vi "CRYLimits Editor.vi"(6 "Channel":i32=1, 8 "Calibration In":string, 9 "Hardware In":string, 10 "Set up in":string) -> (2 "Set up Out":string)   [LabVIEW 2013]
uses:
  <vilib>/Utility/miscctls.llb/LVBoundsTypeDef.ctl
  Typedef Control/CRYLimits.ctl
  Typedef Control/CRYWaveform Cluster.ctl
  Typedef Control/CRYData Cluster.ctl
  <vilib>/Utility/miscctls.llb/LVRowAndColumnTypeDef.ctl
  <vilib>/Utility/miscctls.llb/LVRowAndColumnUnsignedTypeDef.ctl
  CRYLimit edit global.vi
  CRYProject/CRYProject Editor Global.vi
  CRYWindow/SubVI/CRYMain Sub Window Global.vi
  CRYMainGlobal.vi
  CRYStepSetup/CRYStepSetup Global.vi
panel:
  in  "RawLo Limit":dbl caption="酒贰茄拌" format="%.2p"
  in  "RawUp Limit":dbl caption="眶茄拌" format="%.2p"
  out "Limit Cluster Bk":T1={"Name"="", "Tolerance"=2, "X Axis"=1, "Limits"=2, "Upper Limit"=[{100.0, 1.0}, {1000.0, 1.0}], "Align Ref"={1000.0, 0.0}, "Lower Limit"=[{100.0, -1.0}, {1000.0, -1.0}], "Y data"=1, "Y unit"="(und)", "Y dB ref"=1.0, "Curve Names"=[], "Y-Resolution"=1, "Type"=1, "x float"=FALSE, "X min-max-step"={"Limit X Offset Min"=0.9, "Limit X Offset Max"=1.1, "Limit X Offset Step Size"=1.01}, "magn/phase"=1, "Upper Limit Type"=0, "Lower Limit Type"=0, "Lim Curve axis up"=1, "Lim Curve axis lo"=1, "Data Selection Upper"=1, "Data Selection Lower"=1, "X-Resolution"=1, "Output failed point curves?"=FALSE, "X data"=1, "X unit"="(und)", "X dB ref"=1.0, "X-Y Graph Set-up"="", "Tab Value"=enum."Parameters", "Help"="", "X Up Val"=0.0, "Y Up Val"=0.0, "X Low Val"=0.0, "Y Low Val"=0.0, "Up Limit Val"=0.0, "Low Limit Val"=0.0, "bAdd DataName"=FALSE, "Custom Name"=""} {"X data" items=["dB", "Lin"]; "Data Selection Lower" items=["Single Values", "Curves", "Waveforms"]; "Data Selection Upper" items=["Single Values", "Curves", "Waveforms"]; "Lim Curve axis lo" items=["x", "y", "z"]; "Lim Curve axis up" items=["x", "y", "z"]; "Lower Limit Type" items=["User Defined", "Memory List"]; "Upper Limit Type" items=["User Defined", "Memory List"]; "Type" items=["Single Value", "Curve", "Waveforms", "Voltmeter"]; "Y data" items=["dB", "Lin"]; "Limits" items=["Upper Only", "Lower Only", "Upper & Lower"]; "X Axis" items=["Linear", "Logarithmic"]; "Tolerance" items=["Individual Points", "Absolute Limits", "Floating Limits", "Floating Data", "Aligned Limits", "Aligned Data"]}
  out "Raw DataVal":dbl format="%.2p"
  in  "CurLibChange":bool caption="Add Lib"
  out "MinMaxXrange":bool
  out "Lo_oldx":dbl
  out "Up_oldx":dbl
  out "cursor move":bool
  out "Wave":T2={"Waveform"={"X0"=0.0, "dX"=0.0, "Y"=[]}, "X data"=1, "Y data"=1, "Y axis"=1, "X unit"="s", "Y unit"="V", "Y dB ref"=1.0, "display Y"=TRUE, "display X"=TRUE, "Overload?"=FALSE, "Test Info"="", "Step No."=0, "Name"="", "protected"=FALSE, "Sqc history"=[], "Signal Channel ID"=0, "Plot Settings"={"Color"=0, "Interpolation"=0, "Point Style"=0, "Line Style"=0, "Point Color"=0, "Line Width"=0, "Bar Plot Style"=0, "Fill To"=0}, "AutoProtect"=FALSE} {"Y dB ref" format="%.1f"; "Y axis" items=["Log", "Lin"]; "Y data" items=["dB", "Lin"]; "X data" items=["dB", "Lin"]}
  out "EndFlag":bool
  in  "Add Lib":bool
  in  "AddStep":bool
  in  "Load state":bool
  out "Lo Curve and Values":T3={"Name"="", "Curve"=[], "X data"=1, "Y data"=1, "Z data"=1, "X axis"=0, "Y axis"=1, "Z axis"=1, "X unit"="Hz", "Y unit"="", "Z unit"="deg.", "X dB ref"=1.0, "Y dB ref"=1.0, "Z dB ref"=1.0, "single val"=FALSE, "protected"=FALSE, "display X"=TRUE, "display Y"=TRUE, "display Z"=TRUE, "Test Info"="", "Step No."=0, "Plot Settings"={"Color"=0, "Interpolation"=0, "Point Style"=0, "Line Style"=0, "Point Color"=0, "Line Width"=0, "Bar Plot Style"=0, "Fill To"=0}, "AutoProtect"=FALSE} {"Z data" items=["dB", "Lin"]; "X data" items=["dB", "Lin"]; "Y data" items=["dB", "Lin"]; "Z dB ref" format="%.1f"; "Z axis" items=["Log", "Lin"]; "X dB ref" format="%.1f"; "X axis" items=["Log", "Lin"]; "Y axis" items=["Log", "Lin"]; "Y dB ref" format="%.1f"; "Curve"."z" format="%.2f"; "Curve"."y" format="%.2f"; "Curve"."x" format="%.2f"}
  out "Up Curve and Value":T3={"Name"="", "Curve"=[], "X data"=1, "Y data"=1, "Z data"=1, "X axis"=0, "Y axis"=1, "Z axis"=1, "X unit"="Hz", "Y unit"="", "Z unit"="deg.", "X dB ref"=1.0, "Y dB ref"=1.0, "Z dB ref"=1.0, "single val"=FALSE, "protected"=FALSE, "display X"=TRUE, "display Y"=TRUE, "display Z"=TRUE, "Test Info"="", "Step No."=0, "Plot Settings"={"Color"=0, "Interpolation"=0, "Point Style"=0, "Line Style"=0, "Point Color"=0, "Line Width"=0, "Bar Plot Style"=0, "Fill To"=0}, "AutoProtect"=FALSE} {"Z data" items=["dB", "Lin"]; "X data" items=["dB", "Lin"]; "Y data" items=["dB", "Lin"]; "Z dB ref" format="%.1f"; "Z axis" items=["Log", "Lin"]; "X dB ref" format="%.1f"; "X axis" items=["Log", "Lin"]; "Y axis" items=["Log", "Lin"]; "Y dB ref" format="%.1f"; "Curve"."z" format="%.2f"; "Curve"."y" format="%.2f"; "Curve"."x" format="%.2f"}
  out "Curve and Value":T3={"Name"="", "Curve"=[], "X data"=1, "Y data"=1, "Z data"=1, "X axis"=0, "Y axis"=1, "Z axis"=1, "X unit"="Hz", "Y unit"="", "Z unit"="deg.", "X dB ref"=1.0, "Y dB ref"=1.0, "Z dB ref"=1.0, "single val"=FALSE, "protected"=FALSE, "display X"=TRUE, "display Y"=TRUE, "display Z"=TRUE, "Test Info"="", "Step No."=0, "Plot Settings"={"Color"=0, "Interpolation"=0, "Point Style"=0, "Line Style"=0, "Point Color"=0, "Line Width"=0, "Bar Plot Style"=0, "Fill To"=0}, "AutoProtect"=FALSE} {"Z data" items=["dB", "Lin"]; "X data" items=["dB", "Lin"]; "Y data" items=["dB", "Lin"]; "Z dB ref" format="%.1f"; "Z axis" items=["Log", "Lin"]; "X dB ref" format="%.1f"; "X axis" items=["Log", "Lin"]; "Y axis" items=["Log", "Lin"]; "Y dB ref" format="%.1f"; "Curve"."z" format="%.2f"; "Curve"."y" format="%.2f"; "Curve"."x" format="%.2f"}
  in  "Plot Multilimit":bool
  out "Lo Wave":T2={"Waveform"={"X0"=0.0, "dX"=0.0, "Y"=[]}, "X data"=1, "Y data"=1, "Y axis"=1, "X unit"="s", "Y unit"="V", "Y dB ref"=1.0, "display Y"=TRUE, "display X"=TRUE, "Overload?"=FALSE, "Test Info"="", "Step No."=0, "Name"="", "protected"=FALSE, "Sqc history"=[], "Signal Channel ID"=0, "Plot Settings"={"Color"=0, "Interpolation"=0, "Point Style"=0, "Line Style"=0, "Point Color"=0, "Line Width"=0, "Bar Plot Style"=0, "Fill To"=0}, "AutoProtect"=FALSE} {"Y dB ref" format="%.1f"; "Y axis" items=["Log", "Lin"]; "Y data" items=["dB", "Lin"]; "X data" items=["dB", "Lin"]}
  out "Up Wave":T2={"Waveform"={"X0"=0.0, "dX"=0.0, "Y"=[]}, "X data"=1, "Y data"=1, "Y axis"=1, "X unit"="s", "Y unit"="V", "Y dB ref"=1.0, "display Y"=TRUE, "display X"=TRUE, "Overload?"=FALSE, "Test Info"="", "Step No."=0, "Name"="", "protected"=FALSE, "Sqc history"=[], "Signal Channel ID"=0, "Plot Settings"={"Color"=0, "Interpolation"=0, "Point Style"=0, "Line Style"=0, "Point Color"=0, "Line Width"=0, "Bar Plot Style"=0, "Fill To"=0}, "AutoProtect"=FALSE} {"Y dB ref" format="%.1f"; "Y axis" items=["Log", "Lin"]; "Y data" items=["dB", "Lin"]; "X data" items=["dB", "Lin"]}
  out "Lo Limit Data":cluster{"x":dbl, "y":dbl}[](array[cluster])
  out "Up Limit Data":cluster{"x":dbl, "y":dbl}[](array[cluster])
  in  "Plot graphs":bool
  out "Limit Cluster":T1={"Name"="", "Tolerance"=2, "X Axis"=1, "Limits"=2, "Upper Limit"=[{100.0, 1.0}, {1000.0, 1.0}], "Align Ref"={1000.0, 0.0}, "Lower Limit"=[{100.0, -1.0}, {1000.0, -1.0}], "Y data"=1, "Y unit"="(und)", "Y dB ref"=1.0, "Curve Names"=[], "Y-Resolution"=1, "Type"=1, "x float"=FALSE, "X min-max-step"={"Limit X Offset Min"=0.9, "Limit X Offset Max"=1.1, "Limit X Offset Step Size"=1.01}, "magn/phase"=1, "Upper Limit Type"=0, "Lower Limit Type"=0, "Lim Curve axis up"=1, "Lim Curve axis lo"=1, "Data Selection Upper"=1, "Data Selection Lower"=1, "X-Resolution"=1, "Output failed point curves?"=FALSE, "X data"=1, "X unit"="(und)", "X dB ref"=1.0, "X-Y Graph Set-up"="", "Tab Value"=enum."Parameters", "Help"="", "X Up Val"=0.0, "Y Up Val"=0.0, "X Low Val"=0.0, "Y Low Val"=0.0, "Up Limit Val"=0.0, "Low Limit Val"=0.0, "bAdd DataName"=FALSE, "Custom Name"=""} {"X data" items=["dB", "Lin"]; "Data Selection Lower" items=["Single Values", "Curves", "Waveforms"]; "Data Selection Upper" items=["Single Values", "Curves", "Waveforms"]; "Lim Curve axis lo" items=["x", "y", "z"]; "Lim Curve axis up" items=["x", "y", "z"]; "Lower Limit Type" items=["User Defined", "Memory List"]; "Upper Limit Type" items=["User Defined", "Memory List"]; "Type" items=["Single Value", "Curve", "Waveforms", "Voltmeter"]; "Y data" items=["dB", "Lin"]; "Limits" items=["Upper Only", "Lower Only", "Upper & Lower"]; "X Axis" items=["Linear", "Logarithmic"]; "Tolerance" items=["Individual Points", "Absolute Limits", "Floating Limits", "Floating Data", "Aligned Limits", "Aligned Data"]}
  in  "Load Test":bool
  out "VIMiniumBound":T4
  out "Proper VI No":i32
  in  "stop":bool
  out "Point index":i32
  out "Plot index":i32
  in  "Board Tab":enum32{"Page 1", "Page 2"}(tab)
  in  "Cancel":bool caption="Apply"
  in  "OK":bool caption="Apply"
  out "Lo tip":string="(und)"
  out "Up tip":string="(und)"
  in  "Single Limit":dbl(slide)=100.0 caption="Upper limit" scale=-0.1..1.0999999999999999 scale format="%#.3p"
  out "tolerance":string="(und)"
  out "Margin":dbl caption="边缘" format="%.0p"
  out "Verdict":bool=TRUE
  out "Multi unit":string="(und)"
  in  "Multi Limit":cluster{dbl, dbl}(slide)={100.0, 4.285714285714286} caption="Upper limit" scale=-0.1..1.0999999999999999 scale format="%#.3p"
  out "Multi value":dbl(slide) scale=-0.1..1.0999999999999999 scale format="%.1p"
  in  "Main Tab":enum32{"Data", "Parameters", "Help"}(tab)
  in  "bAdd DataName":bool caption="Add Input Data Name"
  in  "Custom Name":string caption="Custom Result Name"
  out "Data":bool
  in  "LoSource":u16(slide)=1 caption="Source"
  in  "UpSource":u16(slide)=1 caption="Source"
  in  "Type":u16(slide)=1
  out "Lower Limit":bool
  in  "Sub2 Tab":enum32{"Page 1"}(tab)
  out "Upper Limit Offset":bool
  in  "X Up Val":dbl caption="X" format="%#.3p"
  in  "Y Up Val":dbl caption="Y" format="%#.3p"
  in  "Upp x Unit":u16(ring) items=["s", "%"]
  in  "Upp y Unit":u16(ring) items=["V", "%"]
  in  "Offset Upper":bool
  in  "Insert Upper":bool
  in  "Delete Upper":bool
  in  "Sub3 Tab":enum32{"Page 1"}(tab)
  in  "Delete Lower":bool
  in  "Insert Lower":bool
  in  "Offset Lower":bool
  in  "Low x Unit":u16(ring) items=["s", "%"]
  in  "Low y Unit":u16(ring) items=["dB", "%"]
  in  "X Lo Val":dbl caption="X" format="%#.3p"
  in  "Y Lo Val":dbl caption="Y" format="%#.3p"
  out "Lower Limit Offset":bool
  in  "Sub5 Tab":enum32{"Page 1"}(tab)
  in  "LoTable_1":string[][](table)=[["100", "1000"], ["1.0", "1.0"]]
  in  "Clear Lower":bool
  in  "copy Lower":bool
  in  "Lo Limit Val":dbl caption="Lower Limit" format="%.0p"
  out "lo single unit":string="(und)"
  out "LowAlignRst_1":string="(und)"
  in  "Sub7 Tab":enum32{"Page 1"}(tab)
  in  "Lo_xyz":u16(slide) scale=0.0..2.0
  in  "Lo Cur Name":u16(ring) items=["unity cal-in sens-in", "CRY33x Mic 1 sens-in", "CRY33x Mic 2 sens-in", "CRY33x Mic 3 sens-in", "CRY33x Mic 4 sens-in", "USB In L sens-in", "USB In R sens-in", "unity cal-out sens-out", "CRY602 Mouth 1 sens-out", "CRY602 Mouth 2 sens-out", "USB Out R sens-out", "Max FSD Out Stimulus", "采集延迟 [Direct Out 1] - P"]
  out "LoSingleVal":dbl format="%.1p"
  out "low_unit":string="(und)"
  out "LoTable_2":string[][](table)=[["100", "1000"], ["1.0", "1.0"]]
  in  "Lo_type":enum32{"Single Values", "Curves", "Waveforms"}(radio) caption="Type"
  out "LowAlignRst_2":string="(und)"
  in  "Sub4 Tab":enum32{"Page 1"}(tab)
  in  "copy Upper":bool
  in  "UpTable_1":string[][](table)
  in  "Clear Upper":bool
  in  "Up Limit Val":dbl caption="Upper Limit" format="%.1p"
  out "UpAlignRst_1":string="(und)"
  out "up single unit":string="(und)"
  out "Upper Limit":bool
  in  "Sub6 Tab":enum32{"Page 1"}(tab)
  in  "Up_xyz":u16(slide) scale=0.0..2.0
  out "UpSingleVal":dbl format="%.1p"
  in  "Up Cur Name":u16(ring) items=["unity cal-in sens-in", "CRY33x Mic 1 sens-in", "CRY33x Mic 2 sens-in", "CRY33x Mic 3 sens-in", "CRY33x Mic 4 sens-in", "USB In L sens-in", "USB In R sens-in", "unity cal-out sens-out", "CRY602 Mouth 1 sens-out", "CRY602 Mouth 2 sens-out", "USB Out R sens-out", "Max FSD Out Stimulus", "采集延迟 [Direct Out 1] - P"]
  out "up_unit":string="(und)"
  out "UpTable_2":string[][](table)=[["100", "1000"], ["-1.0", "-1.0"]]
  in  "Up_type":enum32{"Single Values", "Curves", "Waveforms"}(radio) caption="Type"
  out "UpAlignRst_2":string="(und)"
  in  "Data Name":u16(ring) items=["Stimulus", "Stimulus - P", "2-Stimulus - P", "3-Stimulus - P"]
  in  "Sub1 Tab":enum32{"Page 1"}(tab)
  out "Data Value":dbl format="%.1p"
  in  "Data_xyz":u16(slide) scale=0.0..2.0
  out "data unit":string="(und)"
  out "Data Table":string[][](table)=[["100", "1000"], ["-1.0", "-1.0"]]
  out "DataAlignRst":string="(und)"
  out "y-axis":bool
  out "x-axis":bool
  out "size_unit":string="(und)"
  in  "Step Size":dbl=2.0 min=1.0001 step=0.01 format="%#.3p"
  in  "X AlignRef":dbl=1000.0 caption="Alignment Reference" format="%#.3p"
  in  "X Resolution":u8=1 caption="Absolute Comparison Precision" format="%01.0f"
  in  "x float":bool caption="Float limits"
  in  "Maximum":dbl=10.000000000000009 step=0.01 format="%#.3p"
  in  "Minimum":dbl=1.0 step=0.01 format="%#.3p"
  in  "Y AlignRef":dbl caption="Alignment Reference" format="%#.3p"
  in  "Y Resolution":u8=1 caption="Absolute Comparison Precision"
  out "Limits Parameters":bool
  in  "Out Fail":bool caption="Output Failed"
  in  "Mapping":u16(slide)=1
  in  "Alignment":u16(ring) items=["Individual Points", "Absolute Limits", "Floating Limits", "Floating Data", "Aligned Limits", "Aligned Data"]
  in  "Limits_Ring":u16(ring) caption="Limits" items=["Upper Only", "Lower Only", "Upper & Lower"]
  in  "Help":string
  in  "Appy limits":bool
  out "Limits Graph":cluster{"element":cluster{"x":dbl, "y":dbl}[]}[](graph)
  in  "Load...":bool caption="Apply"
  in  "Revert":bool caption="Apply"
  in  "Save As...":bool caption="Apply"
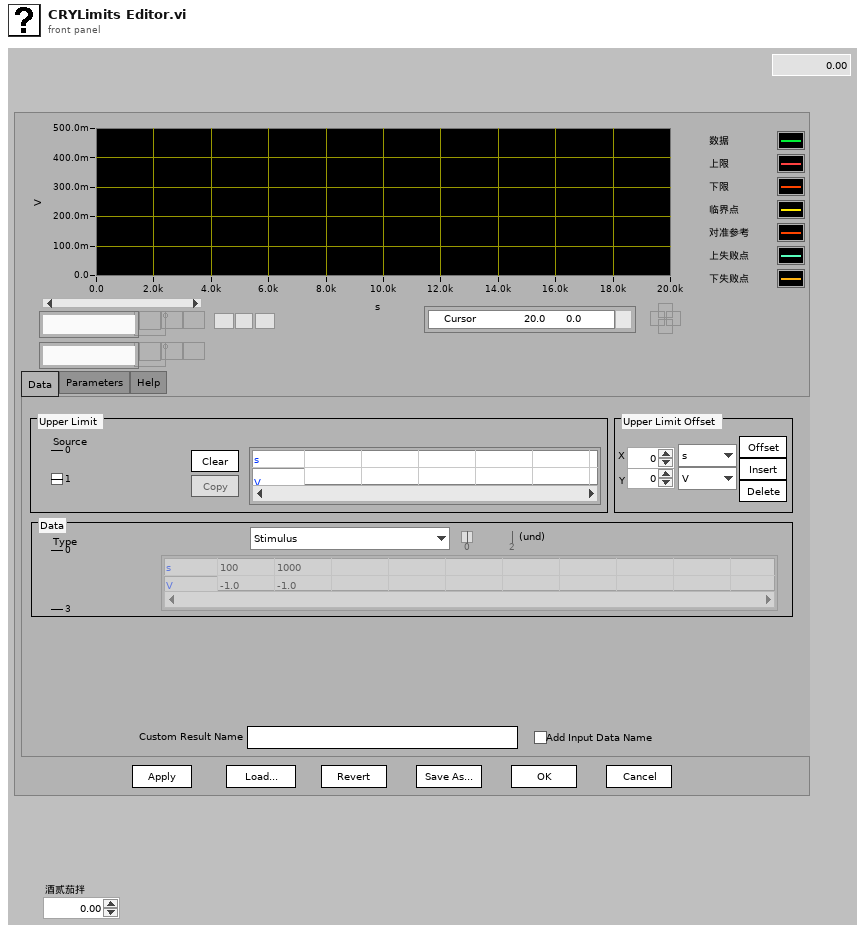
[diagram p1: front panel]
types:
  T1 = typedef "CRYLimits.ctl" = cluster{"Name":string, "Tolerance":u16, "X Axis":u16, "Limits":u16, "Upper Limit":cluster{dbl, dbl}[], "Align Ref":cluster{dbl, dbl}, "Lower Limit":cluster{dbl, dbl}[], "Y data":u16, "Y unit":string, "Y dB ref":dbl, "Curve Names":string[], "Y-Resolution":u8, "Type":u16, "x float":bool, "X min-max-step":cluster{"Limit X Offset Min":dbl, "Limit X Offset Max":dbl, "Limit X Offset Step Size":dbl}, "magn/phase":u16, "Upper Limit Type":u16, "Lower Limit Type":u16, "Lim Curve axis up":u16, "Lim Curve axis lo":u16, "Data Selection Upper":u16, "Data Selection Lower":u16, "X-Resolution":u8, "Output failed point curves?":bool, "X data":u16, "X unit":string, "X dB ref":dbl, "X-Y Graph Set-up":string, "Tab Value":enum32{"Data", "Parameters"}, "Help":string, "X Up Val":dbl, "Y Up Val":dbl, "X Low Val":dbl, "Y Low Val":dbl, "Up Limit Val":dbl, "Low Limit Val":dbl, "bAdd DataName":bool, "Custom Name":string}
  T2 = typedef "CRYWaveform Cluster.ctl" = cluster{"Waveform":cluster{"X0":dbl, "dX":dbl, "Y":sgl[]}, "X data":u16, "Y data":u16, "Y axis":u16, "X unit":string, "Y unit":string, "Y dB ref":dbl, "display Y":bool, "display X":bool, "Overload?":bool, "Test Info":string, "Step No.":i32, "Name":string, "protected":bool, "Sqc history":string[], "Signal Channel ID":i32, "Plot Settings":cluster{"Color":u32, "Interpolation":u8, "Point Style":u8, "Line Style":u8, "Point Color":u32, "Line Width":u8, "Bar Plot Style":u8, "Fill To":i16}, "AutoProtect":bool}
  T3 = typedef "CRYData Cluster.ctl" = cluster{"Name":string, "Curve":cluster{"x":dbl, "y":dbl, "z":dbl}[], "X data":u16, "Y data":u16, "Z data":u16, "X axis":u16, "Y axis":u16, "Z axis":u16, "X unit":string, "Y unit":string, "Z unit":string, "X dB ref":dbl, "Y dB ref":dbl, "Z dB ref":dbl, "single val":bool, "protected":bool, "display X":bool, "display Y":bool, "display Z":bool, "Test Info":string, "Step No.":i32, "Plot Settings":cluster{"Color":u32, "Interpolation":u8, "Point Style":u8, "Line Style":u8, "Point Color":u32, "Line Width":u8, "Bar Plot Style":u8, "Fill To":i16}, "AutoProtect":bool}
  T4 = typedef "LVBoundsTypeDef.ctl" = cluster{"Width":u32, "Height":u32}
  T5 = typedef "LVRowAndColumnTypeDef.ctl" = cluster{"Row":i32, "Column":i32}
  T6 = typedef "LVPositionTypeDef.ctl" = cluster{"Left":i32, "Top":i32}
  T7 = typedef "CRYStep.ctl" = cluster{"No.VI":i32, "Category":string, "StepName":string, "Seq setup flattened":string, "Comment":string, "Steps config.":bool[], "Jump config":i32[], "Start":dbl, "Increment":dbl, "Name":string, "Unit":string, "Y data":u16, "Y prefix":string, "Y dB ref":dbl, "Y unit":string, "Repeat State Array":cluster{"Start":dbl, "Increment":dbl, "Count":i32, "Num":i32}[]}
  T8 = typedef "LVRowAndColumnUnsignedTypeDef.ctl" = cluster{"Row":u32, "Column":u32}
  T9 = enum16{"OK", "Yes", "YesNo", "YesNoCancel", "ReplaceAppend"}
  T10 = typedef "LVPoint32TypeDef.ctl" = cluster{"Horizontal":i32, "Vertical":i32}
  T11 = typedef "LVRectTypeDef.ctl" = cluster{"Left":i16, "Top":i16, "Right":i16, "Bottom":i16}
  T12 = typedef "LVRangeTypeDef.ctl" = cluster{"Minimum":dbl, "Maximum":dbl, "Increment":dbl, "Minor Increment":dbl, "Start":dbl}
  T13 = typedef "CRYData Cluster Array.ctl" = T3[]
  T14 = typedef "CRYWaveform Cluster Array.ctl" = T2[]
  T15 = cluster{"Limit X Offset Min":dbl, "Limit X Offset Max":dbl, "Limit X Offset Step Size":dbl}
  T16 = cluster{"Appy limits":bool, "Load Test":bool, "Plot graphs":bool, "Plot Multilimit":bool, "Add Lib":bool, "OK":bool, "Cancel":bool}
  T17 = typedef "CRYResult Cluster.ctl" = cluster{"Name":string, "Margin":dbl, "unit":string, "Verdict":bool, "Limit":string, "Max/Min":string, "protected":bool, "Step No.":i32, "Test Info":string, "AutoProtect":bool}
  T18 = cluster{"Lower Failed":cluster{"Numeric":dbl, "Numeric 2":dbl}[]}[]
  T19 = cluster{"Lower Failed":cluster{"Numeric":dbl, "Numeric 2":dbl}[]}
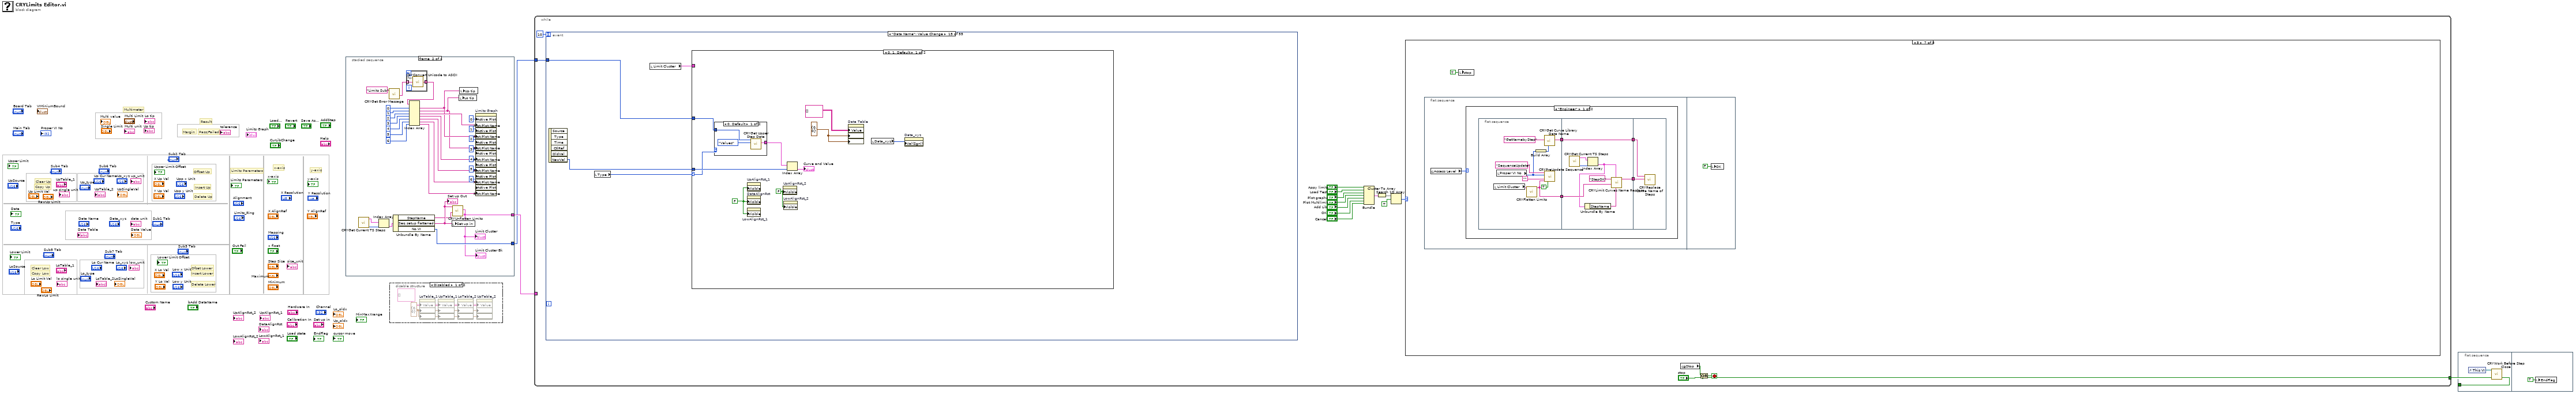
[diagram p0: block diagram]
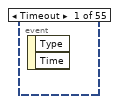
[diagram p3: hidden frame]
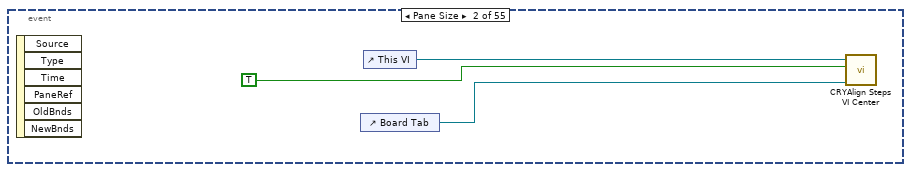
[diagram p4: hidden frame]
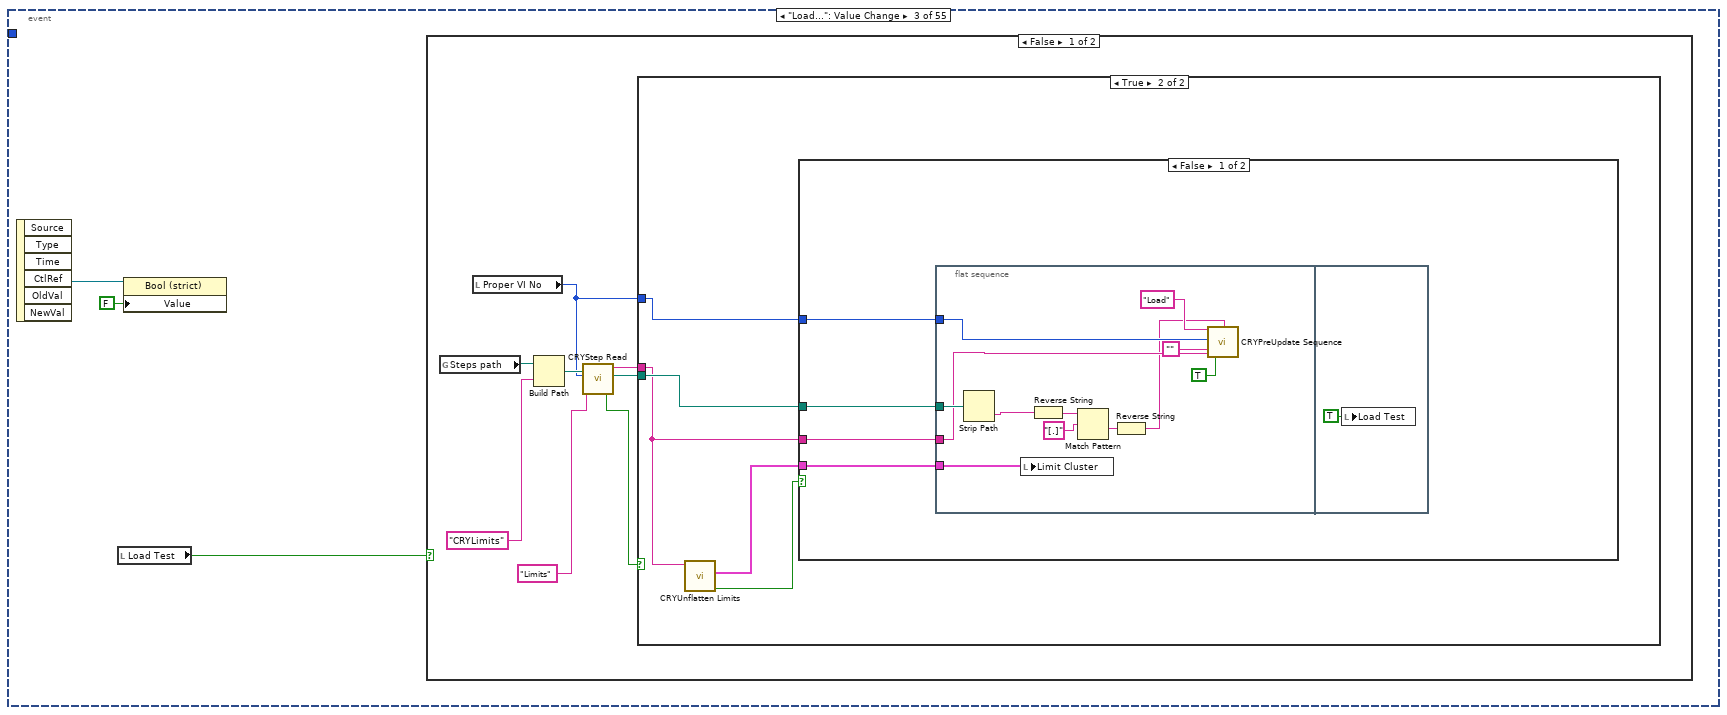
[diagram p5: hidden frame]
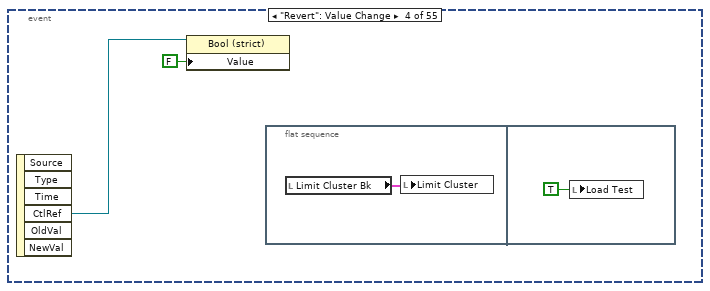
[diagram p9: hidden frame]
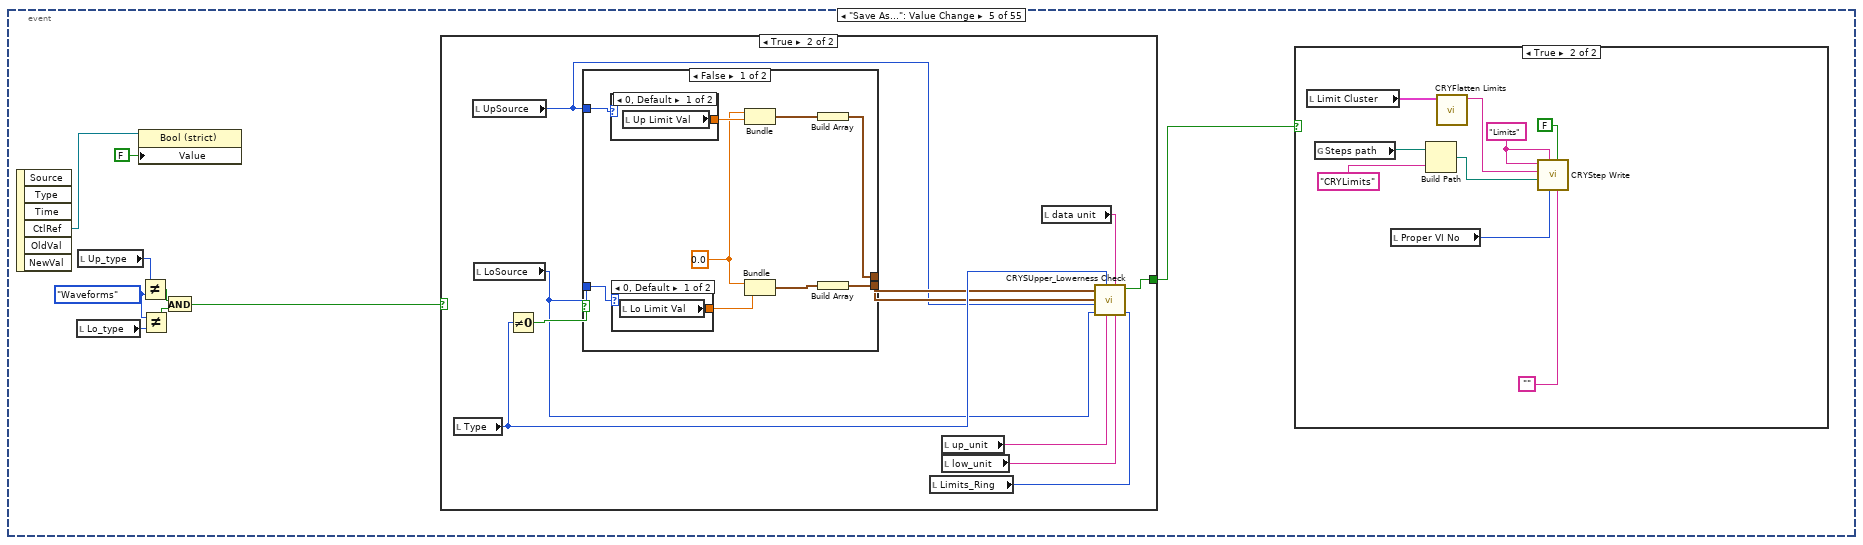
[diagram p10: hidden frame]
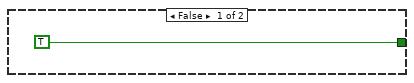
[diagram p11: hidden frame]
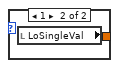
[diagram p12: hidden frame]
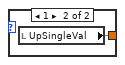
[diagram p13: hidden frame]
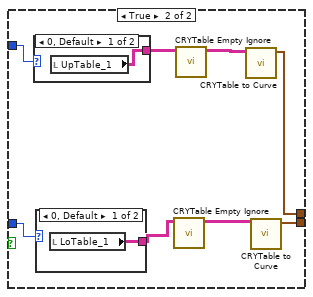
[diagram p14: hidden frame]
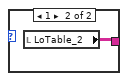
[diagram p15: hidden frame]
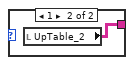
[diagram p16: hidden frame]
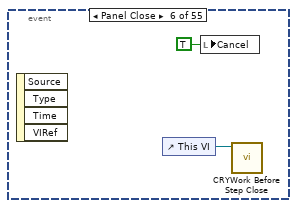
[diagram p18: hidden frame]
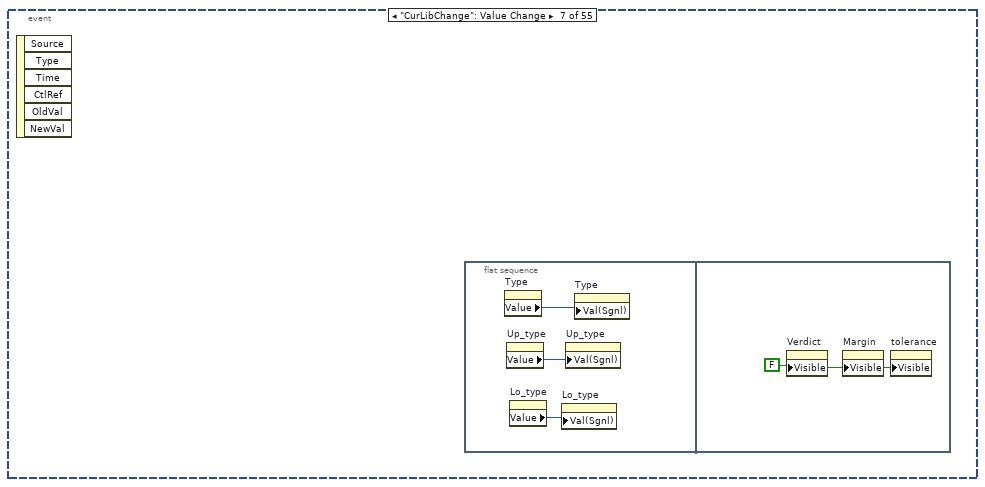
[diagram p19: hidden frame]
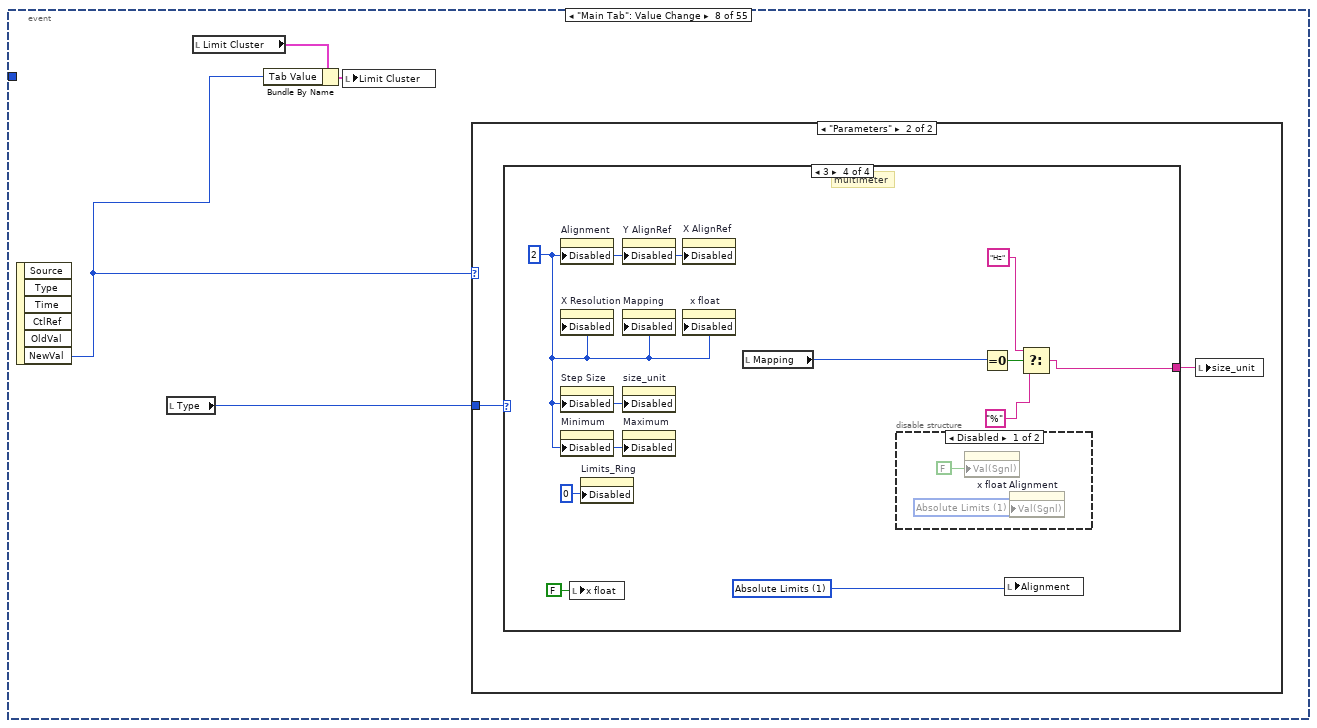
[diagram p20: hidden frame]
diagram:
  # "Pass/Failed"
  # "Margin"
  # "Copy Low"
  # "Clear Low"
  # "Copy Up"
  # "Clear Up"
  # "Delete Lower"
  # "Delete Up"
  # "Insert Lower"
  # "Insert Up"
  # "Ofset Lower"
  # "Offset Up"
  # "Result"
  # "Multimeter"
  # "y-axis"
  # "x-axis"
  # "Limits Parameters"
  n1 = stacked-sequence {
    tunnel: [_ w20 _ _] -> w3
    tunnel: [_ w21 _ _] -> w1
    frame #0 {
      w5 = T5 {"Row"=0, "Column"=0} ("Selection Start")
      w6 = cluster{dbl, dbl}[] [] ("critical point")
      w10 = FALSE ("Plot.Visible")
      w4 = FALSE ("Visible")
      n2 = property on="Board Tab" class="TabCtl (strict)"("Visible"=w4) -> ()  [unwired: 2 in, 2 out]
      n3 = property on="Margin" class="DigNum (strict)"("Visible"=w4) -> ()  [unwired: 2 in, 2 out]
      n4 = property on="Verdict" class="Bool (strict)"("Visible"=w4) -> ()  [unwired: 2 in, 2 out]
      n5 = property on="tolerance" class="Str"("Visible"=w4) -> ()  [unwired: 2 in, 2 out]
      n6 = local write "stop"(w4) -> ()
      n7 = local write "EndFlag"(w4) -> ()
      n8 = property on="Board Tab" class="TabCtl (strict)"() -> ("Width"=w17:u32, "Height"=w18:u32)  [unwired: 2 in, 2 out]
      n9 = global read "CRYProject Editor Global.vi" "Step Setup VI No"() -> (w14:i32)
      n10 = property on="LoTable_1" class="Tbl (strict)"("Index Values"=w5) -> ()  [unwired: 2 in, 2 out]
      n11 = property on="Multi value" class="Slide (strict)"() -> (error out=w9:errorcluster, "Housing Size"=w8:T4)  [unwired: 2 in, 1 out]
      n12 = Bundle By Name(cluster=T4 {"Width"=0, "Height"=0} ("VIMiniumBound"), "Width"=w17, "Height"=w18) -> (w16:T4)
      n13 = property on="UpTable_1" class="Tbl (strict)"("Index Values"=w5) -> ()  [unwired: 2 in, 2 out]
      n14 = local write "Proper VI No"(w14) -> ()
      n15 = local write "VIMiniumBound"(w16) -> ()
      n16 = property on="Multi Limit" class="Slide (strict)"(error in=w9, "Housing Size"=w8) -> ("Position"=w7:T6)  [unwired: 1 in, 2 out]
      n17 = property on="Single Limit" class="Slide (strict)"("Housing Size"=w8, "Position"=w7) -> ()  [unwired: 2 in, 2 out]
      n18 = property on="LoTable_2" class="Tbl (strict)"("Index Values"=w5) -> ()  [unwired: 2 in, 2 out]
      n19 = property on="Limits Graph" class="XYGraph (strict)"("Active Plot"=u32 4, "Plot.Visible?"=w10, "Active Plot"=u32 5, "Plot.Visible?"=w10, "Active Plot"=u32 6, "Plot.Visible?"=w10) -> ()  [unwired: 2 in, 2 out]
      n20 = global write "CRYLimit edit global.vi" "critical point"(w6) -> ()
      n21 = global write "CRYLimit edit global.vi" "align ref point"(w6) -> ()
      n22 = global write "CRYLimit edit global.vi" "Upper Failed"(w6) -> ()
      n23 = global write "CRYLimit edit global.vi" "Lower Failed"(w6) -> ()
      n24 = property on="UpTable_2" class="Tbl (strict)"("Index Values"=w5) -> ()  [unwired: 2 in, 2 out]
      n25 = property on="Data Table" class="Tbl (strict)"("Index Values"=w5) -> ()  [unwired: 2 in, 2 out]
    }
    frame #1 {
      n26 = call "CRYGet Current TS Steps.vi"() -> ("SelectStepNumber in Tree"=w46:i32, "Steps"=w47:T7[])  [unwired: 7 in, 3 out]
      n27 = Index Array(array=w47, index=w46) -> (element=w49:T7)
      n28 = call "CRYGet Error Message.vi"("Kind"="Limits Sub") -> ("Unicode Message Sub"=w23:string[])  [unwired: 5 in, 5 out]
      n29 = Unbundle By Name(w49) -> ("StepName"=w19:string, "Seq setup flattened"=w48:string, "No.VI"=w21:i32)
      "Set up Out" <- w48
      n30 = for {
        tunnel: w23 -> [w51] mode=indexing
        tunnel: [w50] -> w22 mode=indexing
        n31 = call "CRYConvert Unicode to ASCII.vi"("Unicode"=w51) -> ("ASCII"=w50:string)  [unwired: 4 in]
      }
      n32 = Index Array(array=w22, index #1=0 ("index"), index #2=1 ("index"), index #3=2 ("index"), index #4=3 ("index"), index #5=4 ("index"), index #6=5 ("index"), index #7=6 ("index")) -> (element #1=w29:string, element #2=w28:string, element #3=w30:string, element #4=w27:string, element #5=w26:string, element #6=w25:string, element #7=w24:string)
      n33 = local write "Set up in"(w48) -> ()
      n34 = call "CRYUnflatten Limits.vi"("Step Name"=w19, "Unflatten Limits"=w48) -> ("Limits"=w20:T1)  [unwired: 9 out]
      "Limit Cluster" <- w20
      "Limit Cluster Bk" <- w20
      n35 = local write "Lo tip"(w28) -> ()
      n36 = local write "Up tip"(w29) -> ()
      n37 = property on="Limits Graph" class="XYGraph (strict)"("Active Plot"=u32 0, "Plot.Plot Name"=w30, "Active Plot"=u32 1, "Plot.Plot Name"=w29, "Active Plot"=u32 2, "Plot.Plot Name"=w28, "Active Plot"=u32 3, "Plot.Plot Name"=w27, "Active Plot"=u32 4, "Plot.Plot Name"=w26, "Active Plot"=u32 5, "Plot.Plot Name"=w25, "Active Plot"=u32 6, "Plot.Plot Name"=w24) -> ()  [unwired: 2 in, 2 out]
    }
    frame #2 {
      w54 = FALSE ("Visible")
      w52 = u32 16744448
      w61 = 100 ("Numeric")
      n38 = local write "Plot Multilimit"(FALSE ("Plot graphs")) -> ()
      n39 = local write "cursor move"(FALSE ("cursor move")) -> ()
      n40 = control-ref of="UpTable_1"() -> (w65:refnum<vi>)
      n41 = local write "Plot graphs"(FALSE ("Plot graphs")) -> ()
      n42 = control-ref of="LoTable_1"() -> (w64:refnum<vi>)
      n43 = control-ref of="UpTable_2"() -> (w63:refnum<vi>)
      n44 = property on="Board Tab" class="TabCtl (strict)"("Visible"=FALSE) -> ()  [unwired: 2 in, 2 out]
      n45 = control-ref of="LoTable_2"() -> (w62:refnum<vi>)
      n46 = control-ref of="Data Table"() -> (w66:refnum<vi>)
      n47 = call "CRYSet table cell size.vi"("Colum size"=w61, "Table"=w64) -> ()  [unwired: 10 out]
      n48 = call "CRYSet table cell size.vi"("Colum size"=w61, "Table"=w63) -> ()  [unwired: 10 out]
      n49 = call "CRYSet table cell size.vi"("Colum size"=w61, "Table"=w65) -> ()  [unwired: 10 out]
      n50 = call "CRYSet table cell size.vi"("Colum size"=w61, "Table"=w62) -> ()  [unwired: 10 out]
      n51 = call "CRYSet table cell size.vi"("Colum size"=w61, "Table"=w66) -> ()  [unwired: 10 out]
      n52 = property on="DataAlignRst" class="Str"("Visible"=w54) -> ()  [unwired: 2 in, 2 out]
      n53 = property on="LowAlignRst_1" class="Str"("Visible"=w54) -> ()  [unwired: 2 in, 2 out]
      n54 = property on="UpAlignRst_1" class="Str"("Visible"=w54) -> ()  [unwired: 2 in, 2 out]
      n55 = property on="UpAlignRst_2" class="Str"("Visible"=w54) -> ()  [unwired: 2 in, 2 out]
      n56 = property on="LowAlignRst_2" class="Str"("Visible"=w54) -> ()  [unwired: 2 in, 2 out]
      n57 = call "CRYGet Error Message.vi"("Error No"=7, "Kind"="Limits") -> ("Message"=w53:string)  [unwired: 4 in, 5 out]
      n58 = property on="LowAlignRst_1" class="Str"("Text.TextColor"=w52, "Text.Text"=w53) -> ()  [unwired: 2 in, 2 out]
      n59 = property on="UpAlignRst_2" class="Str"("Text.TextColor"=w52, "Text.Text"=w53) -> ()  [unwired: 2 in, 2 out]
      n60 = property on="LowAlignRst_2" class="Str"("Text.TextColor"=w52, "Text.Text"=w53) -> ()  [unwired: 2 in, 2 out]
      n61 = property on="UpAlignRst_1" class="Str"("Text.TextColor"=w52, "Text.Text"=w53) -> ()  [unwired: 2 in, 2 out]
      n62 = property on="DataAlignRst" class="Str"("Text.TextColor"=w52, "Text.Text"=w53) -> ()  [unwired: 2 in, 2 out]
    }
    frame #3 {
      n63 = local write "Load Test"(TRUE ("Load Test")) -> ()
    }
  }
  n64 = disable-structure shown="Disabled" {
    frame Disabled {
      w69 = T5 {"Row"=0, "Column"=0} ("Selection Start")
      w68 = string[][] [] ("LoTable_1")
      n65 = property on="LoTable_1" class="Tbl (strict)"("Value"=w68, "Selection Start"=w69, "Selection Size"=w69) -> ()  [unwired: 2 in, 2 out]
      n66 = property on="UpTable_1" class="Tbl (strict)"("Value"=w68, "Selection Start"=w69, "Selection Size"=w69) -> ()  [unwired: 2 in, 2 out]
      n67 = property on="LoTable_2" class="Tbl (strict)"("Value"=w68, "Selection Start"=w69, "Selection Size"=w69) -> ()  [unwired: 2 in, 2 out]
      n68 = property on="UpTable_2" class="Tbl (strict)"("Value"=w68, "Selection Start"=w69, "Selection Size"=w69) -> ()  [unwired: 2 in, 2 out]
    }
    frame Enabled {
    }
  }
  n69 = while {
    tunnel: w3 -> [_]
    tunnel: ["stop"] -> w2
    tunnel: w1 -> [w73]
    stop <- w79 stop-if-true
    # "5"
    n70 = event shown="[14] \"Data Name\": Value Change" {
      selector: _ -> [_ _ _ _ _ _ _ _ _ _ _ _ _ _ _ _ _ _ _ _ _ _ _ _ _ _ _ _ _ _ _ _ _ _ _ _ _ _ _ _ _ _ _ _ _ _ _ _ _ _ _ _ _ _ _]
      dyn-events: _ -> [_ _ _ _ _ _ _ _ _ _ _ _ _ _ _ _ _ _ _ _ _ _ _ _ _ _ _ _ _ _ _ _ _ _ _ _ _ _ _ _ _ _ _ _ _ _ _ _ _ _ _ _ _ _ _]
      timeout: 10 -> [_ _ _ _ _ _ _ _ _ _ _ _ _ _ _ _ _ _ _ _ _ _ _ _ _ _ _ _ _ _ _ _ _ _ _ _ _ _ _ _ _ _ _ _ _ _ _ _ _ _ _ _ _ _ _]
      tunnel: w73 -> [_ _ _ _ _ _ _ _ _ _ _ _ _ w730 w816 _ _ w1291 w1337 _ _ w1804 w1850 _ _ _ _ _ _ _ _ _ _ _ _ _ _ _ _ _ _ _ _ _ _ _ _ _ _ _ _ _ _ _ _]
      event Timeout {
        n71 = event-data() -> ()  [unwired: 3 out]
      }
      event Pane Size {
        n72 = event-data() -> ()  [unwired: 7 out]
        n73 = control-ref of="Board Tab"() -> (w88:refnum<vi>)
        n74 = control-ref of="This VI"() -> (w86:refnum<vi>)
        n75 = call "CRYAlign Steps VI Center.vi"("Tab2"=w88, "Input/Output"=TRUE ("Preview"), "VIRef"=w86) -> ()  [unwired: 1 in, 8 out]
      }
      event "Load...": Value Change {
        n76 = event-data() -> ("CtlRef"=w89:refnum<vi>)  [unwired: 6 out]
        n77 = local read "Load Test"() -> (w91:bool)
        n78 = property class="Bool (strict)"(reference=w89, "Value"=FALSE) -> ()  [unwired: 1 in, 2 out]
        n79 = case shown="False" w91 {
          frame False {
            n80 = global read "CRYMainGlobal.vi" "Steps path"() -> (w98:path)
            n81 = local read "Proper VI No"() -> (w92:i32)
            n82 = Build Path(base path=w98, name or relative path="CRYLimits") -> (appended path=w99:path)
            n83 = call "CRYStep Read.vi"("Category Name"="Limits", "Proper VI No"=w92, "Step File Path"=w99) -> ("status"=w95:bool, "selected path"=w93:path, "Flatten Step"=w94:string)  [unwired: 1 in, 3 out]
            n84 = case shown="True" w95 {
              tunnel: w94 -> [_ w100]
              tunnel: w93 -> [_ w102]
              tunnel: w92 -> [_ w101]
              frame False {
              }
              frame True {
                n85 = call "CRYUnflatten Limits.vi"("Unflatten Limits"=w100) -> ("Error?"=w104:bool, "Limits"=w103:T1)  [unwired: 1 in, 8 out]
                n86 = case shown="False" w104 {
                  tunnel: w103 -> [w108 _]
                  tunnel: w102 -> [w107 _]
                  tunnel: w101 -> [w106 _]
                  tunnel: w100 -> [w105 _]
                  frame False {
                    n87 = flat-sequence {
                      tunnel: w108 -> [w120]
                      tunnel: w107 -> [w117]
                      tunnel: w106 -> [w116]
                      tunnel: w105 -> [w115]
                      frame #0 {
                        n88 = Strip Path(path=w117) -> (name=w110:string)  [unwired: 1 out]
                        n89 = local write "Limit Cluster"(w120) -> ()
                        n90 = Reverse String(1:w110) -> (0:w112:string)
                        n91 = Match Pattern(string=w112, regular expression="[.]") -> (after substring=w113:string)  [unwired: 4 out]
                        n92 = Reverse String(1:w113) -> (0:w109:string)
                        n93 = call "CRYPreUpdate Sequence.vi"("EventName"="Load", "StepName Arg3"=w109, "Proper VI No"=w116, "Project View Step Name Identifier Arg1"="", "Step flattened Arg2"=w115, "AllChangeFlg"=TRUE ("Name/Identifier")) -> ()  [unwired: 10 in]
                      }
                      frame #1 {
                        n94 = local write "Load Test"(TRUE ("Load Test")) -> ()
                      }
                    }
                  }
                  frame True {
                  }
                }
              }
            }
          }
          frame True {
          }
        }
      }
      event "Revert": Value Change {
        n95 = event-data() -> ("CtlRef"=w123:refnum<vi>)  [unwired: 6 out]
        n96 = property class="Bool (strict)"(reference=w123, "Value"=FALSE) -> ()  [unwired: 1 in, 2 out]
        n97 = flat-sequence {
          frame #0 {
            n98 = local read "Limit Cluster Bk"() -> (w124:T1)
            n99 = local write "Limit Cluster"(w124) -> ()
          }
          frame #1 {
            n100 = local write "Load Test"(TRUE ("Load Test")) -> ()
          }
        }
      }
      event "Save As...": Value Change {
        w131 = enum32{"Single Values", "Curves", "Waveforms"}."Waveforms" ("y")
        n101 = event-data() -> ("CtlRef"=w126:refnum<vi>)  [unwired: 6 out]
        n102 = local read "Lo_type"() -> (w132:enum32{"Single Values", "Curves", "Waveforms"})
        n103 = local read "Up_type"() -> (w133:enum32{"Single Values", "Curves", "Waveforms"})
        n104 = property class="Bool (strict)"(reference=w126, "Value"=FALSE) -> ()  [unwired: 1 in, 2 out]
        n105 = Not Equal?(x=w133, y=w131) -> (x != y?=w129:bool)
        n106 = Not Equal?(x=w131, y=w132) -> (x != y?=w128:bool)
        n107 = And(x=w129, y=w128) -> (x .and. y?=w130:bool)
        n108 = case shown="True" w130 {
          tunnel: [TRUE ("Do save") w146] -> w134
          frame False {
          }
          frame True {
            n109 = local read "Type"() -> (w141:u16)
            n110 = local read "UpSource"() -> (w137:u16)
            n111 = local read "LoSource"() -> (w136:u16)
            n112 = Not Equal To 0?(x=w141) -> (x != 0?=w142:bool)
            n113 = case shown="False" w142 {
              tunnel: [w151 w163] -> w140
              tunnel: [w149 w160] -> w139
              tunnel: w137 -> [w148 w167]
              tunnel: w136 -> [w147 w166]
              frame False {
                w153 = 0.0 ("UpSingleVal")
                n114 = case shown="0, Default" w148 {
                  tunnel: [w158 w159] -> w155
                  frame 0, Default {
                    n115 = local read "Up Limit Val"() -> (w158:dbl)
                  }
                  frame 1 {
                    n116 = local read "UpSingleVal"() -> (w159:dbl)
                  }
                }
                n117 = case shown="0, Default" w147 {
                  tunnel: [w156 w157] -> w154
                  frame 0, Default {
                    n118 = local read "Lo Limit Val"() -> (w156:dbl)
                  }
                  frame 1 {
                    n119 = local read "LoSingleVal"() -> (w157:dbl)
                  }
                }
                n120 = Bundle("UpSingleVal"=w153, "UpSingleVal"=w155) -> (w152:cluster{"UpSingleVal":dbl, "UpSingleVal":dbl})  [unwired: 1 out]
                n121 = Bundle("UpSingleVal"=w153, "LoSingleVal"=w154) -> (w150:cluster{"UpSingleVal":dbl, "LoSingleVal":dbl})  [unwired: 1 out]
                n122 = Build Array(w152) -> (w151:cluster{"UpSingleVal":dbl, "UpSingleVal":dbl}[])
                n123 = Build Array(w150) -> (w149:cluster{"UpSingleVal":dbl, "LoSingleVal":dbl}[])
              }
              frame True {
                n124 = case shown="0, Default" w167 {
                  tunnel: [w170 w171] -> w165
                  frame 0, Default {
                    n125 = local read "UpTable_1"() -> (w170:string[][])
                  }
                  frame 1 {
                    n126 = local read "UpTable_2"() -> (w171:string[][])
                  }
                }
                n127 = case shown="0, Default" w166 {
                  tunnel: [w168 w169] -> w161
                  frame 0, Default {
                    n128 = local read "LoTable_1"() -> (w168:string[][])
                  }
                  frame 1 {
                    n129 = local read "LoTable_2"() -> (w169:string[][])
                  }
                }
                n130 = call "CRYTable Empty Ignore.vi"("Table In"=w161) -> ("Table Out"=w162:string[][])  [unwired: 10 in]
                n131 = call "CRYTable Empty Ignore.vi"("Table In"=w165) -> ("Table Out"=w164:string[][])  [unwired: 10 in]
                n132 = call "CRYTable to Curve.vi"("Table In"=w164) -> ("Limit curve"=w163:cluster{"Numeric":dbl, "Numeric 2":dbl}[])  [unwired: 10 in]
                n133 = call "CRYTable to Curve.vi"("Table In"=w162) -> ("Limit curve"=w160:cluster{"Numeric":dbl, "Numeric 2":dbl}[])  [unwired: 10 in]
              }
            }
            n134 = local read "Limits_Ring"() -> (w138:u16)
            n135 = local read "up_unit"() -> (w144:string)
            n136 = local read "low_unit"() -> (w143:string)
            n137 = local read "data unit"() -> (w145:string)
            n138 = call "CRYSUpper_Lowerness Check.vi"("Limits"=w138, "Lo unit"=w143, "Data unit"=w145, "Up unit"=w144, "Type"=w141, "Lo source"=w136, "Up source"=w137, "Lower limit"=w139, "Upper limit"=w140) -> ("Do save"=w146:bool)  [unwired: 2 out]
          }
        }
        n139 = case shown="True" w134 {
          frame False {
          }
          frame True {
            w175 = "Limits" ("Step File Name")
            n140 = local read "Limit Cluster"() -> (w173:T1)
            n141 = global read "CRYMainGlobal.vi" "Steps path"() -> (w179:path)
            n142 = local read "Proper VI No"() -> (w176:i32)
            n143 = Build Path(base path=w179, name or relative path="CRYLimits") -> (appended path=w177:path)
            n144 = call "CRYFlatten Limits.vi"("Limits"=w173) -> ("Flatten Limits String"=w172:string)  [unwired: 10 out]
            n145 = call "CRYStep Write.vi"("StepIdentifier"="", "Default"=FALSE, "Proper VI No"=w176, "Category Name"=w175, "Step File Path"=w177, "Step flattened"=w172, "Step File Name"=w175) -> ()  [unwired: 1 in, 4 out]
          }
        }
      }
      event Panel Close {
        n146 = event-data() -> ()  [unwired: 5 out]
        n147 = control-ref of="This VI"() -> (w182:refnum<vi>)
        n148 = local write "Cancel"(TRUE ("Cancel")) -> ()
        n149 = call "CRYWork Before Step Close.vi"("StepVI Ref"=w182) -> ()  [unwired: 11 in]
      }
      event "CurLibChange": Value Change {
        n150 = event-data() -> ()  [unwired: 7 out]
        n151 = flat-sequence {
          frame #0 {
            n152 = property on="Type" class="Slide (strict)"() -> ("Value"=w183:u16)  [unwired: 2 in, 2 out]
            n153 = property on="Up_type" class="RadioBtnsControl (strict)"() -> ("Value"=w184:enum32{"Single Values", "Curves", "Waveforms"})  [unwired: 2 in, 2 out]
            n154 = property on="Lo_type" class="RadioBtnsControl (strict)"() -> ("Value"=w185:enum32{"Single Values", "Curves", "Waveforms"})  [unwired: 2 in, 2 out]
            n155 = property on="Lo_type" class="RadioBtnsControl (strict)"("Val(Sgnl)"=w185) -> ()  [unwired: 2 in, 2 out]
            n156 = property on="Up_type" class="RadioBtnsControl (strict)"("Val(Sgnl)"=w184) -> ()  [unwired: 2 in, 2 out]
            n157 = property on="Type" class="Slide (strict)"("Val(Sgnl)"=w183) -> ()  [unwired: 2 in, 2 out]
          }
          frame #1 {
            w186 = FALSE ("Visible")
            n158 = property on="Verdict" class="Bool (strict)"("Visible"=w186) -> ()  [unwired: 2 in, 2 out]
            n159 = property on="Margin" class="DigNum (strict)"("Visible"=w186) -> ()  [unwired: 2 in, 2 out]
            n160 = property on="tolerance" class="Str"("Visible"=w186) -> ()  [unwired: 2 in, 2 out]
          }
        }
      }
      event "Main Tab": Value Change {
        n161 = event-data() -> ("NewVal"=w188:enum32{"Data", "Parameters", "Help"})  [unwired: 6 out]
        n162 = local read "Type"() -> (w187:u16)
        n163 = local read "Limit Cluster"() -> (w190:T1)
        n164 = Bundle By Name(cluster=w190, "Tab Value"=w188) -> (w189:T1)
        n165 = local write "Limit Cluster"(w189) -> ()
        n166 = case shown="\"Parameters\"" w188 {
          tunnel: w187 -> [_ w192]
          frame "Data", Default {
          }
          frame "Parameters" {
            n167 = case shown="3" w192 {
              tunnel: [w195 w207 "s" ("size_unit") w223] -> w191
              frame 0 {
                w200 = u16 1 items=["Individual Points", "Absolute Limits", "Floating Limits", "Floating Data", "Aligned Limits", "Aligned Data"] ("Alignment")
                w194 = u8 2 ("Disabled")
                # "single value"
                n168 = property on="Alignment" class="Ring (strict)"("Disabled"=w194) -> ()  [unwired: 2 in, 2 out]
                n169 = property on="X Resolution" class="DigNum (strict)"("Disabled"=w194) -> ()  [unwired: 2 in, 2 out]
                n170 = property on="Step Size" class="DigNum (strict)"("Disabled"=w194) -> ()  [unwired: 2 in, 2 out]
                n171 = property on="Minimum" class="DigNum (strict)"("Disabled"=w194) -> ()  [unwired: 2 in, 2 out]
                n172 = property on="Limits_Ring" class="Ring (strict)"("Disabled"=u8 0) -> ()  [unwired: 2 in, 2 out]
                n173 = property on="Y AlignRef" class="DigNum (strict)"("Disabled"=w194) -> ()  [unwired: 2 in, 2 out]
                n174 = property on="Mapping" class="Slide (strict)"("Disabled"=w194) -> ()  [unwired: 2 in, 2 out]
                n175 = property on="size_unit" class="Str"("Disabled"=w194) -> ()  [unwired: 2 in, 2 out]
                n176 = property on="Maximum" class="DigNum (strict)"("Disabled"=w194) -> ()  [unwired: 2 in, 2 out]
                n177 = property on="X AlignRef" class="DigNum (strict)"("Disabled"=w194) -> ()  [unwired: 2 in, 2 out]
                n178 = property on="x float" class="Bool (strict)"("Disabled"=w194) -> ()  [unwired: 2 in, 2 out]
                n179 = local write "x float"(FALSE ("x float")) -> ()
                n180 = local read "Mapping"() -> (w199:u16)
                n181 = local write "Alignment"(w200) -> ()
                n182 = Equal To 0?(x=w199) -> (x = 0?=w198:bool)
                n183 = Select(t="Hz" ("size_unit"), s=w198, f="%" ("size_unit")) -> (s? t:f=w195:string)
              }
              frame 1, Default {
                w204 = u8 0 ("Disabled")
                w205 = u8 2 ("Disabled")
                # "curve"
                n184 = property on="Step Size" class="DigNum (strict)"("Disabled"=w205) -> ()  [unwired: 2 in, 2 out]
                n185 = property on="Minimum" class="DigNum (strict)"("Disabled"=w205) -> ()  [unwired: 2 in, 2 out]
                n186 = property on="Y AlignRef" class="DigNum (strict)"("Disabled"=w205) -> ()  [unwired: 2 in, 2 out]
                n187 = property on="X Resolution" class="DigNum (strict)"("Disabled"=w204) -> ()  [unwired: 2 in, 2 out]
                n188 = property on="Alignment" class="Ring (strict)"("Disabled"=w204) -> ()  [unwired: 2 in, 2 out]
                n189 = property on="Limits_Ring" class="Ring (strict)"("Disabled"=u8 0) -> ()  [unwired: 2 in, 2 out]
                n190 = property on="X AlignRef" class="DigNum (strict)"("Disabled"=w205) -> ()  [unwired: 2 in, 2 out]
                n191 = property on="size_unit" class="Str"("Disabled"=w205) -> ()  [unwired: 2 in, 2 out]
                n192 = property on="Maximum" class="DigNum (strict)"("Disabled"=w205) -> ()  [unwired: 2 in, 2 out]
                n193 = property on="Mapping" class="Slide (strict)"("Disabled"=w204) -> ()  [unwired: 2 in, 2 out]
                n194 = property on="x float" class="Bool (strict)"("Disabled"=w204) -> ()  [unwired: 2 in, 2 out]
                n195 = local read "Mapping"() -> (w211:u16)
                n196 = local read "Alignment"() -> (w206:u16)
                n197 = Equal To 0?(x=w211) -> (x = 0?=w210:bool)
                n198 = local read "x float"() -> (w202:bool)
                n199 = property on="Alignment" class="Ring (strict)"("Val(Sgnl)"=w206) -> ()  [unwired: 2 in, 2 out]
                n200 = Select(t="Hz" ("size_unit"), s=w210, f="%" ("size_unit")) -> (s? t:f=w207:string)
                n201 = property on="x float" class="Bool (strict)"("Val(Sgnl)"=w202) -> ()  [unwired: 2 in, 2 out]
              }
              frame 2 {
                w214 = u8 0 ("Disabled")
                w215 = u8 2 ("Disabled")
                w218 = u16 0 items=["Linear", "Log"] ("Mapping")
                # "waveform"
                n202 = property on="Y AlignRef" class="DigNum (strict)"("Disabled"=w215) -> ()  [unwired: 2 in, 2 out]
                n203 = property on="Step Size" class="DigNum (strict)"("Disabled"=w215) -> ()  [unwired: 2 in, 2 out]
                n204 = property on="Minimum" class="DigNum (strict)"("Disabled"=w215) -> ()  [unwired: 2 in, 2 out]
                n205 = property on="X Resolution" class="DigNum (strict)"("Disabled"=w214) -> ()  [unwired: 2 in, 2 out]
                n206 = property on="Alignment" class="Ring (strict)"("Disabled"=w214) -> ()  [unwired: 2 in, 2 out]
                n207 = property on="Limits_Ring" class="Ring (strict)"("Disabled"=u8 0) -> ()  [unwired: 2 in, 2 out]
                n208 = property on="X AlignRef" class="DigNum (strict)"("Disabled"=w215) -> ()  [unwired: 2 in, 2 out]
                n209 = property on="size_unit" class="Str"("Disabled"=w215) -> ()  [unwired: 2 in, 2 out]
                n210 = property on="Maximum" class="DigNum (strict)"("Disabled"=w215) -> ()  [unwired: 2 in, 2 out]
                n211 = property on="Mapping" class="Slide (strict)"("Disabled"=w214) -> ()  [unwired: 2 in, 2 out]
                n212 = property on="x float" class="Bool (strict)"("Disabled"=w214) -> ()  [unwired: 2 in, 2 out]
                n213 = local read "Alignment"() -> (w216:u16)
                n214 = local read "x float"() -> (w212:bool)
                n215 = property on="Alignment" class="Ring (strict)"("Val(Sgnl)"=w216) -> ()  [unwired: 2 in, 2 out]
                n216 = property on="x float" class="Bool (strict)"("Val(Sgnl)"=w212) -> ()  [unwired: 2 in, 2 out]
                n217 = local write "Mapping"(w218) -> ()
              }
              frame 3 {
                w221 = u8 2 ("Disabled")
                w222 = u16 1 items=["Individual Points", "Absolute Limits", "Floating Limits", "Floating Data", "Aligned Limits", "Aligned Data"] ("Alignment")
                # "multimeter"
                n218 = property on="Alignment" class="Ring (strict)"("Disabled"=w221) -> ()  [unwired: 2 in, 2 out]
                n219 = property on="X Resolution" class="DigNum (strict)"("Disabled"=w221) -> ()  [unwired: 2 in, 2 out]
                n220 = property on="Step Size" class="DigNum (strict)"("Disabled"=w221) -> ()  [unwired: 2 in, 2 out]
                n221 = property on="Minimum" class="DigNum (strict)"("Disabled"=w221) -> ()  [unwired: 2 in, 2 out]
                n222 = local write "x float"(FALSE ("x float")) -> ()
                n223 = property on="Limits_Ring" class="Ring (strict)"("Disabled"=u8 0) -> ()  [unwired: 2 in, 2 out]
                n224 = property on="Y AlignRef" class="DigNum (strict)"("Disabled"=w221) -> ()  [unwired: 2 in, 2 out]
                n225 = property on="Mapping" class="Slide (strict)"("Disabled"=w221) -> ()  [unwired: 2 in, 2 out]
                n226 = property on="size_unit" class="Str"("Disabled"=w221) -> ()  [unwired: 2 in, 2 out]
                n227 = property on="Maximum" class="DigNum (strict)"("Disabled"=w221) -> ()  [unwired: 2 in, 2 out]
                n228 = property on="X AlignRef" class="DigNum (strict)"("Disabled"=w221) -> ()  [unwired: 2 in, 2 out]
                n229 = property on="x float" class="Bool (strict)"("Disabled"=w221) -> ()  [unwired: 2 in, 2 out]
                n230 = local read "Mapping"() -> (w227:u16)
                n231 = disable-structure shown="Disabled" {
                  frame Disabled {
                    w229 = u16 1 items=["Individual Points", "Absolute Limits", "Floating Limits", "Floating Data", "Aligned Limits", "Aligned Data"] ("Alignment")
                    n232 = property on="x float" class="Bool (strict)"("Val(Sgnl)"=FALSE ("Value (Signaling)")) -> ()  [unwired: 2 in, 2 out]
                    n233 = property on="Alignment" class="Ring (strict)"("Val(Sgnl)"=w229) -> ()  [unwired: 2 in, 2 out]
                  }
                  frame Enabled {
                  }
                }
                n234 = Equal To 0?(x=w227) -> (x = 0?=w226:bool)
                n235 = local write "Alignment"(w222) -> ()
                n236 = Select(t="Hz" ("size_unit"), s=w226, f="%" ("size_unit")) -> (s? t:f=w223:string)
              }
            }
            n237 = local write "size_unit"(w191) -> ()
          }
        }
      }
      event "Limits Graph": Cursor Move {
        n238 = event-data() -> ("CursLoc"=w230:cluster{"X":dbl, "Y":dbl})  [unwired: 9 out]
        n239 = disable-structure shown="Disabled" {
          disable-tunnel: w230 -> [w231 _]
          frame Disabled {
            n240 = local read "Limit Cluster"() -> (w237:T1)
            n241 = local read "Plot index"() -> (w238:i32)
            n242 = local read "X Resolution"() -> (w233:u8)
            n243 = local read "Y Resolution"() -> (w232:u8)
            n244 = local read "Point index"() -> (w234:i32)
            n245 = Unbundle By Name(w237) -> ("Upper Limit"=w236:cluster{dbl, dbl}[], "Lower Limit"=w235:cluster{dbl, dbl}[])
            n246 = flat-sequence {
              tunnel: w231 -> [w246]
              tunnel: w238 -> [w245]
              tunnel: w237 -> [w244]
              tunnel: w236 -> [w243]
              tunnel: w235 -> [w242]
              tunnel: w234 -> [w241]
              tunnel: w233 -> [w240]
              tunnel: w232 -> [w239]
              frame #0 {
                n247 = case shown="1, Default" w245 {
                  tunnel: w244 -> [w254 w271]
                  tunnel: w243 -> [w251 _]
                  tunnel: w242 -> [_ w270]
                  tunnel: w241 -> [w253 w268]
                  tunnel: w246 -> [w252 w269]
                  tunnel: w240 -> [w250 w267]
                  tunnel: w239 -> [w249 w266]
                  frame 1, Default {
                    n248 = local read "UpSource"() -> (w248:u16)
                    n249 = Equal To 0?(x=w248) -> (x = 0?=w247:bool)
                    n250 = case shown="True" w247 {
                      tunnel: w254 -> [_ w263]
                      tunnel: w253 -> [_ w262]
                      tunnel: w252 -> [_ w261]
                      tunnel: w251 -> [_ w260]
                      tunnel: w250 -> [_ w257]
                      tunnel: w249 -> [_ w256]
                      frame False {
                      }
                      frame True {
                        n251 = Replace Array Subset(array=w260, new element=w261, index=w262) -> (w258:cluster{dbl, dbl}[])
                        n252 = call "CRYCurve to Table.vi"("y precision"=w256, "x precision"=w257, "Limit curve In"=w258) -> ("Limit Table"=w259:string[][])  [unwired: 7 in, 1 out]
                        n253 = local write "UpTable_1"(w259) -> ()
                        n254 = Bundle By Name(cluster=w263, "Upper Limit"=w258) -> (w255:T1)
                        n255 = local write "Limit Cluster"(w255) -> ()
                      }
                    }
                  }
                  frame 2 {
                    n256 = local read "LoSource"() -> (w265:u16)
                    n257 = Equal To 0?(x=w265) -> (x = 0?=w264:bool)
                    n258 = case shown="True" w264 {
                      tunnel: w271 -> [_ w280]
                      tunnel: w270 -> [_ w279]
                      tunnel: w269 -> [_ w278]
                      tunnel: w268 -> [_ w277]
                      tunnel: w267 -> [_ w274]
                      tunnel: w266 -> [_ w273]
                      frame False {
                      }
                      frame True {
                        n259 = Replace Array Subset(array=w279, new element=w278, index=w277) -> (w276:cluster{dbl, dbl}[])
                        n260 = call "CRYCurve to Table.vi"("y precision"=w273, "x precision"=w274, "Limit curve In"=w276) -> ("Limit Table"=w275:string[][])  [unwired: 7 in, 1 out]
                        n261 = Bundle By Name(cluster=w280, "Lower Limit"=w276) -> (w272:T1)
                        n262 = local write "LoTable_1"(w275) -> ()
                        n263 = local write "Limit Cluster"(w272) -> ()
                      }
                    }
                  }
                }
              }
              frame #1 {
                n264 = local write "Plot graphs"(TRUE ("Plot graphs")) -> ()
              }
            }
          }
          frame Enabled {
          }
        }
      }
      event "Limits Graph": Mouse Down {
        n265 = event-data() -> ("Coords"=w293:T10)  [unwired: 8 out]
        n266 = property on="Limits Graph" class="XYGraph (strict)"() -> ("XScale.Mapping Mode"=w284:u8)  [unwired: 2 in, 2 out]
        n267 = property on="Limits Graph" class="XYGraph (strict)"() -> ("Plot Bounds"=w292:T11, "Plot Area Size"=w291:T4, "XScale.Range"=w290:T12, "YScale.Range"=w289:T12, "Value"=w287:cluster{"element":cluster{"x":dbl, "y":dbl}[]}[])  [unwired: 2 in, 2 out]
        n268 = call "CRYPixel to x-y.vi"("Y Scale.Range"=w289, "MapMode"=w284, "X Scale.Range"=w290, "Plot Area:Size"=w291, "Plot Area Bounds"=w292, "Graph Cordinate"=w293) -> ("x-y cordinate"=w286:cluster{dbl, dbl}, "abs(x)"=w294:cluster{dbl, dbl})  [unwired: 4 out]
        n269 = call "CRYPoint Clicked Check.vi"("MapMode"=w284, "X-Y position of mouse"=w286, "Units per pixel"=w294, "Limits graph"=w287) -> ("Pointer Clicked"=w288:bool, "Point index"=w283:i32, "Plot index"=w282:i32)  [unwired: 5 out]
        n270 = Unbundle(w286) -> (w285:dbl)  [unwired: 1 out]
        n271 = case shown="True" w288 {
          tunnel: w282 -> [_ w296]
          tunnel: w283 -> [_ w297]
          tunnel: w287 -> [_ w301]
          tunnel: w285 -> [_ w300]
          frame False {
            n272 = local write "cursor move"(FALSE ("cursor move")) -> ()
          }
          frame True {
            n273 = case shown="1" w296 {
              tunnel: w301 -> [_ w308 w323]
              tunnel: w296 -> [_ w307 w322]
              tunnel: w297 -> [_ w306 w321]
              tunnel: w300 -> [_ w305 w320]
              frame Default {
                n274 = local write "cursor move"(FALSE ("cursor move")) -> ()
              }
              frame 1 {
                n275 = local read "UpSource"() -> (w310:u16)
                n276 = Equal To 0?(x=w310) -> (x = 0?=w309:bool)
                n277 = case shown="True" w309 {
                  tunnel: w308 -> [_ w316]
                  tunnel: w307 -> [_ w315]
                  tunnel: w306 -> [_ w314]
                  tunnel: w305 -> [_ w313]
                  frame False {
                    n278 = local write "cursor move"(FALSE ("cursor move")) -> ()
                  }
                  frame True {
                    n279 = Index Array(array=w316, index=w315) -> (element=w318:cluster{"element":cluster{"x":dbl, "y":dbl}[]})
                    n280 = Unbundle(w318) -> ("element"=w319:cluster{"x":dbl, "y":dbl}[])
                    n281 = Index Array(array=w319, index=w314) -> (element=w317:cluster{"x":dbl, "y":dbl})
                    n282 = property on="Limits Graph" class="XYGraph (strict)"("Cursor.Cursor Position"=w317) -> ()  [unwired: 2 in, 2 out]
                    n283 = local write "cursor move"(TRUE ("cursor move")) -> ()
                    n284 = local write "Up_oldx"(w313) -> ()
                  }
                }
              }
              frame 2 {
                n285 = local read "LoSource"() -> (w325:u16)
                n286 = Equal To 0?(x=w325) -> (x = 0?=w324:bool)
                n287 = case shown="True" w324 {
                  tunnel: w323 -> [_ w331]
                  tunnel: w322 -> [_ w330]
                  tunnel: w321 -> [_ w329]
                  tunnel: w320 -> [_ w328]
                  frame False {
                    n288 = local write "cursor move"(FALSE ("cursor move")) -> ()
                  }
                  frame True {
                    n289 = Index Array(array=w331, index=w330) -> (element=w333:cluster{"element":cluster{"x":dbl, "y":dbl}[]})
                    n290 = Unbundle(w333) -> ("element"=w334:cluster{"x":dbl, "y":dbl}[])
                    n291 = Index Array(array=w334, index=w329) -> (element=w332:cluster{"x":dbl, "y":dbl})
                    n292 = property on="Limits Graph" class="XYGraph (strict)"("Cursor.Cursor Position"=w332) -> ()  [unwired: 2 in, 2 out]
                    n293 = local write "cursor move"(TRUE ("cursor move")) -> ()
                    n294 = local write "Lo_oldx"(w328) -> ()
                  }
                }
              }
            }
            n295 = property on="Limits Graph" class="XYGraph (strict)"("Cursor.Cursor Plot"=w296, "Cursor.Cursor Index"=w297) -> ()  [unwired: 2 in, 2 out]
            n296 = Not Equal?(x=-1, y=w297) -> (x != y?=w298:bool)
            n297 = case shown="True" w298 {
              tunnel: w297 -> [_ w302]
              tunnel: w296 -> [_ w303]
              frame False {
              }
              frame True {
                "Plot index" <- w303
                "Point index" <- w302
              }
            }
          }
        }
      }
      event "Limits Graph": Mouse Up {
        n298 = event-data() -> ()  [unwired: 9 out]
        n299 = local write "cursor move"(FALSE ("cursor move")) -> ()
      }
      event "Limits Graph": Mouse Move {
        n300 = event-data() -> ("Coords"=w341:T10)  [unwired: 5 out]
        n301 = local read "cursor move"() -> (w338:bool)
        n302 = call "CRYMouse.vi"() -> ("Current Button State"=w339:bool[])  [unwired: 8 out]
        n303 = Index Array(array=w339, index=0 ("Index")) -> (element=w337:bool)
        n304 = And(x=w337, y=w338) -> (x .and. y?=w336:bool)
        n305 = case shown="True" w336 {
          tunnel: w341 -> [_ w362]
          frame False {
          }
          frame True {
            n306 = property on="Limits Graph" class="XYGraph (strict)"("Cursor.Allow Drag"=TRUE) -> ("Plot Bounds"=w361:T11, "Plot Area Size"=w360:T4, "XScale.Range"=w359:T12, "YScale.Range"=w358:T12)  [unwired: 2 in, 2 out]
            n307 = property on="Limits Graph" class="XYGraph (strict)"() -> ("XScale.Mapping Mode"=w342:u8)  [unwired: 2 in, 2 out]
            n308 = local read "X Resolution"() -> (w349:u8)
            n309 = local read "Y Resolution"() -> (w348:u8)
            n310 = property on="Limits Graph" class="XYGraph (strict)"() -> ("Cursor.Cursor Plot"=w357:i32, "Cursor.Cursor Index"=w350:i32)  [unwired: 2 in, 2 out]
            n311 = local read "Limit Cluster"() -> (w347:T1)
            n312 = call "CRYPixel to x-y.vi"("Y Scale.Range"=w358, "MapMode"=w342, "X Scale.Range"=w359, "Plot Area:Size"=w360, "Plot Area Bounds"=w361, "Graph Cordinate"=w362) -> ("x-y cordinate"=w351:cluster{dbl, dbl})  [unwired: 5 out]
            n313 = Unbundle By Name(w347) -> ("Upper Limit"=w356:cluster{dbl, dbl}[], "Lower Limit"=w355:cluster{dbl, dbl}[])
            n314 = Unbundle(w351) -> (w354:dbl, w352:dbl)
            n315 = case shown="1" w342 {
              tunnel: w354 -> [w363 w365]
              tunnel: [w363 w364] -> w353
              frame 0, Default {
              }
              frame 1 {
                n316 = Power Of 10(x=w365) -> (10^x=w364:dbl)
              }
            }
            n317 = Bundle(w353, w352) -> (w346:cluster{dbl, dbl})  [unwired: 1 out]
            n318 = case shown="1, Default" w357 {
              tunnel: w356 -> [w371 _]
              tunnel: w355 -> [_ w548]
              tunnel: w346 -> [w366 w547]
              tunnel: w350 -> [w370 w552]
              tunnel: w349 -> [w369 w551]
              tunnel: w348 -> [w368 w550]
              tunnel: w347 -> [w367 w549]
              frame 1, Default {
                n319 = local read "UpSource"() -> (w373:u16)
                n320 = Equal To 0?(x=w373) -> (x = 0?=w372:bool)
                n321 = case shown="True" w372 {
                  tunnel: w367 -> [w378 _]
                  tunnel: w366 -> [w381 _]
                  tunnel: w371 -> [w382 _]
                  tunnel: w370 -> [w380 _]
                  tunnel: w369 -> [w377 _]
                  tunnel: w368 -> [w376 _]
                  tunnel: w366 -> [w379 _]
                  frame True {
                    n322 = Replace Array Subset(array=w382, new element=w381, index=w380) -> (w375:cluster{dbl, dbl}[])
                    n323 = Array Size(array=w375) -> (size(s)=w374:i32)
                    n324 = case shown="0" w380 {
                      selector: w380 -> [_ w428]
                      tunnel: w375 -> [w391 w434]
                      tunnel: w379 -> [w390 w432]
                      tunnel: w378 -> [w389 w431]
                      tunnel: w377 -> [w388 w429]
                      tunnel: w376 -> [w387 w430]
                      tunnel: w374 -> [w386 w433]
                      frame 0 {
                        n325 = Decrement(x=w386) -> (x-1=w385:i32)
                        n326 = Greater?(x=w385, y=0) -> (0:w383:bool)
                        n327 = case shown="True" w383 {
                          tunnel: w391 -> [w394 w404]
                          tunnel: w390 -> [_ w403]
                          tunnel: w389 -> [w395 w402]
                          tunnel: w388 -> [w393 w401]
                          tunnel: w387 -> [w392 w400]
                          tunnel: w385 -> [_ w399]
                          frame False {
                            n328 = Bundle By Name(cluster=w395, "Upper Limit"=w394) -> (w397:T1)
                            n329 = call "CRYCurve to Table.vi"("y precision"=w392, "x precision"=w393, "Limit curve In"=w394) -> ("Limit Table"=w398:string[][])  [unwired: 7 in, 1 out]
                            n330 = local write "Limit Cluster"(w397) -> ()
                            n331 = local write "UpTable_1"(w398) -> ()
                            n332 = local write "Plot graphs"(TRUE ("Plot graphs")) -> ()
                          }
                          frame True {
                            n333 = for {
                              N: w399 -> [_]
                              tunnel: w403 -> [w414]
                              tunnel: w402 -> [w411]
                              tunnel: w401 -> [w410]
                              tunnel: w400 -> [w409]
                              shift-right: [w405] -> _
                              shift-left: w404 -> [w415]
                              i -> [w420]
                              stop <- w407 stop-if-true
                              n334 = Increment(x=w420) -> (x+1=w406:i32)
                              n335 = Index Array(array=w415, index=w406) -> (element=w419:cluster{dbl, dbl})
                              n336 = Unbundle(w419) -> (w418:dbl)  [unwired: 1 out]
                              n337 = Unbundle(w414) -> (w417:dbl)  [unwired: 1 out]
                              n338 = Less?(x=w418, y=w417) -> (x < y?=w416:bool)
                              n339 = case shown="True" w416 {
                                tunnel: w415 -> [w422 w427]
                                tunnel: w406 -> [_ w423]
                                tunnel: w414 -> [_ w426]
                                tunnel: [w422 w425] -> w405
                                tunnel: [TRUE FALSE] -> w407
                                frame False {
                                }
                                frame True {
                                n340 = Replace Array Subset(array=w427, new element=w426, index=w423) -> (w425:cluster{dbl, dbl}[])
                                }
                              }
                              n341 = Bundle By Name(cluster=w411, "Upper Limit"=w405) -> (w412:T1)
                              n342 = call "CRYCurve to Table.vi"("y precision"=w409, "x precision"=w410, "Limit curve In"=w405) -> ("Limit Table"=w413:string[][])  [unwired: 7 in, 1 out]
                              n343 = local write "UpTable_1"(w413) -> ()
                              n344 = local write "Limit Cluster"(w412) -> ()
                              n345 = local write "Plot graphs"(TRUE ("Plot graphs")) -> ()
                            }
                          }
                        }
                      }
                      frame Default {
                        n346 = Decrement(x=w433) -> (x-1=w436:i32)
                        n347 = Less Or Equal?(x=w436, y=w428) -> (x <= y?=w435:bool)
                        n348 = case shown="False" w435 {
                          tunnel: w434 -> [w445 w521]
                          tunnel: w433 -> [w440 w520]
                          tunnel: w432 -> [w444 w519]
                          tunnel: w431 -> [w443 w518]
                          tunnel: w430 -> [w442 w517]
                          tunnel: w429 -> [w441 w516]
                          tunnel: w428 -> [w439 _]
                          frame False {
                            n349 = local read "Up_oldx"() -> (w447:dbl)
                            n350 = Unbundle(w444) -> (w437:dbl)  [unwired: 1 out]
                            n351 = Greater?(x=w447, y=w437) -> (0:w446:bool)
                            n352 = case shown="True" w446 {
                              tunnel: w439 -> [w451 w489]
                              tunnel: w445 -> [w458 w488]
                              tunnel: w444 -> [w457 w487]
                              tunnel: w443 -> [w455 w486]
                              tunnel: w442 -> [w453 w485]
                              tunnel: w441 -> [w454 w484]
                              tunnel: w440 -> [w450 _]
                              tunnel: w439 -> [w456 _]
                              tunnel: [w452 _] -> w438
                              frame False {
                                n353 = Subtract(x=w450, y=w451) -> (x-y=w449:i32)
                                n354 = for {
                                N: w449 -> [_]
                                tunnel: w457 -> [w471]
                                tunnel: w454 -> [w468]
                                tunnel: w453 -> [w467]
                                tunnel: w455 -> [w463]
                                tunnel: w456 -> [w462]
                                tunnel: [w460] -> w452
                                shift-right: [w459] -> _
                                shift-left: w458 -> [w472]
                                i -> [w465]
                                stop <- w460 stop-if-true
                                n355 = Add(x=w462, y=w465) -> (x+y=w461:i32)
                                n356 = Increment(x=w461) -> (x+1=w464:i32)
                                n357 = Index Array(array=w472, index=w464) -> (element=w476:cluster{dbl, dbl})
                                n358 = Unbundle(w476) -> (w475:dbl)  [unwired: 1 out]
                                n359 = Unbundle(w471) -> (w474:dbl)  [unwired: 1 out]
                                n360 = Less Or Equal?(x=w475, y=w474) -> (x <= y?=w473:bool)
                                n361 = case shown="True" w473 {
                                tunnel: w472 -> [w478 w483]
                                tunnel: w464 -> [_ w482]
                                tunnel: w471 -> [_ w481]
                                tunnel: [w478 w480] -> w459
                                tunnel: [TRUE FALSE] -> w460
                                frame False {
                                }
                                frame True {
                                n362 = Replace Array Subset(array=w483, new element=w481, index=w482) -> (w480:cluster{dbl, dbl}[])
                                }
                                }
                                n363 = Bundle By Name(cluster=w463, "Upper Limit"=w459) -> (w469:T1)
                                n364 = call "CRYCurve to Table.vi"("y precision"=w467, "x precision"=w468, "Limit curve In"=w459) -> ("Limit Table"=w470:string[][])  [unwired: 7 in, 1 out]
                                n365 = local write "UpTable_1"(w470) -> ()
                                n366 = local write "Limit Cluster"(w469) -> ()
                                n367 = local write "Plot graphs"(TRUE ("Plot graphs")) -> ()
                                }
                              }
                              frame True {
                                n368 = for {
                                N: w489 -> [w495]
                                tunnel: w487 -> [w502]
                                tunnel: w484 -> [w499]
                                tunnel: w485 -> [w498]
                                tunnel: w486 -> [w491]
                                shift-right: [w490] -> _
                                shift-left: w488 -> [w503]
                                i -> [w494]
                                stop <- w496 stop-if-true
                                n369 = Decrement(x=w495) -> (x-1=w493:i32)
                                n370 = Subtract(x=w493, y=w494) -> (x-y=w492:i32)
                                n371 = Index Array(array=w503, index=w492) -> (element=w507:cluster{dbl, dbl})
                                n372 = Unbundle(w507) -> (w506:dbl)  [unwired: 1 out]
                                n373 = Unbundle(w502) -> (w505:dbl)  [unwired: 1 out]
                                n374 = Greater?(x=w506, y=w505) -> (0:w504:bool)
                                n375 = case shown="True" w504 {
                                tunnel: w503 -> [w509 w514]
                                tunnel: w492 -> [_ w513]
                                tunnel: w502 -> [_ w512]
                                tunnel: [w509 w511] -> w490
                                tunnel: [TRUE FALSE] -> w496
                                frame False {
                                }
                                frame True {
                                n376 = Replace Array Subset(array=w514, new element=w512, index=w513) -> (w511:cluster{dbl, dbl}[])
                                }
                                }
                                n377 = Bundle By Name(cluster=w491, "Upper Limit"=w490) -> (w500:T1)
                                n378 = call "CRYCurve to Table.vi"("y precision"=w498, "x precision"=w499, "Limit curve In"=w490) -> ("Limit Table"=w501:string[][])  [unwired: 7 in, 1 out]
                                n379 = local write "Limit Cluster"(w500) -> ()
                                n380 = local write "UpTable_1"(w501) -> ()
                                n381 = local write "Plot graphs"(TRUE ("Plot graphs")) -> ()
                                }
                              }
                            }
                            n382 = flat-sequence {
                              tunnel: w438 -> [_]
                              tunnel: w437 -> [w448]
                              frame #0 {
                                n383 = local write "Up_oldx"(w448) -> ()
                              }
                            }
                          }
                          frame True {
                            # "end point"
                            n384 = Decrement(x=w520) -> (x-1=w515:i32)
                            n385 = for {
                              N: w515 -> [w526]
                              tunnel: w519 -> [w534]
                              tunnel: w518 -> [w531]
                              tunnel: w516 -> [w530]
                              tunnel: w517 -> [w529]
                              shift-right: [w522] -> _
                              shift-left: w521 -> [w535]
                              i -> [w525]
                              stop <- w527 stop-if-true
                              n386 = Decrement(x=w526) -> (x-1=w524:i32)
                              n387 = Subtract(x=w524, y=w525) -> (x-y=w523:i32)
                              n388 = Index Array(array=w535, index=w523) -> (element=w539:cluster{dbl, dbl})
                              n389 = Unbundle(w539) -> (w538:dbl)  [unwired: 1 out]
                              n390 = Unbundle(w534) -> (w537:dbl)  [unwired: 1 out]
                              n391 = Greater?(x=w538, y=w537) -> (0:w536:bool)
                              n392 = case shown="True" w536 {
                                tunnel: w535 -> [w541 w546]
                                tunnel: w523 -> [_ w545]
                                tunnel: w534 -> [_ w544]
                                tunnel: [w541 w543] -> w522
                                tunnel: [TRUE FALSE] -> w527
                                frame False {
                                }
                                frame True {
                                n393 = Replace Array Subset(array=w546, new element=w544, index=w545) -> (w543:cluster{dbl, dbl}[])
                                }
                              }
                              n394 = Bundle By Name(cluster=w531, "Upper Limit"=w522) -> (w532:T1)
                              n395 = call "CRYCurve to Table.vi"("y precision"=w529, "x precision"=w530, "Limit curve In"=w522) -> ("Limit Table"=w533:string[][])  [unwired: 7 in, 1 out]
                              n396 = local write "UpTable_1"(w533) -> ()
                              n397 = local write "Limit Cluster"(w532) -> ()
                              n398 = local write "Plot graphs"(TRUE ("Plot graphs")) -> ()
                            }
                          }
                        }
                      }
                    }
                  }
                  frame False {
                  }
                }
              }
              frame 2 {
                n399 = local read "LoSource"() -> (w554:u16)
                n400 = Equal To 0?(x=w554) -> (x = 0?=w553:bool)
                n401 = case shown="True" w553 {
                  tunnel: w549 -> [w559 _]
                  tunnel: w547 -> [w562 _]
                  tunnel: w548 -> [w563 _]
                  tunnel: w552 -> [w561 _]
                  tunnel: w551 -> [w558 _]
                  tunnel: w550 -> [w557 _]
                  tunnel: w547 -> [w560 _]
                  frame True {
                    n402 = Replace Array Subset(array=w563, new element=w562, index=w561) -> (w556:cluster{dbl, dbl}[])
                    n403 = Array Size(array=w556) -> (size(s)=w555:i32)
                    n404 = case shown="0" w561 {
                      selector: w561 -> [_ w609]
                      tunnel: w556 -> [w572 w615]
                      tunnel: w560 -> [w571 w613]
                      tunnel: w559 -> [w570 w612]
                      tunnel: w558 -> [w569 w610]
                      tunnel: w557 -> [w568 w611]
                      tunnel: w555 -> [w567 w614]
                      frame 0 {
                        n405 = Decrement(x=w567) -> (x-1=w566:i32)
                        n406 = Greater?(x=w566, y=0) -> (0:w564:bool)
                        n407 = case shown="False" w564 {
                          tunnel: w572 -> [w576 w585]
                          tunnel: w571 -> [_ w584]
                          tunnel: w570 -> [w573 w583]
                          tunnel: w569 -> [w575 w582]
                          tunnel: w568 -> [w574 w581]
                          tunnel: w566 -> [_ w580]
                          frame False {
                            n408 = Bundle By Name(cluster=w573, "Lower Limit"=w576) -> (w578:T1)
                            n409 = call "CRYCurve to Table.vi"("y precision"=w574, "x precision"=w575, "Limit curve In"=w576) -> ("Limit Table"=w579:string[][])  [unwired: 7 in, 1 out]
                            n410 = local write "LoTable_1"(w579) -> ()
                            n411 = local write "Plot graphs"(TRUE ("Plot graphs")) -> ()
                            n412 = local write "Limit Cluster"(w578) -> ()
                          }
                          frame True {
                            n413 = for {
                              N: w580 -> [_]
                              tunnel: w584 -> [w595]
                              tunnel: w583 -> [w592]
                              tunnel: w582 -> [w591]
                              tunnel: w581 -> [w590]
                              shift-right: [w586] -> _
                              shift-left: w585 -> [w596]
                              i -> [w601]
                              stop <- w588 stop-if-true
                              n414 = Increment(x=w601) -> (x+1=w587:i32)
                              n415 = Index Array(array=w596, index=w587) -> (element=w600:cluster{dbl, dbl})
                              n416 = Unbundle(w600) -> (w599:dbl)  [unwired: 1 out]
                              n417 = Unbundle(w595) -> (w598:dbl)  [unwired: 1 out]
                              n418 = Less?(x=w599, y=w598) -> (x < y?=w597:bool)
                              n419 = case shown="False" w597 {
                                tunnel: w596 -> [w603 w608]
                                tunnel: w587 -> [_ w604]
                                tunnel: w595 -> [_ w607]
                                tunnel: [w603 w606] -> w586
                                tunnel: [TRUE FALSE] -> w588
                                frame False {
                                }
                                frame True {
                                n420 = Replace Array Subset(array=w608, new element=w607, index=w604) -> (w606:cluster{dbl, dbl}[])
                                }
                              }
                              n421 = Bundle By Name(cluster=w592, "Lower Limit"=w586) -> (w593:T1)
                              n422 = call "CRYCurve to Table.vi"("y precision"=w590, "x precision"=w591, "Limit curve In"=w586) -> ("Limit Table"=w594:string[][])  [unwired: 7 in, 1 out]
                              n423 = local write "LoTable_1"(w594) -> ()
                              n424 = local write "Limit Cluster"(w593) -> ()
                              n425 = local write "Plot graphs"(TRUE ("Plot graphs")) -> ()
                            }
                          }
                        }
                      }
                      frame Default {
                        n426 = Decrement(x=w614) -> (x-1=w617:i32)
                        n427 = Less Or Equal?(x=w617, y=w609) -> (x <= y?=w616:bool)
                        n428 = case shown="False" w616 {
                          tunnel: w615 -> [w626 w702]
                          tunnel: w614 -> [w621 w701]
                          tunnel: w613 -> [w625 w700]
                          tunnel: w612 -> [w624 w699]
                          tunnel: w611 -> [w623 w698]
                          tunnel: w610 -> [w622 w697]
                          tunnel: w609 -> [w620 _]
                          frame False {
                            n429 = local read "Lo_oldx"() -> (w628:dbl)
                            n430 = Unbundle(w625) -> (w618:dbl)  [unwired: 1 out]
                            n431 = Greater?(x=w628, y=w618) -> (0:w627:bool)
                            n432 = case shown="True" w627 {
                              tunnel: w620 -> [w632 w670]
                              tunnel: w626 -> [w639 w669]
                              tunnel: w625 -> [w638 w668]
                              tunnel: w624 -> [w636 w667]
                              tunnel: w623 -> [w634 w666]
                              tunnel: w622 -> [w635 w665]
                              tunnel: w621 -> [w631 _]
                              tunnel: w620 -> [w637 _]
                              tunnel: [w633 _] -> w619
                              frame False {
                                n433 = Subtract(x=w631, y=w632) -> (x-y=w630:i32)
                                n434 = for {
                                N: w630 -> [_]
                                tunnel: w638 -> [w652]
                                tunnel: w635 -> [w649]
                                tunnel: w634 -> [w648]
                                tunnel: w636 -> [w644]
                                tunnel: w637 -> [w643]
                                tunnel: [w641] -> w633
                                shift-right: [w640] -> _
                                shift-left: w639 -> [w653]
                                i -> [w646]
                                stop <- w641 stop-if-true
                                n435 = Add(x=w643, y=w646) -> (x+y=w642:i32)
                                n436 = Increment(x=w642) -> (x+1=w645:i32)
                                n437 = Index Array(array=w653, index=w645) -> (element=w657:cluster{dbl, dbl})
                                n438 = Unbundle(w657) -> (w656:dbl)  [unwired: 1 out]
                                n439 = Unbundle(w652) -> (w655:dbl)  [unwired: 1 out]
                                n440 = Less Or Equal?(x=w656, y=w655) -> (x <= y?=w654:bool)
                                n441 = case shown="True" w654 {
                                tunnel: w653 -> [w659 w664]
                                tunnel: w645 -> [_ w663]
                                tunnel: w652 -> [_ w662]
                                tunnel: [w659 w661] -> w640
                                tunnel: [TRUE FALSE] -> w641
                                frame False {
                                }
                                frame True {
                                n442 = Replace Array Subset(array=w664, new element=w662, index=w663) -> (w661:cluster{dbl, dbl}[])
                                }
                                }
                                n443 = Bundle By Name(cluster=w644, "Lower Limit"=w640) -> (w650:T1)
                                n444 = call "CRYCurve to Table.vi"("y precision"=w648, "x precision"=w649, "Limit curve In"=w640) -> ("Limit Table"=w651:string[][])  [unwired: 7 in, 1 out]
                                n445 = local write "LoTable_1"(w651) -> ()
                                n446 = local write "Limit Cluster"(w650) -> ()
                                n447 = local write "Plot graphs"(TRUE ("Plot graphs")) -> ()
                                }
                              }
                              frame True {
                                n448 = for {
                                N: w670 -> [w676]
                                tunnel: w668 -> [w683]
                                tunnel: w665 -> [w680]
                                tunnel: w666 -> [w679]
                                tunnel: w667 -> [w672]
                                shift-right: [w671] -> _
                                shift-left: w669 -> [w684]
                                i -> [w675]
                                stop <- w677 stop-if-true
                                n449 = Decrement(x=w676) -> (x-1=w674:i32)
                                n450 = Subtract(x=w674, y=w675) -> (x-y=w673:i32)
                                n451 = Index Array(array=w684, index=w673) -> (element=w688:cluster{dbl, dbl})
                                n452 = Unbundle(w688) -> (w687:dbl)  [unwired: 1 out]
                                n453 = Unbundle(w683) -> (w686:dbl)  [unwired: 1 out]
                                n454 = Greater?(x=w687, y=w686) -> (0:w685:bool)
                                n455 = case shown="False" w685 {
                                tunnel: w684 -> [w690 w695]
                                tunnel: w673 -> [_ w694]
                                tunnel: w683 -> [_ w693]
                                tunnel: [w690 w692] -> w671
                                tunnel: [TRUE FALSE] -> w677
                                frame False {
                                }
                                frame True {
                                n456 = Replace Array Subset(array=w695, new element=w693, index=w694) -> (w692:cluster{dbl, dbl}[])
                                }
                                }
                                n457 = Bundle By Name(cluster=w672, "Lower Limit"=w671) -> (w681:T1)
                                n458 = local write "Limit Cluster"(w681) -> ()
                                n459 = call "CRYCurve to Table.vi"("y precision"=w679, "x precision"=w680, "Limit curve In"=w671) -> ("Limit Table"=w682:string[][])  [unwired: 7 in, 1 out]
                                n460 = local write "LoTable_1"(w682) -> ()
                                n461 = local write "Plot graphs"(TRUE ("Plot graphs")) -> ()
                                }
                              }
                            }
                            n462 = flat-sequence {
                              tunnel: w619 -> [_]
                              tunnel: w618 -> [w629]
                              frame #0 {
                                n463 = local write "Lo_oldx"(w629) -> ()
                              }
                            }
                          }
                          frame True {
                            # "end point"
                            n464 = Decrement(x=w701) -> (x-1=w696:i32)
                            n465 = for {
                              N: w696 -> [w707]
                              tunnel: w700 -> [w715]
                              tunnel: w699 -> [w712]
                              tunnel: w697 -> [w711]
                              tunnel: w698 -> [w710]
                              shift-right: [w703] -> _
                              shift-left: w702 -> [w716]
                              i -> [w706]
                              stop <- w708 stop-if-true
                              n466 = Decrement(x=w707) -> (x-1=w705:i32)
                              n467 = Subtract(x=w705, y=w706) -> (x-y=w704:i32)
                              n468 = Index Array(array=w716, index=w704) -> (element=w720:cluster{dbl, dbl})
                              n469 = Unbundle(w720) -> (w719:dbl)  [unwired: 1 out]
                              n470 = Unbundle(w715) -> (w718:dbl)  [unwired: 1 out]
                              n471 = Greater?(x=w719, y=w718) -> (0:w717:bool)
                              n472 = case shown="True" w717 {
                                tunnel: w716 -> [w722 w727]
                                tunnel: w704 -> [_ w726]
                                tunnel: w715 -> [_ w725]
                                tunnel: [w722 w724] -> w703
                                tunnel: [TRUE FALSE] -> w708
                                frame False {
                                }
                                frame True {
                                n473 = Replace Array Subset(array=w727, new element=w725, index=w726) -> (w724:cluster{dbl, dbl}[])
                                }
                              }
                              n474 = Bundle By Name(cluster=w712, "Lower Limit"=w703) -> (w713:T1)
                              n475 = call "CRYCurve to Table.vi"("y precision"=w710, "x precision"=w711, "Limit curve In"=w703) -> ("Limit Table"=w714:string[][])  [unwired: 7 in, 1 out]
                              n476 = local write "LoTable_1"(w714) -> ()
                              n477 = local write "Limit Cluster"(w713) -> ()
                              n478 = local write "Plot graphs"(TRUE ("Plot graphs")) -> ()
                            }
                          }
                        }
                      }
                    }
                  }
                  frame False {
                  }
                }
              }
            }
            n479 = property on="Limits Graph" class="XYGraph (strict)"("Cursor.Cursor Position"=w346, "Cursor.Allow Drag"=FALSE) -> ()  [unwired: 2 in, 2 out]
            n480 = local write "Plot graphs"(TRUE ("Plot graphs")) -> ()
          }
        }
      }
      event "Limits Graph": Value Change; "Limits Graph": Autoscale Range Change; "Limits Graph": Scale Range Change; "Limits Graph": Plot Attribute Change {
        n481 = event-data() -> ()  [unwired: 5 out]
        n482 = control-ref of="Limits Graph"() -> (w729:refnum<vi>)
        n483 = call "CRYPaint WaterMark.vi"("Type"="Small", "Graph Ref"=w729) -> ()  [unwired: 10 in]
      }
      event "Type": Value Change {
        n484 = event-data() -> ("OldVal"=w735:u16, "NewVal"=w734:u16)  [unwired: 5 out]
        n485 = Not Equal?(x=w735, y=w734) -> (x != y?=w732:bool)
        n486 = flat-sequence {
          tunnel: w734 -> [w739]
          tunnel: [w739] -> w733
          tunnel: w732 -> [w737]
          tunnel: [w736] -> w731
          tunnel: w730 -> [w736]
          tunnel: w733 -> [w746]
          tunnel: w731 -> [w745]
          frame #0 {
            n487 = local read "Load state"() -> (w738:bool)
            n488 = case shown="False" w738 {
              tunnel: w737 -> [w740 _]
              frame False {
                w741 = enum32{"Single Values", "Curves", "Waveforms"}."Single Values" ("Up_type")
                n489 = case shown="True" w740 {
                  frame False {
                  }
                  frame True {
                    w742 = FALSE ("Visible")
                    w743 = FALSE ("Visible")
                    n490 = property on="UpAlignRst_2" class="Str"("Visible"=w742) -> ()  [unwired: 2 in, 2 out]
                    n491 = property on="LowAlignRst_2" class="Str"("Visible"=w742) -> ()  [unwired: 2 in, 2 out]
                    n492 = local write "Load state"(TRUE ("Load state")) -> ()
                    n493 = property on="UpAlignRst_1" class="Str"("Visible"=w743) -> ()  [unwired: 2 in, 2 out]
                    n494 = property on="DataAlignRst" class="Str"("Visible"=w743) -> ()  [unwired: 2 in, 2 out]
                    n495 = property on="LowAlignRst_1" class="Str"("Visible"=w743) -> ()  [unwired: 2 in, 2 out]
                  }
                }
                n496 = local write "Up_type"(w741) -> ()
                n497 = local write "Lo_type"(w741) -> ()
              }
              frame True {
              }
            }
          }
          frame #1 {
            n498 = local read "Limit Cluster"() -> (w748:T1)
            n499 = Unbundle By Name(w748) -> ("Name"=w747:string)
            n500 = case shown="2" w746 {
              tunnel: w745 -> [w750 w771 w789 _]
              tunnel: w747 -> [w756 w775 w794 _]
              frame 0 {
                w762 = TRUE ("Visible")
                n501 = property on="Sub1 Tab" class="TabCtl (strict)"("Visible"=w762) -> ()  [unwired: 2 in, 2 out]
                n502 = local write "x float"(FALSE ("x float")) -> ()
                n503 = Not(x=w762) -> (.not. x?=w749:bool)
                n504 = property on="Data Value" class="DigNum (strict)"("Visible"=w762) -> ()  [unwired: 2 in, 2 out]
                n505 = property on="Data Table" class="Tbl (strict)"("Visible"=w749) -> ()  [unwired: 2 in, 2 out]
                n506 = call "CRYGet Upper Step Data.vi"("Type In"=enum16{"Curves", "Values", "Results", "WFM"}."Values" ("Type"), "No.VI"=w750) -> ("Value array"=w752:T13)  [unwired: 9 out]
                n507 = property on="Limits Graph" class="XYGraph (strict)"("Visible"=w749) -> ()  [unwired: 2 in, 2 out]
                n508 = property on="Appy limits" class="Bool"("Visible"=w762) -> ()  [unwired: 2 in, 2 out]
                n509 = property on="Y Up Val" class="DigNum (strict)"("Caption.Visible"=w749) -> ()  [unwired: 2 in, 2 out]
                n510 = property on="Y Lo Val" class="DigNum (strict)"("Caption.Visible"=w749) -> ()  [unwired: 2 in, 2 out]
                n511 = property on="Multi value" class="Slide (strict)"("Visible"=w762) -> ()  [unwired: 2 in, 2 out]
                n512 = for {
                  tunnel: w752 -> [w768] mode=indexing
                  tunnel: [w767] -> w757 mode=indexing
                  n513 = Unbundle By Name(w768) -> ("Name"=w767:string)
                }
                n514 = property on="Multi unit" class="Str"("Visible"=w762) -> ()  [unwired: 2 in, 2 out]
                n515 = Search 1D Array(1D array=w757, element=w756) -> (index of element=w759:i32)  [unwired: 1 in]
                n516 = property on="Data Name" class="Ring (strict)"("Strings []"=w757) -> ()  [unwired: 2 in, 2 out]
                n517 = local read "Load state"() -> (w751:bool)
                n518 = Less Than 0?(x=w759) -> (x < 0?=w758:bool)
                n519 = case shown="True" w751 {
                  frame False {
                  }
                  frame True {
                    w766 = u16 1 items=["Individual Points", "Absolute Limits", "Floating Limits", "Floating Data", "Aligned Limits", "Aligned Data"] ("Alignment")
                    n520 = local write "Alignment"(w766) -> ()
                  }
                }
                n521 = property on="Data_xyz" class="Slide (strict)"("Visible"=TRUE, "TextLbls[]"=string[] ["x", "y", "z"] ("Text Labels[]"), "Disabled"=u8 0, "Scale.Text Color"=u32 16777222) -> ()  [unwired: 2 in, 2 out]
                n522 = Select(t=0, s=w758, f=w759) -> (s? t:f=w755:i32)
                n523 = property on="Data Name" class="Ring (strict)"("Val(Sgnl)"=w755) -> ()  [unwired: 2 in, 2 out]
              }
              frame 1, Default {
                w769 = TRUE ("Visible")
                n524 = Not(x=w769) -> (.not. x?=w784:bool)
                n525 = property on="Sub1 Tab" class="TabCtl (strict)"("Visible"=w769) -> ()  [unwired: 2 in, 2 out]
                n526 = property on="Y Up Val" class="DigNum (strict)"("Caption.Visible"=w769) -> ()  [unwired: 2 in, 2 out]
                n527 = property on="Data Value" class="DigNum (strict)"("Visible"=w784) -> ()  [unwired: 2 in, 2 out]
                n528 = property on="Lo tip" class="Str"("Visible"=w784) -> ()  [unwired: 2 in, 2 out]
                n529 = property on="Limits Graph" class="XYGraph (strict)"("Visible"=w769) -> ()  [unwired: 2 in, 2 out]
                n530 = property on="Up tip" class="Str"("Visible"=w784) -> ()  [unwired: 2 in, 2 out]
                n531 = call "CRYGet Upper Step Data.vi"("Type In"=enum16{"Curves", "Values", "Results", "WFM"}."Curves" ("Type"), "No.VI"=w771) -> ("Curve array"=w770:T13)  [unwired: 9 out]
                n532 = property on="Multi value" class="Slide (strict)"("Visible"=w784) -> ()  [unwired: 2 in, 2 out]
                n533 = property on="Y Lo Val" class="DigNum (strict)"("Caption.Visible"=w769) -> ()  [unwired: 2 in, 2 out]
                n534 = property on="Appy limits" class="Bool"("Visible"=w769) -> ()  [unwired: 2 in, 2 out]
                n535 = property on="Single Limit" class="Slide (strict)"("Visible"=w784) -> ()  [unwired: 2 in, 2 out]
                n536 = property on="Multi Limit" class="Slide (strict)"("Visible"=w784) -> ()  [unwired: 2 in, 2 out]
                n537 = for {
                  tunnel: w770 -> [w787] mode=indexing
                  tunnel: [w786] -> w774 mode=indexing
                  n538 = Unbundle By Name(w787) -> ("Name"=w786:string)
                }
                n539 = property on="Data Table" class="Tbl (strict)"("Visible"=w769) -> ()  [unwired: 2 in, 2 out]
                n540 = property on="Multi unit" class="Str"("Visible"=w784) -> ()  [unwired: 2 in, 2 out]
                n541 = Search 1D Array(1D array=w774, element=w775) -> (index of element=w777:i32)  [unwired: 1 in]
                n542 = property on="Data Name" class="Ring (strict)"("Strings []"=w774) -> ()  [unwired: 2 in, 2 out]
                n543 = disable-structure shown="Disabled" {
                  frame Disabled {
                    n544 = local read "Limits_Ring"() -> (w785:u16)
                    n545 = property on="Limits_Ring" class="Ring (strict)"("Val(Sgnl)"=w785) -> ()  [unwired: 2 in, 2 out]
                  }
                  frame Enabled {
                  }
                }
                n546 = Less Than 0?(x=w777) -> (x < 0?=w776:bool)
                n547 = Select(t=0, s=w776, f=w777) -> (s? t:f=w779:i32)
                n548 = property on="Data_xyz" class="Slide (strict)"("Visible"=TRUE, "TextLbls[]"=string[] ["x", "y", "z"] ("Text Labels[]"), "Disabled"=u8 0, "Scale.Text Color"=u32 0) -> ()  [unwired: 2 in, 2 out]
                n549 = property on="Data Name" class="Ring (strict)"("Val(Sgnl)"=w779) -> ()  [unwired: 2 in, 2 out]
                n550 = property on="Data Table" class="Tbl (strict)"("Disabled"=u8 0) -> ()  [unwired: 2 in, 2 out]
              }
              frame 2 {
                w788 = TRUE ("Visible")
                w801 = u16 2 items=["x0", "dx", "y"] ("Data_xyz")
                n551 = Not(x=w788) -> (.not. x?=w800:bool)
                n552 = property on="Sub1 Tab" class="TabCtl (strict)"("Visible"=w788) -> ()  [unwired: 2 in, 2 out]
                n553 = property on="Y Up Val" class="DigNum (strict)"("Caption.Visible"=w788) -> ()  [unwired: 2 in, 2 out]
                n554 = call "CRYGet Upper Step Data.vi"("Type In"=enum16{"Curves", "Values", "Results", "WFM"}."WFM", "No.VI"=w789) -> ("Waveform Array"=w790:T14)  [unwired: 9 out]
                n555 = property on="Data Value" class="DigNum (strict)"("Visible"=w800) -> ()  [unwired: 2 in, 2 out]
                n556 = property on="Lo tip" class="Str"("Visible"=w800) -> ()  [unwired: 2 in, 2 out]
                n557 = property on="Limits Graph" class="XYGraph (strict)"("Visible"=w788) -> ()  [unwired: 2 in, 2 out]
                n558 = property on="Up tip" class="Str"("Visible"=w800) -> ()  [unwired: 2 in, 2 out]
                n559 = property on="Y Lo Val" class="DigNum (strict)"("Caption.Visible"=w788) -> ()  [unwired: 2 in, 2 out]
                n560 = property on="Multi value" class="Slide (strict)"("Visible"=w800) -> ()  [unwired: 2 in, 2 out]
                n561 = property on="Appy limits" class="Bool"("Visible"=w788) -> ()  [unwired: 2 in, 2 out]
                n562 = property on="Single Limit" class="Slide (strict)"("Visible"=w800) -> ()  [unwired: 2 in, 2 out]
                n563 = for {
                  tunnel: w790 -> [w807] mode=indexing
                  tunnel: [w806] -> w795 mode=indexing
                  n564 = Unbundle By Name(w807) -> ("Name"=w806:string)
                }
                n565 = property on="Multi Limit" class="Slide (strict)"("Visible"=w800) -> ()  [unwired: 2 in, 2 out]
                n566 = property on="Data Table" class="Tbl (strict)"("Visible"=w788) -> ()  [unwired: 2 in, 2 out]
                n567 = property on="Multi unit" class="Str"("Visible"=w800) -> ()  [unwired: 2 in, 2 out]
                n568 = property on="Data Name" class="Ring (strict)"("Strings []"=w795) -> ()  [unwired: 2 in, 2 out]
                n569 = Search 1D Array(1D array=w795, element=w794) -> (index of element=w797:i32)  [unwired: 1 in]
                n570 = Less Than 0?(x=w797) -> (x < 0?=w796:bool)
                n571 = Select(t=0, s=w796, f=w797) -> (s? t:f=w793:i32)
                n572 = property on="Data Name" class="Ring (strict)"("Val(Sgnl)"=w793) -> ()  [unwired: 2 in, 2 out]
                n573 = property on="Limits Graph" class="XYGraph (strict)"("XScale.Mapping Mode"=u8 0 ("X Scale.Mapping Mode")) -> ()  [unwired: 2 in, 2 out]
                n574 = property on="Data_xyz" class="Slide (strict)"("Visible"=TRUE, "TextLbls[]"=string[] ["x0", "dx", "y"] ("Text Labels[]"), "Disabled"=u8 2, "Value"=w801, "Scale.Text Color"=u32 16777222) -> ()  [unwired: 2 in, 2 out]
                n575 = property on="Data Table" class="Tbl (strict)"("Disabled"=u8 2) -> ()  [unwired: 2 in, 2 out]
              }
              frame 3 {
                w811 = TRUE ("Visible")
                w812 = 0.0 ("Multi value")
                w808 = FALSE ("Visible")
                w813 = "dB" ("Multi unit")
                n576 = disable-structure shown="Disabled" {
                  frame Disabled {
                    n577 = local write "x float"(FALSE ("x float")) -> ()
                  }
                  frame Enabled {
                  }
                }
                n578 = local write "up single unit"(w813) -> ()
                n579 = property on="Sub1 Tab" class="TabCtl (strict)"("Visible"=w808) -> ()  [unwired: 2 in, 2 out]
                n580 = local write "Multi unit"(w813) -> ()
                n581 = local write "lo single unit"(w813) -> ()
                n582 = property on="Multi value" class="Slide (strict)"("Visible"=w811) -> ()  [unwired: 2 in, 2 out]
                n583 = property on="Y Up Val" class="DigNum (strict)"("Caption.Visible"=w808) -> ()  [unwired: 2 in, 2 out]
                n584 = property on="Limits Graph" class="XYGraph (strict)"("Visible"=w808) -> ()  [unwired: 2 in, 2 out]
                n585 = property on="Multi unit" class="Str"("Visible"=w811) -> ()  [unwired: 2 in, 2 out]
                n586 = property on="Y Lo Val" class="DigNum (strict)"("Caption.Visible"=w808) -> ()  [unwired: 2 in, 2 out]
                n587 = property on="Appy limits" class="Bool"("Visible"=w808) -> ()  [unwired: 2 in, 2 out]
                n588 = local write "Single Limit"(w812) -> ()
                n589 = local write "Multi value"(w812) -> ()
                n590 = local read "Load state"() -> (w809:bool)
                n591 = local read "Limits_Ring"() -> (w810:u16)
                n592 = case shown="True" w809 {
                  frame False {
                  }
                  frame True {
                    w814 = u16 1 items=["Individual Points", "Absolute Limits", "Floating Limits", "Floating Data", "Aligned Limits", "Aligned Data"] ("Alignment")
                    n593 = local write "Alignment"(w814) -> ()
                  }
                }
                n594 = property on="Limits_Ring" class="Ring (strict)"("Val(Sgnl)"=w810) -> ()  [unwired: 2 in, 2 out]
              }
            }
          }
        }
      }
      event "Data Name": Value Change {
        n595 = event-data() -> ("NewVal"=w817:u16)  [unwired: 6 out]
        n596 = local read "Type"() -> (w818:u16)
        n597 = local read "Limit Cluster"() -> (w819:T1)
        n598 = case shown="0, 1, Default" w818 {
          selector: w818 -> [w823 w846]
          tunnel: w817 -> [w827 w847]
          tunnel: w816 -> [w824 w839]
          tunnel: w819 -> [_ w861]
          frame 0, 1, Default {
            w820 = FALSE ("Visible")
            w821 = FALSE ("Visible")
            w825 = T5 {"Row"=0, "Column"=0} ("Selection Size")
            n599 = case shown="0, Default" w823 {
              tunnel: w824 -> [w831 w834]
              tunnel: [w830 w833] -> w822
              frame 0, Default {
                n600 = call "CRYGet Upper Step Data.vi"("Type In"=enum16{"Curves", "Values", "Results", "WFM"}."Values" ("Type"), "No.VI"=w831) -> ("Value array"=w830:T13)  [unwired: 9 out]
              }
              frame 1 {
                n601 = call "CRYGet Upper Step Data.vi"("Type In"=enum16{"Curves", "Values", "Results", "WFM"}."Curves" ("Type"), "No.VI"=w834) -> ("Curve array"=w833:T13)  [unwired: 9 out]
              }
            }
            n602 = property on="UpAlignRst_1" class="Str"("Visible"=w821) -> ()  [unwired: 2 in, 2 out]
            n603 = property on="DataAlignRst" class="Str"("Visible"=w821) -> ()  [unwired: 2 in, 2 out]
            n604 = property on="LowAlignRst_1" class="Str"("Visible"=w821) -> ()  [unwired: 2 in, 2 out]
            n605 = property on="UpAlignRst_2" class="Str"("Visible"=w820) -> ()  [unwired: 2 in, 2 out]
            n606 = property on="LowAlignRst_2" class="Str"("Visible"=w820) -> ()  [unwired: 2 in, 2 out]
            n607 = Index Array(array=w822, index=w827) -> (element=→"Curve and Value":T3)
            n608 = property on="Data Table" class="Tbl (strict)"("Value"=string[][] [], "Selection Size"=w825, "Selection Start"=w825) -> ()  [unwired: 2 in, 2 out]
            n609 = local read "Data_xyz"() -> (w829:u16)
            n610 = property on="Data_xyz" class="Slide (strict)"("Val(Sgnl)"=w829) -> ()  [unwired: 2 in, 2 out]
          }
          frame 2 {
            w836 = FALSE ("Visible")
            w837 = FALSE ("Visible")
            w857 = cluster{dbl, dbl}[] [] ("critical point")
            n611 = call "CRYGet Upper Step Data.vi"("Type In"=enum16{"Curves", "Values", "Results", "WFM"}."WFM", "No.VI"=w839) -> ("Waveform Array"=w838:T14)  [unwired: 9 out]
            n612 = disable-structure shown="Disabled" {
              disable-tunnel: w857 -> [w862 _]
              frame Disabled {
                n613 = global write "CRYLimit edit global.vi" "align ref point"(w862) -> ()
              }
              frame Enabled {
              }
            }
            n614 = property on="Data Name" class="Ring (strict)"() -> ("Strings []"=w848:string[])  [unwired: 2 in, 2 out]
            n615 = global write "CRYLimit edit global.vi" "critical point"(w857) -> ()
            n616 = global write "CRYLimit edit global.vi" "Upper Failed"(w857) -> ()
            n617 = global write "CRYLimit edit global.vi" "Lower Failed"(w857) -> ()
            n618 = Index Array(array=w838, index=w847) -> (element=w844:T2)
            "Wave" <- w844
            n619 = Index Array(array=w848, index=w847) -> (element=w860:string)
            n620 = call "CRYWave Resolve Convert.vi"("Data Wave"=w844) -> ("Curve Out"=w843:cluster{dbl, dbl}[])  [unwired: 10 in]
            n621 = property on="UpAlignRst_1" class="Str"("Visible"=w837) -> ()  [unwired: 2 in, 2 out]
            n622 = property on="DataAlignRst" class="Str"("Visible"=w837) -> ()  [unwired: 2 in, 2 out]
            n623 = property on="LowAlignRst_1" class="Str"("Visible"=w837) -> ()  [unwired: 2 in, 2 out]
            n624 = Unbundle By Name(w844) -> ("X unit"=w859:string, "Y unit"=w858:string, "Y dB ref"=w850:dbl, "Y data"=w849:u16)
            n625 = global write "CRYLimit edit global.vi" "Data"(w843) -> ()
            n626 = property on="UpAlignRst_2" class="Str"("Visible"=w836) -> ()  [unwired: 2 in, 2 out]
            n627 = property on="LowAlignRst_2" class="Str"("Visible"=w836) -> ()  [unwired: 2 in, 2 out]
            n628 = property on="Limits Graph" class="XYGraph (strict)"("YScale.NameLbl.Text"=w858, "XScale.NameLbl.Text"="s" ("X Scale.Name Label.Text")) -> ()  [unwired: 2 in, 2 out]
            n629 = local write "data unit"(w858) -> ()
            n630 = Bundle By Name(cluster=w861, "Name"=w860, "X unit"=w859, "Y unit"=w858, "Y dB ref"=w850, "Y data"=w849, "Type"=w846) -> (w845:T1)
            n631 = Build Array(w859, w858) -> (w851:string[])
            n632 = local read "LoSource"() -> (w854:u16)
            n633 = local write "Limit Cluster"(w845) -> ()
            n634 = local read "UpSource"() -> (w855:u16)
            n635 = Equal To 0?(x=w854) -> (x = 0?=w852:bool)
            n636 = Equal To 0?(x=w855) -> (x = 0?=w853:bool)
            n637 = case shown="True" w852 {
              tunnel: w851 -> [_ w869]
              frame False {
              }
              frame True {
                w871 = "%"
                n638 = Index Array(array=w869, index=0) -> (element=w872:string)
                n639 = Index Array(array=w869, index=1) -> (element=w870:string)
                n640 = property on="LoTable_1" class="Tbl (strict)"("Row Headers[]"=w869) -> ()  [unwired: 2 in, 2 out]
                n641 = Build Array(w872, w871) -> (w874:string[])
                n642 = Build Array(w870, w871) -> (w873:string[])
                n643 = property on="Low y Unit" class="Ring (strict)"("Strings []"=w873) -> ()  [unwired: 2 in, 2 out]
                n644 = property on="Low x Unit" class="Ring (strict)"("Strings []"=w874) -> ()  [unwired: 2 in, 2 out]
              }
            }
            n645 = flat-sequence {
              tunnel: w851 -> [w865]
              tunnel: string[][] [] ("Value") -> [w864]
              tunnel: T5 {"Row"=0, "Column"=0} ("Selection Size") -> [w863]
              frame #0 {
                n646 = property on="Data Table" class="Tbl (strict)"("Row Headers[]"=w865, "Value"=w864, "Selection Size"=w863, "Selection Start"=w863) -> ()  [unwired: 2 in, 2 out]
              }
              frame #1 {
                n647 = local read "Load state"() -> (w866:bool)
                n648 = case shown="True" w866 {
                  frame False {
                    n649 = local write "Plot graphs"(TRUE ("Plot graphs")) -> ()
                  }
                  frame True {
                    n650 = local read "Alignment"() -> (w868:u16)
                    n651 = property on="Alignment" class="Ring (strict)"("Val(Sgnl)"=w868) -> ()  [unwired: 2 in, 2 out]
                  }
                }
              }
            }
            n652 = case shown="True" w853 {
              tunnel: w851 -> [_ w877]
              frame False {
              }
              frame True {
                w879 = "%"
                n653 = property on="UpTable_1" class="Tbl (strict)"("Row Headers[]"=w877) -> ()  [unwired: 2 in, 2 out]
                n654 = Index Array(array=w877, index=0) -> (element=w882:string)
                n655 = Index Array(array=w877, index=1) -> (element=w880:string)
                n656 = Build Array(w880, w879) -> (w878:string[])
                n657 = Build Array(w882, w879) -> (w881:string[])
                n658 = property on="Upp x Unit" class="Ring (strict)"("Strings []"=w881) -> ()  [unwired: 2 in, 2 out]
                n659 = property on="Upp y Unit" class="Ring (strict)"("Strings []"=w878) -> ()  [unwired: 2 in, 2 out]
              }
            }
          }
        }
      }
      event "Data_xyz": Value Change {
        n660 = event-data() -> ("NewVal"=w885:u16)  [unwired: 6 out]
        n661 = local read "Curve and Value"() -> (w886:T3)
        n662 = local read "X Resolution"() -> (w888:u8)
        n663 = local read "Y Resolution"() -> (w887:u8)
        n664 = local read "Limit Cluster"() -> (w889:T1)
        n665 = local read "Type"() -> (w890:u16)
        n666 = case shown="0, Default" w890 {
          selector: w890 -> [w921 w953]
          tunnel: w886 -> [w924 w980]
          tunnel: w885 -> [w923 w979]
          tunnel: w889 -> [w922 w978]
          tunnel: w888 -> [_ w977]
          tunnel: w887 -> [w891 w976]
          frame 0, Default {
            n667 = Unbundle By Name(w924) -> ("Name"=w899:string, "Z data"=w907:u16, "X data"=w908:u16, "Y data"=w913:u16, "Z unit"=w914:string, "X unit"=w919:string, "Y unit"=w920:string, "X dB ref"=w911:dbl, "Y dB ref"=w910:dbl, "Z dB ref"=w909:dbl, "Curve"=w912:cluster{"x":dbl, "y":dbl, "z":dbl}[])
            n668 = Index Array(array=w912) -> (element=w918:cluster{"x":dbl, "y":dbl, "z":dbl})  [unwired: 1 in]
            n669 = Unbundle(w918) -> ("x"=w917:dbl, "y"=w916:dbl, "z"=w915:dbl)
            n670 = case shown="0" w923 {
              tunnel: w919 -> [_ w942 _]
              tunnel: w920 -> [w936 _ _]
              tunnel: w917 -> [_ w943 _]
              tunnel: w916 -> [w937 _ _]
              tunnel: w915 -> [_ _ w947]
              tunnel: [w935 w942 w946] -> w900
              tunnel: [w937 w943 w947] -> w895
              tunnel: w914 -> [_ _ w946]
              tunnel: w913 -> [w934 _ _]
              tunnel: w911 -> [_ w940 _]
              tunnel: w910 -> [w933 _ _]
              tunnel: w909 -> [_ _ w944]
              tunnel: w908 -> [_ w941 _]
              tunnel: w907 -> [_ _ w945]
              tunnel: [w934 w941 w945] -> w906
              tunnel: [w933 w940 w944] -> w905
              frame 1, Default {
                n671 = case shown="0, Default" w934 {
                  tunnel: w936 -> [_ w939]
                  tunnel: ["dB" ("Y unit") w939] -> w935
                  frame 0, Default {
                  }
                  frame 1 {
                  }
                }
              }
              frame 0 {
              }
              frame 2 {
              }
            }
            "Raw DataVal" <- w895
            n672 = local write "Multi unit"(w900) -> ()
            n673 = property on="Multi value" class="Slide (strict)"("Value"=w895, "Scale.Precision"=w891) -> ()  [unwired: 2 in, 2 out]
            n674 = local write "data unit"(w900) -> ()
            n675 = local read "LoSource"() -> (w902:u16)
            n676 = local read "UpSource"() -> (w904:u16)
            n677 = call "CRYRepresent numeric by precission.vi"("Pprecision"=w891, "Numeric In"=w895) -> ("Out Format"=w892:string, "output string"=w893:string, "Numeric Out"=w894:dbl)  [unwired: 7 in]
            n678 = Equal To 0?(x=w902) -> (x = 0?=w901:bool)
            n679 = Equal To 0?(x=w904) -> (x = 0?=w903:bool)
            n680 = Bundle By Name(cluster=w922, "Type"=w921, "Name"=w899, "magn/phase"=w923, "Y unit"=w900, "Y data"=w906, "Y dB ref"=w905, "Tolerance"=u16 1) -> (w898:T1)
            n681 = property on="Data Value" class="DigNum (strict)"("Value"=w894, "FormatString"=w892) -> ()  [unwired: 2 in, 2 out]
            n682 = property class="DigNum (strict)"("NumText.Text"=w893, "FormatString"=w892) -> ()  [unwired: 2 in, 2 out]
            n683 = case shown="True" w903 {
              tunnel: w900 -> [_ w930]
              frame False {
              }
              frame True {
                n684 = Build Array(w930, "%") -> (w931:string[])
                n685 = local write "up single unit"(w930) -> ()
                n686 = property on="Upp y Unit" class="Ring (strict)"("Strings []"=w931) -> ()  [unwired: 2 in, 2 out]
              }
            }
            n687 = case shown="True" w901 {
              tunnel: w900 -> [_ w927]
              frame False {
              }
              frame True {
                n688 = local write "lo single unit"(w927) -> ()
                n689 = Build Array(w927, "%") -> (w928:string[])
                n690 = property on="Low y Unit" class="Ring (strict)"("Strings []"=w928) -> ()  [unwired: 2 in, 2 out]
              }
            }
            n691 = local read "Load state"() -> (w896:bool)
            n692 = local write "Limit Cluster"(w898) -> ()
            n693 = case shown="True" w896 {
              frame False {
                n694 = local write "Plot Multilimit"(TRUE ("Plot graphs")) -> ()
              }
              frame True {
                n695 = local read "Alignment"() -> (w926:u16)
                n696 = property on="Alignment" class="Ring (strict)"("Val(Sgnl)"=w926) -> ()  [unwired: 2 in, 2 out]
              }
            }
          }
          frame 1 {
            w955 = cluster{dbl, dbl}[] [] ("critical point")
            n697 = Unbundle By Name(w980) -> ("Name"=w954:string, "X data"=w971:u16, "Y data"=w972:u16, "Z data"=w970:u16, "X unit"=w975:string, "Y unit"=w974:string, "Z unit"=w969:string, "X dB ref"=w966:dbl, "Y dB ref"=w967:dbl, "Z dB ref"=w968:dbl, "Curve"=w973:cluster{"x":dbl, "y":dbl, "z":dbl}[])
            n698 = case shown="1, Default" w979 {
              tunnel: w975 -> [w1008 w1020 w1030]
              tunnel: w974 -> [w1006 _ _]
              tunnel: w973 -> [w1010 w1022 w1032]
              tunnel: [w1005 w1020 w1028] -> w961
              tunnel: [w1009 w1021 w1031] -> w950
              tunnel: [w1007 w1019 w1029] -> w956
              tunnel: [w1008 w1020 w1030] -> w963
              tunnel: [w1005 w1020 w1028] -> w962
              tunnel: w972 -> [w1004 _ _]
              tunnel: w971 -> [_ w1018 _]
              tunnel: w970 -> [_ _ w1027]
              tunnel: w969 -> [_ _ w1028]
              tunnel: w968 -> [_ _ w1026]
              tunnel: w967 -> [w1003 _ _]
              tunnel: w966 -> [_ w1017 _]
              tunnel: [w1004 w1018 w1027] -> w964
              tunnel: [w1003 w1017 w1026] -> w965
              frame 1, Default {
                n699 = for {
                  tunnel: w1010 -> [w1016] mode=indexing
                  tunnel: [w1014] -> w1009 mode=indexing
                  n700 = Unbundle(w1016) -> ("x"=w1015:dbl, "y"=w1013:dbl)  [unwired: 1 out]
                  n701 = Bundle("x"=w1015, "y"=w1013) -> (w1014:cluster{"x":dbl, "y":dbl})  [unwired: 1 out]
                }
                n702 = case shown="1" w1004 {
                  tunnel: w1006 -> [_ w1012]
                  tunnel: ["dB" ("Y unit") w1012] -> w1005
                  frame 0, Default {
                  }
                  frame 1 {
                  }
                }
                n703 = Build Array(w1008, w1005) -> (w1007:string[])
              }
              frame 0 {
                n704 = for {
                  tunnel: w1022 -> [w1025] mode=indexing
                  tunnel: [w1023] -> w1021 mode=indexing
                  n705 = Unbundle(w1025) -> ("x"=w1024:dbl)  [unwired: 2 out]
                  n706 = Bundle("x"=w1024, "x"=w1024) -> (w1023:cluster{"x":dbl, "x":dbl})  [unwired: 1 out]
                }
                n707 = Build Array(w1020, w1020) -> (w1019:string[])
              }
              frame 2 {
                n708 = for {
                  tunnel: w1032 -> [w1036] mode=indexing
                  tunnel: [w1034] -> w1031 mode=indexing
                  n709 = Unbundle(w1036) -> ("x"=w1035:dbl, "z"=w1033:dbl)  [unwired: 1 out]
                  n710 = Bundle("x"=w1035, "z"=w1033) -> (w1034:cluster{"x":dbl, "z":dbl})  [unwired: 1 out]
                }
                n711 = Build Array(w1030, w1028) -> (w1029:string[])
              }
            }
            n712 = property on="Limits Graph" class="XYGraph (strict)"("XScale.NameLbl.Text"=w963, "YScale.NameLbl.Text"=w962) -> ()  [unwired: 2 in, 2 out]
            n713 = Bundle By Name(cluster=w978, "Type"=w953, "Name"=w954, "magn/phase"=w979, "Y unit"=w961, "Y data"=w964, "Y dB ref"=w965) -> (w952:T1)
            n714 = call "CRYCurve to Table.vi"("y precision"=w976, "Margin"=TRUE, "x precision"=w977, "Limit curve In"=w950) -> ("Limit Table"=w951:string[][])  [unwired: 7 out]
            n715 = property on="Data Table" class="Tbl (strict)"("Row Headers[]"=w956) -> ()  [unwired: 2 in, 2 out]
            n716 = local write "data unit"(w961) -> ()
            n717 = local write "Limit Cluster"(w952) -> ()
            n718 = property on="DataAlignRst" class="Str"("Visible"=FALSE) -> ()  [unwired: 2 in, 2 out]
            n719 = disable-structure shown="Disabled" {
              disable-tunnel: w955 -> [w981 _]
              frame Disabled {
                n720 = global write "CRYLimit edit global.vi" "align ref point"(w981) -> ()
              }
              frame Enabled {
              }
            }
            n721 = global write "CRYLimit edit global.vi" "critical point"(w955) -> ()
            n722 = global write "CRYLimit edit global.vi" "Upper Failed"(w955) -> ()
            n723 = global write "CRYLimit edit global.vi" "Lower Failed"(w955) -> ()
            n724 = local read "LoSource"() -> (w958:u16)
            n725 = local read "UpSource"() -> (w960:u16)
            n726 = flat-sequence {
              tunnel: w951 -> [w983]
              tunnel: w950 -> [w982]
              frame #0 {
                n727 = local write "Data Table"(w983) -> ()
                n728 = global write "CRYLimit edit global.vi" "Data"(w982) -> ()
              }
              frame #1 {
                n729 = local read "Load state"() -> (w984:bool)
                n730 = case shown="False" w984 {
                  frame False {
                    n731 = local write "Plot graphs"(TRUE ("Plot graphs")) -> ()
                  }
                  frame True {
                    n732 = local read "Alignment"() -> (w986:u16)
                    n733 = property on="Alignment" class="Ring (strict)"("Val(Sgnl)"=w986) -> ()  [unwired: 2 in, 2 out]
                  }
                }
              }
            }
            n734 = Equal To 0?(x=w960) -> (x = 0?=w959:bool)
            n735 = Equal To 0?(x=w958) -> (x = 0?=w957:bool)
            n736 = case shown="True" w959 {
              tunnel: w956 -> [_ w995]
              frame False {
              }
              frame True {
                w998 = "%"
                n737 = Index Array(array=w995, index=1) -> (element=w999:string)
                n738 = Index Array(array=w995, index=0) -> (element=w1000:string)
                n739 = Build Array(w999, w998) -> (w997:string[])
                n740 = Build Array(w1000, w998) -> (w996:string[])
                n741 = property on="UpTable_1" class="Tbl (strict)"("Row Headers[]"=w995) -> ()  [unwired: 2 in, 2 out]
                n742 = property on="Upp x Unit" class="Ring (strict)"("Strings []"=w996) -> ()  [unwired: 2 in, 2 out]
                n743 = property on="Upp y Unit" class="Ring (strict)"("Strings []"=w997) -> ()  [unwired: 2 in, 2 out]
              }
            }
            n744 = case shown="True" w957 {
              tunnel: w956 -> [_ w987]
              frame False {
              }
              frame True {
                w989 = "%"
                n745 = property on="LoTable_1" class="Tbl (strict)"("Row Headers[]"=w987) -> ()  [unwired: 2 in, 2 out]
                n746 = Index Array(array=w987, index=0) -> (element=w992:string)
                n747 = Index Array(array=w987, index=1) -> (element=w990:string)
                n748 = Build Array(w992, w989) -> (w991:string[])
                n749 = Build Array(w990, w989) -> (w988:string[])
                n750 = property on="Low y Unit" class="Ring (strict)"("Strings []"=w988) -> ()  [unwired: 2 in, 2 out]
                n751 = property on="Low x Unit" class="Ring (strict)"("Strings []"=w991) -> ()  [unwired: 2 in, 2 out]
              }
            }
          }
        }
      }
      event "UpSource": Value Change {
        n752 = event-data() -> ("OldVal"=w1037:u16, "NewVal"=w1038:u16)  [unwired: 5 out]
        n753 = local read "X Resolution"() -> (w1041:u8)
        n754 = local read "Y Resolution"() -> (w1040:u8)
        n755 = local read "Limit Cluster"() -> (w1042:T1)
        n756 = local read "Limits_Ring"() -> (w1043:u16)
        n757 = local read "Type"() -> (w1044:u16)
        n758 = Bundle By Name(cluster=w1042, "Upper Limit Type"=w1038) -> (w1039:T1)
        n759 = local write "Limit Cluster"(w1039) -> ()
        n760 = case shown="3" w1044 {
          tunnel: w1038 -> [w1046 w1112 w1179 w1240]
          tunnel: w1043 -> [w1049 w1111 w1178 w1239]
          tunnel: w1042 -> [w1048 w1110 w1177 w1238]
          tunnel: w1041 -> [_ w1109 w1176 _]
          tunnel: w1040 -> [w1047 w1108 w1175 w1237]
          tunnel: w1037 -> [w1045 w1107 w1174 w1236]
          frame 0, Default {
            n761 = case shown="0, Default" w1046 {
              selector: w1046 -> [_ w1079]
              tunnel: w1049 -> [w1066 w1090]
              tunnel: w1048 -> [w1067 _]
              tunnel: w1047 -> [w1053 _]
              tunnel: w1045 -> [_ w1078]
              frame 0, Default {
                w1063 = u8 2 ("Disabled")
                w1065 = FALSE ("Visible")
                w1064 = TRUE ("Visible")
                n762 = property on="Up Limit Val" class="DigNum (strict)"("Visible"=w1064) -> ()  [unwired: 2 in, 2 out]
                n763 = property on="Delete Upper" class="Bool"("Disabled"=w1063) -> ()  [unwired: 2 in, 2 out]
                n764 = property on="up single unit" class="Str"("Visible"=w1064) -> ()  [unwired: 2 in, 2 out]
                n765 = property on="Insert Upper" class="Bool"("Disabled"=w1063) -> ()  [unwired: 2 in, 2 out]
                n766 = property on="copy Upper" class="Bool"("Disabled"=u8 0) -> ()  [unwired: 2 in, 2 out]
                n767 = property on="Sub4 Tab" class="TabCtl (strict)"("Visible"=w1064) -> ()  [unwired: 2 in, 2 out]
                n768 = property on="Sub2 Tab" class="TabCtl (strict)"("Visible"=w1064) -> ()  [unwired: 2 in, 2 out]
                n769 = local read "LoSource"() -> (w1056:u16)
                n770 = Unbundle By Name(w1067) -> ("Upper Limit"=w1060:cluster{dbl, dbl}[])
                n771 = property on="Upp x Unit" class="Ring (strict)"("Visible"=w1065) -> ()  [unwired: 2 in, 2 out]
                n772 = property on="X Up Val" class="DigNum (strict)"("Visible"=w1065) -> ()  [unwired: 2 in, 2 out]
                n773 = property on="Sub6 Tab" class="TabCtl (strict)"("Visible"=w1065) -> ()  [unwired: 2 in, 2 out]
                n774 = property on="UpTable_1" class="Tbl (strict)"("Visible"=w1065) -> ()  [unwired: 2 in, 2 out]
                n775 = Equal To 0?(x=w1056) -> (x = 0?=w1055:bool)
                n776 = Index Array(array=w1060) -> (element=w1061:cluster{dbl, dbl})  [unwired: 1 in]
                n777 = local read "data unit"() -> (w1057:string)
                n778 = Unbundle(w1061) -> (w1050:dbl)  [unwired: 1 out]
                n779 = case shown="2" w1066 {
                  tunnel: w1055 -> [_ w1071]
                  frame 0, 1, Default {
                    n780 = property on="Single Limit" class="Slide (strict)"("Disabled"=u8 0, "Visible"=TRUE) -> ()  [unwired: 2 in, 2 out]
                    n781 = property on="Multi Limit" class="Slide (strict)"("Visible"=FALSE) -> ()  [unwired: 2 in, 2 out]
                  }
                  frame 2 {
                    n782 = disable-structure shown="Disabled" {
                      disable-tunnel: w1071 -> [w1074 _]
                      frame Disabled {
                        n783 = Select(t=u8 0 ("Disabled"), s=w1074, f=u8 1) -> (s? t:f=w1075:u8)
                        n784 = property on="Multi Limit" class="Slide (strict)"("Disabled"=w1075) -> ()  [unwired: 2 in, 2 out]
                      }
                      frame Enabled {
                      }
                    }
                    n785 = property on="Multi Limit" class="Slide (strict)"("Visible"=TRUE, "DisabledEnum"=u8 0 ("Disabled")) -> ()  [unwired: 2 in, 2 out]
                  }
                }
                n786 = local write "RawUp Limit"(w1050) -> ()
                n787 = call "CRYRepresent numeric by precission.vi"("Pprecision"=w1053, "Numeric In"=w1050) -> ("Out Format"=w1051:string, "Numeric Out"=w1052:dbl)  [unwired: 7 in, 1 out]
                n788 = local write "up single unit"(w1057) -> ()
                n789 = property on="Up Limit Val" class="DigNum (strict)"("Value"=w1052, "FormatString"=w1051) -> ()  [unwired: 2 in, 2 out]
                n790 = Build Array(w1057, "%") -> (w1058:string[])
                n791 = property on="Upp y Unit" class="Ring (strict)"("Strings []"=w1058) -> ()  [unwired: 2 in, 2 out]
                n792 = local write "Plot Multilimit"(TRUE ("Plot Multilimit")) -> ()
              }
              frame 1 {
                w1088 = TRUE ("Visible")
                w1089 = FALSE ("Visible")
                n793 = case shown="0, Default" w1090 {
                  frame 0, Default {
                    n794 = property on="Single Limit" class="Slide (strict)"("Disabled"=u8 1) -> ()  [unwired: 2 in, 2 out]
                  }
                  frame 2 {
                    n795 = property on="Multi Limit" class="Slide (strict)"("Disabled"=u8 1) -> ()  [unwired: 2 in, 2 out]
                  }
                }
                n796 = property on="Sub4 Tab" class="TabCtl (strict)"("Visible"=w1089) -> ()  [unwired: 2 in, 2 out]
                n797 = property on="UpSingleVal" class="DigNum (strict)"("Visible"=w1088) -> ()  [unwired: 2 in, 2 out]
                n798 = property on="Up_type" class="RadioBtnsControl (strict)"("Visible"=TRUE) -> ("Controls[]"=w1086:refnum<vi>[])  [unwired: 2 in, 2 out]
                n799 = property on="Sub2 Tab" class="TabCtl (strict)"("Visible"=w1089) -> ()  [unwired: 2 in, 2 out]
                n800 = property on="Sub6 Tab" class="TabCtl (strict)"("Visible"=w1088) -> ()  [unwired: 2 in, 2 out]
                n801 = for {
                  tunnel: w1086 -> [w1095] mode=indexing
                  i -> [w1096]
                  n802 = case shown="1, 2" w1096 {
                    tunnel: w1095 -> [w1097 w1101]
                    frame 0, Default {
                      n803 = To More Specific Class(target class=refnum<vi> refnum ("Single Values"), reference=w1097) -> (specific class reference=w1100:refnum<vi>)  [unwired: 1 in, 1 out]
                      n804 = property class="Bool (strict)"(reference=w1100, "Disabled"=u8 0) -> ()  [unwired: 1 in, 2 out]
                    }
                    frame 1, 2 {
                      n805 = To More Specific Class(target class=refnum<vi> refnum ("Single Values"), reference=w1101) -> (specific class reference=w1104:refnum<vi>)  [unwired: 1 in, 1 out]
                      n806 = property class="Bool (strict)"(reference=w1104, "Disabled"=u8 2) -> ()  [unwired: 1 in, 2 out]
                    }
                  }
                }
                n807 = property on="UpTable_2" class="Tbl (strict)"("Visible"=w1089) -> ()  [unwired: 2 in, 2 out]
                n808 = local read "Load state"() -> (w1081:bool)
                n809 = Not Equal?(x=w1078, y=w1079) -> (x != y?=w1082:bool)
                n810 = Or(x=w1082, y=w1081) -> (x .or. y?=w1080:bool)
                n811 = case shown="True" w1080 {
                  frame False {
                    n812 = local write "Plot Multilimit"(TRUE ("Plot Multilimit")) -> ()
                  }
                  frame True {
                    n813 = property on="Up_type" class="RadioBtnsControl (strict)"("Val(Sgnl)"=enum32{"Single Values", "Curves", "Waveforms"}."Single Values" ("Up_type")) -> ()  [unwired: 2 in, 2 out]
                  }
                }
                n814 = property on="Up_xyz" class="Slide (strict)"("Visible"=TRUE, "TextLbls[]"=string[] ["x", "y", "z"] ("Text Labels[]"), "Disabled"=u8 0) -> ()  [unwired: 2 in, 2 out]
              }
            }
          }
          frame 1 {
            w1105 = FALSE ("Visible")
            w1106 = FALSE ("Visible")
            n815 = case shown="0, Default" w1112 {
              selector: w1112 -> [w1114 w1147]
              tunnel: w1111 -> [_ _]
              tunnel: w1110 -> [w1121 _]
              tunnel: w1109 -> [w1119 _]
              tunnel: w1108 -> [w1120 _]
              tunnel: w1107 -> [w1115 w1148]
              frame 0, Default {
                w1126 = FALSE ("Visible")
                w1124 = u8 0 ("Disabled")
                w1118 = TRUE ("Visible")
                n816 = local read "Load state"() -> (w1117:bool)
                n817 = property on="Insert Upper" class="Bool"("Disabled"=w1124) -> ()  [unwired: 2 in, 2 out]
                n818 = property on="Up Limit Val" class="DigNum (strict)"("Visible"=w1126) -> ()  [unwired: 2 in, 2 out]
                n819 = property on="UpTable_1" class="Tbl (strict)"("Visible"=TRUE) -> ()  [unwired: 2 in, 2 out]
                n820 = property on="Upp x Unit" class="Ring (strict)"("Visible"=w1118) -> ()  [unwired: 2 in, 2 out]
                n821 = property on="X Up Val" class="DigNum (strict)"("Visible"=w1118) -> (error out=w1122:errorcluster)  [unwired: 2 in, 1 out]
                n822 = Not Equal?(x=w1115, y=w1114) -> (x != y?=w1116:bool)
                n823 = property on="Delete Upper" class="Bool"("Disabled"=w1124) -> ()  [unwired: 2 in, 2 out]
                n824 = property on="up single unit" class="Str"("Visible"=w1126) -> (error out=w1125:errorcluster)  [unwired: 2 in, 1 out]
                n825 = Or(x=w1116, y=w1117) -> (x .or. y?=w1113:bool)
                n826 = property on="Sub2 Tab" class="TabCtl (strict)"("Visible"=w1118) -> ()  [unwired: 2 in, 2 out]
                n827 = property on="Sub4 Tab" class="TabCtl (strict)"(error in=w1122, "Visible"=w1118) -> ()  [unwired: 1 in, 2 out]
                n828 = property on="copy Upper" class="Bool"("Disabled"=w1124) -> ()  [unwired: 2 in, 2 out]
                n829 = property on="Sub6 Tab" class="TabCtl (strict)"(error in=w1125, "Visible"=w1126) -> ()  [unwired: 1 in, 2 out]
                n830 = case shown="True" w1113 {
                  tunnel: w1121 -> [_ w1130]
                  tunnel: w1120 -> [_ w1129]
                  tunnel: w1119 -> [_ w1128]
                  frame False {
                  }
                  frame True {
                    w1133 = "%"
                    n831 = flat-sequence {
                      tunnel: w1130 -> [w1143]
                      tunnel: w1129 -> [w1142]
                      tunnel: w1128 -> [w1141]
                      frame #0 {
                        n832 = property on="UpTable_1" class="Tbl (strict)"("Value"=string[][] [] ("UpTable_1")) -> ()  [unwired: 2 in, 2 out]
                      }
                      frame #1 {
                        n833 = Unbundle By Name(w1143) -> ("Upper Limit"=w1144:cluster{dbl, dbl}[])
                        n834 = call "CRYCurve to Table.vi"("y precision"=w1142, "x precision"=w1141, "Limit curve In"=w1144) -> ("Limit Table"=w1145:string[][])  [unwired: 1 in, 7 out]
                        n835 = local write "UpTable_1"(w1145) -> ()
                      }
                      frame #2 {
                        n836 = local write "Plot graphs"(TRUE ("Plot graphs")) -> ()
                      }
                    }
                    n837 = property on="Data Table" class="Tbl (strict)"() -> ("Row Headers[]"=w1136:string[])  [unwired: 2 in, 2 out]
                    n838 = Index Array(array=w1136, index=1) -> (element=w1134:string)
                    n839 = Index Array(array=w1136, index=0) -> (element=w1135:string)
                    n840 = Build Array(w1134, w1133) -> (w1132:string[])
                    n841 = Build Array(w1135, w1133) -> (w1131:string[])
                    n842 = property on="UpTable_1" class="Tbl (strict)"("Row Headers[]"=w1136) -> ()  [unwired: 2 in, 2 out]
                    n843 = property on="Upp x Unit" class="Ring (strict)"("Strings []"=w1131) -> ()  [unwired: 2 in, 2 out]
                    n844 = property on="Upp y Unit" class="Ring (strict)"("Strings []"=w1132) -> ()  [unwired: 2 in, 2 out]
                    n845 = local read "Limits_Ring"() -> (w1127:u16)
                    n846 = case shown="0" w1127 {
                      frame 0 {
                        n847 = local write "Load state"(FALSE ("Load state")) -> ()
                      }
                      frame 1, Default {
                      }
                    }
                  }
                }
              }
              frame 1 {
                w1157 = TRUE ("Visible")
                w1156 = FALSE ("Visible")
                n848 = property on="Sub2 Tab" class="TabCtl (strict)"("Visible"=w1156) -> (error out=w1155:errorcluster)  [unwired: 2 in, 1 out]
                n849 = property on="Up_type" class="RadioBtnsControl (strict)"("Visible"=TRUE) -> ("Controls[]"=w1158:refnum<vi>[])  [unwired: 2 in, 2 out]
                n850 = property on="Sub6 Tab" class="TabCtl (strict)"("Visible"=w1157) -> ()  [unwired: 2 in, 2 out]
                n851 = property on="Sub4 Tab" class="TabCtl (strict)"(error in=w1155, "Visible"=w1156) -> ()  [unwired: 1 in, 2 out]
                n852 = for {
                  tunnel: w1158 -> [w1162] mode=indexing
                  i -> [w1163]
                  n853 = case shown="2" w1163 {
                    tunnel: w1162 -> [w1164 w1168]
                    frame 0, 1, Default {
                      n854 = To More Specific Class(target class=refnum<vi> refnum ("Single Values"), reference=w1164) -> (specific class reference=w1167:refnum<vi>)  [unwired: 1 in, 1 out]
                      n855 = property class="Bool (strict)"(reference=w1167, "Disabled"=u8 0) -> ()  [unwired: 1 in, 2 out]
                    }
                    frame 2 {
                      n856 = To More Specific Class(target class=refnum<vi> refnum ("Single Values"), reference=w1168) -> (specific class reference=w1171:refnum<vi>)  [unwired: 1 in, 1 out]
                      n857 = property class="Bool (strict)"(reference=w1171, "Disabled"=u8 2) -> ()  [unwired: 1 in, 2 out]
                    }
                  }
                }
                n858 = property on="UpTable_2" class="Tbl (strict)"("Visible"=w1157) -> ()  [unwired: 2 in, 2 out]
                n859 = property on="UpSingleVal" class="DigNum (strict)"("Visible"=w1156) -> ()  [unwired: 2 in, 2 out]
                n860 = property on="Up_xyz" class="Slide (strict)"("Visible"=TRUE, "TextLbls[]"=string[] ["x", "y", "z"] ("Text Labels[]"), "Disabled"=u8 0) -> ()  [unwired: 2 in, 2 out]
                n861 = local read "Load state"() -> (w1150:bool)
                n862 = Not Equal?(x=w1148, y=w1147) -> (x != y?=w1151:bool)
                n863 = Or(x=w1151, y=w1150) -> (x .or. y?=w1149:bool)
                n864 = case shown="True" w1149 {
                  frame False {
                    n865 = local write "Plot graphs"(TRUE ("Plot graphs")) -> ()
                  }
                  frame True {
                    n866 = local read "Up_type"() -> (w1161:enum32{"Single Values", "Curves", "Waveforms"})
                    n867 = property on="Up_type" class="RadioBtnsControl (strict)"("Val(Sgnl)"=w1161) -> ()  [unwired: 2 in, 2 out]
                  }
                }
              }
            }
            n868 = property on="UpAlignRst_2" class="Str"("Visible"=w1105) -> ()  [unwired: 2 in, 2 out]
            n869 = property on="LowAlignRst_2" class="Str"("Visible"=w1105) -> ()  [unwired: 2 in, 2 out]
            n870 = property on="UpAlignRst_1" class="Str"("Visible"=w1106) -> ()  [unwired: 2 in, 2 out]
            n871 = property on="DataAlignRst" class="Str"("Visible"=w1106) -> ()  [unwired: 2 in, 2 out]
            n872 = property on="LowAlignRst_1" class="Str"("Visible"=w1106) -> ()  [unwired: 2 in, 2 out]
          }
          frame 2 {
            w1172 = FALSE ("Visible")
            w1173 = FALSE ("Visible")
            n873 = case shown="0, Default" w1179 {
              selector: w1179 -> [w1181 w1218]
              tunnel: w1178 -> [_ _]
              tunnel: w1177 -> [w1187 _]
              tunnel: w1176 -> [w1186 _]
              tunnel: w1175 -> [w1185 _]
              tunnel: w1174 -> [w1182 w1217]
              frame 0, Default {
                w1193 = FALSE ("Visible")
                w1190 = u8 0 ("Disabled")
                w1191 = TRUE ("Visible")
                n874 = property on="Up Limit Val" class="DigNum (strict)"("Visible"=w1193) -> ()  [unwired: 2 in, 2 out]
                n875 = property on="copy Upper" class="Bool"("Disabled"=u8 2) -> ()  [unwired: 2 in, 2 out]
                n876 = property on="Insert Upper" class="Bool"("Disabled"=w1190) -> ()  [unwired: 2 in, 2 out]
                n877 = property on="Sub2 Tab" class="TabCtl (strict)"("Visible"=w1191) -> (error out=w1189:errorcluster)  [unwired: 2 in, 1 out]
                n878 = property on="X Up Val" class="DigNum (strict)"("Visible"=w1191) -> ()  [unwired: 2 in, 2 out]
                n879 = local read "Load state"() -> (w1183:bool)
                n880 = property on="up single unit" class="Str"("Visible"=w1193) -> (error out=w1192:errorcluster)  [unwired: 2 in, 1 out]
                n881 = property on="Delete Upper" class="Bool"("Disabled"=w1190) -> ()  [unwired: 2 in, 2 out]
                n882 = property on="Upp x Unit" class="Ring (strict)"("Visible"=w1191) -> ()  [unwired: 2 in, 2 out]
                n883 = property on="Sub4 Tab" class="TabCtl (strict)"(error in=w1189, "Visible"=w1191) -> ()  [unwired: 1 in, 2 out]
                n884 = Not Equal?(x=w1182, y=w1181) -> (x != y?=w1184:bool)
                n885 = property on="Sub6 Tab" class="TabCtl (strict)"(error in=w1192, "Visible"=w1193) -> ()  [unwired: 1 in, 2 out]
                n886 = property on="UpTable_1" class="Tbl (strict)"("Visible"=w1191) -> ()  [unwired: 2 in, 2 out]
                n887 = Or(x=w1184, y=w1183) -> (x .or. y?=w1180:bool)
                n888 = case shown="True" w1180 {
                  tunnel: w1187 -> [_ w1197]
                  tunnel: w1186 -> [_ w1196]
                  tunnel: w1185 -> [_ w1195]
                  frame False {
                  }
                  frame True {
                    w1199 = "%"
                    n889 = flat-sequence {
                      tunnel: w1197 -> [w1210]
                      tunnel: w1196 -> [w1209]
                      tunnel: w1195 -> [w1208]
                      frame #0 {
                        n890 = property on="UpTable_1" class="Tbl (strict)"("Value"=string[][] [] ("UpTable_1")) -> ()  [unwired: 2 in, 2 out]
                      }
                      frame #1 {
                        n891 = Unbundle By Name(w1210) -> ("Upper Limit"=w1211:cluster{dbl, dbl}[])
                        n892 = call "CRYCurve to Table.vi"("y precision"=w1208, "x precision"=w1209, "Limit curve In"=w1211) -> ("Limit Table"=w1212:string[][])  [unwired: 1 in, 7 out]
                        n893 = local write "UpTable_1"(w1212) -> ()
                      }
                      frame #2 {
                        n894 = local write "Plot graphs"(TRUE ("Plot graphs")) -> ()
                      }
                    }
                    n895 = property on="Data Table" class="Tbl (strict)"() -> ("Row Headers[]"=w1203:string[])  [unwired: 2 in, 2 out]
                    n896 = Index Array(array=w1203, index=0) -> (element=w1202:string)
                    n897 = Index Array(array=w1203, index=1) -> (element=w1200:string)
                    n898 = property on="UpTable_1" class="Tbl (strict)"("Row Headers[]"=w1203) -> ()  [unwired: 2 in, 2 out]
                    n899 = Build Array(w1200, w1199) -> (w1198:string[])
                    n900 = Build Array(w1202, w1199) -> (w1201:string[])
                    n901 = property on="Upp x Unit" class="Ring (strict)"("Strings []"=w1201) -> ()  [unwired: 2 in, 2 out]
                    n902 = property on="Upp y Unit" class="Ring (strict)"("Strings []"=w1198) -> ()  [unwired: 2 in, 2 out]
                    n903 = local read "Limits_Ring"() -> (w1194:u16)
                    n904 = case shown="0" w1194 {
                      frame 0 {
                        n905 = local write "Load state"(FALSE ("Load state")) -> ()
                      }
                      frame 1, Default {
                      }
                    }
                  }
                }
              }
              frame 1 {
                w1223 = TRUE ("Visible")
                w1222 = FALSE ("Visible")
                n906 = property on="Up_type" class="RadioBtnsControl (strict)"("Visible"=TRUE) -> ("Controls[]"=w1219:refnum<vi>[])  [unwired: 2 in, 2 out]
                n907 = property on="Sub2 Tab" class="TabCtl (strict)"("Visible"=w1222) -> (error out=w1221:errorcluster)  [unwired: 2 in, 1 out]
                n908 = property on="Sub6 Tab" class="TabCtl (strict)"("Visible"=w1223) -> ()  [unwired: 2 in, 2 out]
                n909 = for {
                  tunnel: w1219 -> [w1226] mode=indexing
                  i -> [w1227]
                  n910 = case shown="1" w1227 {
                    tunnel: w1226 -> [w1228 w1232]
                    frame 0, 2, Default {
                      n911 = To More Specific Class(target class=refnum<vi> refnum ("Single Values"), reference=w1228) -> (specific class reference=w1231:refnum<vi>)  [unwired: 1 in, 1 out]
                      n912 = property class="Bool (strict)"(reference=w1231, "Disabled"=u8 0) -> ()  [unwired: 1 in, 2 out]
                    }
                    frame 1 {
                      n913 = To More Specific Class(target class=refnum<vi> refnum ("Single Values"), reference=w1232) -> (specific class reference=w1235:refnum<vi>)  [unwired: 1 in, 1 out]
                      n914 = property class="Bool (strict)"(reference=w1235, "Disabled"=u8 2) -> ()  [unwired: 1 in, 2 out]
                    }
                  }
                }
                n915 = property on="Sub4 Tab" class="TabCtl (strict)"(error in=w1221, "Visible"=w1222) -> ()  [unwired: 1 in, 2 out]
                n916 = property on="UpTable_2" class="Tbl (strict)"("Visible"=w1223) -> ()  [unwired: 2 in, 2 out]
                n917 = property on="UpSingleVal" class="DigNum (strict)"("Visible"=w1222) -> ()  [unwired: 2 in, 2 out]
                n918 = local read "Load state"() -> (w1215:bool)
                n919 = Not Equal?(x=w1217, y=w1218) -> (x != y?=w1216:bool)
                n920 = Or(x=w1216, y=w1215) -> (x .or. y?=w1214:bool)
                n921 = case shown="True" w1214 {
                  frame False {
                    n922 = local write "Plot graphs"(TRUE ("Plot graphs")) -> ()
                  }
                  frame True {
                    n923 = local read "Up_type"() -> (w1225:enum32{"Single Values", "Curves", "Waveforms"})
                    n924 = property on="Up_type" class="RadioBtnsControl (strict)"("Val(Sgnl)"=w1225) -> ()  [unwired: 2 in, 2 out]
                  }
                }
              }
            }
            n925 = property on="UpAlignRst_1" class="Str"("Visible"=w1172) -> ()  [unwired: 2 in, 2 out]
            n926 = property on="DataAlignRst" class="Str"("Visible"=w1172) -> ()  [unwired: 2 in, 2 out]
            n927 = property on="LowAlignRst_1" class="Str"("Visible"=w1172) -> ()  [unwired: 2 in, 2 out]
            n928 = property on="UpAlignRst_2" class="Str"("Visible"=w1173) -> ()  [unwired: 2 in, 2 out]
            n929 = property on="LowAlignRst_2" class="Str"("Visible"=w1173) -> ()  [unwired: 2 in, 2 out]
          }
          frame 3 {
            n930 = case shown="0, Default" w1240 {
              selector: w1240 -> [_ w1265]
              tunnel: w1239 -> [w1248 w1276]
              tunnel: w1238 -> [w1249 _]
              tunnel: w1237 -> [w1244 _]
              tunnel: w1236 -> [_ w1264]
              frame 0, Default {
                w1251 = u8 2 ("Disabled")
                w1253 = FALSE ("Visible")
                w1252 = TRUE ("Visible")
                w1255 = "dB" ("Multi unit")
                n931 = property on="Insert Upper" class="Bool"("Disabled"=w1251) -> ()  [unwired: 2 in, 2 out]
                n932 = property on="up single unit" class="Str"("Visible"=w1252) -> ()  [unwired: 2 in, 2 out]
                n933 = property on="Up Limit Val" class="DigNum (strict)"("Visible"=w1252) -> ()  [unwired: 2 in, 2 out]
                n934 = property on="UpTable_1" class="Tbl (strict)"("Visible"=w1253) -> ()  [unwired: 2 in, 2 out]
                n935 = property on="X Up Val" class="DigNum (strict)"("Visible"=w1253) -> ()  [unwired: 2 in, 2 out]
                n936 = property on="copy Upper" class="Bool"("Disabled"=u8 0) -> ()  [unwired: 2 in, 2 out]
                n937 = property on="Sub2 Tab" class="TabCtl (strict)"("Visible"=w1252) -> ()  [unwired: 2 in, 2 out]
                n938 = property on="Delete Upper" class="Bool"("Disabled"=w1251) -> ()  [unwired: 2 in, 2 out]
                n939 = property on="Sub6 Tab" class="TabCtl (strict)"("Visible"=w1253) -> ()  [unwired: 2 in, 2 out]
                n940 = property on="Upp x Unit" class="Ring (strict)"("Visible"=w1253) -> ()  [unwired: 2 in, 2 out]
                n941 = property on="Sub4 Tab" class="TabCtl (strict)"("Visible"=w1252) -> ()  [unwired: 2 in, 2 out]
                n942 = local read "LoSource"() -> (w1247:u16)
                n943 = Unbundle By Name(w1249) -> ("Upper Limit"=w1257:cluster{dbl, dbl}[])
                n944 = Equal To 0?(x=w1247) -> (x = 0?=w1246:bool)
                n945 = Index Array(array=w1257) -> (element=w1258:cluster{dbl, dbl})  [unwired: 1 in]
                n946 = Unbundle(w1258) -> (w1241:dbl)  [unwired: 1 out]
                n947 = local write "Multi unit"(w1255) -> ()
                n948 = Build Array(w1255, "%") -> (w1254:string[])
                n949 = call "CRYRepresent numeric by precission.vi"("Pprecision"=w1244, "Numeric In"=w1241) -> ("Out Format"=w1242:string, "Numeric Out"=w1243:dbl)  [unwired: 7 in, 1 out]
                n950 = local write "RawUp Limit"(w1241) -> ()
                n951 = property on="Upp y Unit" class="Ring (strict)"("Strings []"=w1254) -> ()  [unwired: 2 in, 2 out]
                n952 = case shown="2" w1248 {
                  tunnel: w1246 -> [_ w1263]
                  frame 0, Default {
                    n953 = property on="Single Limit" class="Slide (strict)"("Disabled"=u8 0) -> ()  [unwired: 2 in, 2 out]
                  }
                  frame 2 {
                    n954 = Select(t=u8 0 ("Disabled"), s=w1263, f=u8 2) -> (s? t:f=w1260:u8)
                    n955 = property on="Multi Limit" class="Slide (strict)"("Disabled"=w1260) -> ()  [unwired: 2 in, 2 out]
                  }
                }
                n956 = property on="Up Limit Val" class="DigNum (strict)"("Value"=w1243, "FormatString"=w1242) -> ()  [unwired: 2 in, 2 out]
                n957 = local write "up single unit"(w1255) -> ()
                n958 = local write "Plot Multilimit"(TRUE ("Plot Multilimit")) -> ()
              }
              frame 1 {
                w1275 = TRUE ("Visible")
                w1274 = FALSE ("Visible")
                n959 = property on="Up_type" class="RadioBtnsControl (strict)"("Visible"=TRUE) -> ("Controls[]"=w1272:refnum<vi>[])  [unwired: 2 in, 2 out]
                n960 = case shown="2" w1276 {
                  frame 0, Default {
                    n961 = property on="Single Limit" class="Slide (strict)"("Disabled"=u8 1) -> ()  [unwired: 2 in, 2 out]
                  }
                  frame 2 {
                    n962 = property on="Multi Limit" class="Slide (strict)"("Disabled"=u8 1) -> ()  [unwired: 2 in, 2 out]
                  }
                }
                n963 = property on="Sub4 Tab" class="TabCtl (strict)"("Visible"=w1274) -> ()  [unwired: 2 in, 2 out]
                n964 = property on="Sub2 Tab" class="TabCtl (strict)"("Visible"=w1274) -> ()  [unwired: 2 in, 2 out]
                n965 = property on="UpTable_2" class="Tbl (strict)"("Visible"=w1274) -> ()  [unwired: 2 in, 2 out]
                n966 = for {
                  tunnel: w1272 -> [w1281] mode=indexing
                  i -> [w1282]
                  n967 = case shown="0, Default" w1282 {
                    tunnel: w1281 -> [w1283 w1287]
                    frame 0, Default {
                      n968 = To More Specific Class(target class=refnum<vi> refnum ("Single Values"), reference=w1283) -> (specific class reference=w1286:refnum<vi>)  [unwired: 1 in, 1 out]
                      n969 = property class="Bool (strict)"(reference=w1286, "Disabled"=u8 0) -> ()  [unwired: 1 in, 2 out]
                    }
                    frame 1, 2 {
                      n970 = To More Specific Class(target class=refnum<vi> refnum ("Single Values"), reference=w1287) -> (specific class reference=w1290:refnum<vi>)  [unwired: 1 in, 1 out]
                      n971 = property class="Bool (strict)"(reference=w1290, "Disabled"=u8 2) -> ()  [unwired: 1 in, 2 out]
                    }
                  }
                }
                n972 = property on="UpSingleVal" class="DigNum (strict)"("Visible"=w1275) -> ()  [unwired: 2 in, 2 out]
                n973 = property on="Sub6 Tab" class="TabCtl (strict)"("Visible"=w1275) -> ()  [unwired: 2 in, 2 out]
                n974 = property on="Up_xyz" class="Slide (strict)"("Visible"=TRUE, "Disabled"=u8 0, "TextLbls[]"=string[] ["x", "y", "z"] ("Text Labels[]")) -> ()  [unwired: 2 in, 2 out]
                n975 = local read "Load state"() -> (w1267:bool)
                n976 = Not Equal?(x=w1264, y=w1265) -> (x != y?=w1268:bool)
                n977 = Or(x=w1268, y=w1267) -> (x .or. y?=w1266:bool)
                n978 = case shown="True" w1266 {
                  frame False {
                    n979 = local write "Plot Multilimit"(TRUE ("Plot Multilimit")) -> ()
                  }
                  frame True {
                    n980 = property on="Up_type" class="RadioBtnsControl (strict)"("Val(Sgnl)"=enum32{"Single Values", "Curves", "Waveforms"}."Single Values" ("Up_type")) -> ()  [unwired: 2 in, 2 out]
                  }
                }
              }
            }
          }
        }
      }
      event "Up_type": Value Change {
        n981 = event-data() -> ("NewVal"=w1292:enum32{"Single Values", "Curves", "Waveforms"})  [unwired: 6 out]
        n982 = case shown="\"Waveforms\"" w1292 {
          tunnel: w1291 -> [w1304 w1315 w1327]
          tunnel: [w1305 w1317 w1328] -> w1294
          frame "Single Values", Default {
            n983 = call "CRYGet Upper Step Data.vi"("Type In"=enum16{"Curves", "Values", "Results", "WFM"}."Values", "No.VI"=w1304) -> ("Value array"=w1302:T13)  [unwired: 9 out]
            n984 = property on="Up_xyz" class="Slide (strict)"("Visible"=TRUE, "TextLbls[]"=string[] ["x", "y", "z"] ("Text Labels[]"), "Disabled"=u8 0, "Scale.Text Color"=u32 0) -> ()  [unwired: 2 in, 2 out]
            n985 = for {
              tunnel: w1302 -> [w1312] mode=indexing
              tunnel: [w1311] -> w1305 mode=indexing
              n986 = Unbundle By Name(w1312) -> ("Name"=w1311:string)
            }
            n987 = property on="UpTable_2" class="Tbl (strict)"("Disabled"=u8 0) -> ()  [unwired: 2 in, 2 out]
          }
          frame "Curves" {
            n988 = call "CRYGet Upper Step Data.vi"("Type In"=enum16{"Curves", "Values", "Results", "WFM"}."Curves", "No.VI"=w1315) -> ("Curve array"=w1313:T13)  [unwired: 9 out]
            n989 = property on="Up_xyz" class="Slide (strict)"("Visible"=TRUE, "TextLbls[]"=string[] ["x", "y", "z"] ("Text Labels[]"), "Disabled"=u8 0, "Scale.Text Color"=u32 0) -> ()  [unwired: 2 in, 2 out]
            n990 = for {
              tunnel: w1313 -> [w1324] mode=indexing
              tunnel: [w1323] -> w1317 mode=indexing
              n991 = Unbundle By Name(w1324) -> ("Name"=w1323:string)
            }
            n992 = property on="UpTable_2" class="Tbl (strict)"("Disabled"=u8 0) -> ()  [unwired: 2 in, 2 out]
            n993 = property on="UpTable_2" class="Tbl (strict)"("Value"=string[][] [] ("Upper limit Table")) -> ()  [unwired: 2 in, 2 out]
          }
          frame "Waveforms" {
            w1334 = u8 2 ("Disabled")
            n994 = call "CRYGet Upper Step Data.vi"("Type In"=enum16{"Curves", "Values", "Results", "WFM"}."WFM", "No.VI"=w1327) -> ("Waveform Array"=w1325:T14)  [unwired: 9 out]
            n995 = property on="Up_xyz" class="Slide (strict)"("Visible"=TRUE, "TextLbls[]"=string[] ["x0", "dx", "y"] ("Text Labels[]"), "Disabled"=w1334, "Value"=w1334, "Scale.Text Color"=u32 1193471) -> ()  [unwired: 2 in, 2 out]
            n996 = for {
              tunnel: w1325 -> [w1336] mode=indexing
              tunnel: [w1335] -> w1328 mode=indexing
              n997 = Unbundle By Name(w1336) -> ("Name"=w1335:string)
            }
            n998 = property on="UpTable_2" class="Tbl (strict)"("Disabled"=u8 2, "Value"=string[][] [] ("Upper limit Table")) -> ()  [unwired: 2 in, 2 out]
          }
        }
        n999 = local read "Limit Cluster"() -> (w1301:T1)
        n1000 = Unbundle By Name(w1301) -> ("Curve Names"=w1300:string[])
        n1001 = property on="Up Cur Name" class="Ring (strict)"("Strings []"=w1294) -> ()  [unwired: 2 in, 2 out]
        n1002 = Index Array(array=w1300, index=0) -> (element=w1295:string)
        n1003 = Search 1D Array(1D array=w1294, element=w1295) -> (index of element=w1296:i32)  [unwired: 1 in]
        n1004 = Less Than 0?(x=w1296) -> (x < 0?=w1298:bool)
        n1005 = Select(t=0, s=w1298, f=w1296) -> (s? t:f=w1293:i32)
        n1006 = property on="Up Cur Name" class="Ring (strict)"("Val(Sgnl)"=w1293) -> ()  [unwired: 2 in, 2 out]
      }
      event "Up Cur Name": Value Change {
        w1338 = FALSE ("Visible")
        w1339 = FALSE ("Visible")
        n1007 = event-data() -> ("NewVal"=w1340:u16)  [unwired: 6 out]
        n1008 = local read "Up_type"() -> (w1342:enum32{"Single Values", "Curves", "Waveforms"})
        n1009 = Equal?(x=w1342, y=u16 2) -> (x = y?=w1350:bool)
        n1010 = case shown="True" w1350 {
          tunnel: w1340 -> [w1364 w1379]
          tunnel: w1342 -> [w1360 _]
          tunnel: w1337 -> [w1362 w1374]
          tunnel: [w1365 w1381] -> w1346
          frame False {
            n1011 = case shown="\"Single Values\", Default" w1360 {
              tunnel: w1362 -> [w1369 w1372]
              tunnel: [w1368 w1371] -> w1361
              frame "Single Values", Default {
                n1012 = call "CRYGet Upper Step Data.vi"("Type In"=enum16{"Curves", "Values", "Results", "WFM"}."Values" ("Type"), "No.VI"=w1369) -> ("Value array"=w1368:T13)  [unwired: 9 out]
              }
              frame "Curves" {
                n1013 = call "CRYGet Upper Step Data.vi"("Type In"=enum16{"Curves", "Values", "Results", "WFM"}."Curves" ("Type"), "No.VI"=w1372) -> ("Curve array"=w1371:T13)  [unwired: 9 out]
              }
            }
            n1014 = Index Array(array=w1361, index=w1364) -> (element=→"Up Curve and Value":T3)
            n1015 = property on="Up Cur Name" class="Ring (strict)"() -> ("Strings []"=w1363:string[])  [unwired: 2 in, 2 out]
            n1016 = local read "Up_xyz"() -> (w1367:u16)
            n1017 = Index Array(array=w1363, index=w1364) -> (element=w1365:string)
            n1018 = property on="Up_xyz" class="Slide (strict)"("Val(Sgnl)"=w1367) -> ()  [unwired: 2 in, 2 out]
          }
          frame True {
            n1019 = call "CRYGet Upper Step Data.vi"("Type In"=enum16{"Curves", "Values", "Results", "WFM"}."WFM", "No.VI"=w1374) -> ("Waveform Array"=w1375:T14)  [unwired: 9 out]
            n1020 = property on="Up Cur Name" class="Ring (strict)"() -> ("Strings []"=w1380:string[])  [unwired: 2 in, 2 out]
            n1021 = Index Array(array=w1375, index=w1379) -> (element=w1382:T2)
            "Up Wave" <- w1382
            n1022 = Index Array(array=w1380, index=w1379) -> (element=w1381:string)
            n1023 = Unbundle By Name(w1382) -> ("X unit"=w1385:string, "Y unit"=w1384:string)
            n1024 = local write "Plot graphs"(TRUE ("Plot graphs")) -> ()
            n1025 = local write "Load state"(FALSE ("Load state")) -> ()
            n1026 = local write "up_unit"(w1384) -> ()
            n1027 = Build Array(w1385, w1384) -> (w1383:string[])
            n1028 = property on="UpTable_2" class="Tbl (strict)"("Row Headers[]"=w1383) -> ()  [unwired: 2 in, 2 out]
          }
        }
        n1029 = property on="UpAlignRst_1" class="Str"("Visible"=w1339) -> ()  [unwired: 2 in, 2 out]
        n1030 = property on="DataAlignRst" class="Str"("Visible"=w1339) -> ()  [unwired: 2 in, 2 out]
        n1031 = property on="LowAlignRst_1" class="Str"("Visible"=w1339) -> ()  [unwired: 2 in, 2 out]
        n1032 = property on="UpAlignRst_2" class="Str"("Visible"=w1338) -> ()  [unwired: 2 in, 2 out]
        n1033 = property on="LowAlignRst_2" class="Str"("Visible"=w1338) -> ()  [unwired: 2 in, 2 out]
        n1034 = local read "Limit Cluster"() -> (w1344:T1)
        n1035 = Unbundle By Name(w1344) -> ("Curve Names"=w1345:string[])
        n1036 = Index Array(array=w1345, index=0) -> (element=w1348:string)
        n1037 = Empty String/Path?(string/path=w1348) -> (empty?=w1347:bool)
        n1038 = case shown="True" w1347 {
          tunnel: w1346 -> [w1353 w1357]
          tunnel: w1345 -> [w1355 w1358]
          tunnel: [w1352 w1356] -> w1343
          frame False {
            n1039 = Replace Array Subset(array=w1355, new element=w1353, index=0) -> (w1352:string[])
          }
          frame True {
            n1040 = Insert Into Array(array=w1358, index=0, new element=w1357) -> (w1356:string[])
          }
        }
        n1041 = Bundle By Name(cluster=w1344, "Data Selection Upper"=w1342, "Curve Names"=w1343) -> (w1341:T1)
        n1042 = local write "Limit Cluster"(w1341) -> ()
      }
      event "Up_xyz": Value Change {
        n1043 = event-data() -> ("OldVal"=w1388:u16, "NewVal"=w1387:u16)  [unwired: 5 out]
        n1044 = Not Equal?(x=w1388, y=w1387) -> (x != y?=w1386:bool)
        n1045 = local read "Up Curve and Value"() -> (w1390:T3)
        n1046 = case shown="True" w1386 {
          frame False {
          }
          frame True {
            w1397 = FALSE ("Visible")
            n1047 = property on="UpAlignRst_2" class="Str"("Visible"=w1397) -> ()  [unwired: 2 in, 2 out]
            n1048 = property on="UpAlignRst_1" class="Str"("Visible"=w1397) -> ()  [unwired: 2 in, 2 out]
          }
        }
        n1049 = local read "X Resolution"() -> (w1394:u8)
        n1050 = local read "Y Resolution"() -> (w1393:u8)
        n1051 = local read "Limits_Ring"() -> (w1392:u16)
        n1052 = local read "Up_type"() -> (w1395:enum32{"Single Values", "Curves", "Waveforms"})
        n1053 = local read "Type"() -> (w1396:u16)
        n1054 = case shown="0, 3" w1396 {
          selector: w1396 -> [w1402 _ _]
          tunnel: w1390 -> [w1403 w1441 w1519]
          tunnel: w1387 -> [w1401 w1440 w1518]
          tunnel: w1395 -> [_ w1439 w1517]
          tunnel: w1394 -> [_ w1436 w1516]
          tunnel: w1393 -> [w1399 w1435 w1515]
          tunnel: w1392 -> [_ _ w1514]
          frame 0, 3 {
            n1055 = Unbundle By Name(w1403) -> ("Y data"=w1404:u16, "X unit"=w1412:string, "Y unit"=w1413:string, "Curve"=w1411:cluster{"x":dbl, "y":dbl, "z":dbl}[])
            n1056 = Index Array(array=w1411, index=0) -> (element=w1409:cluster{"x":dbl, "y":dbl, "z":dbl})
            n1057 = Equal To 0?(x=w1402) -> (x = 0?=w1405:bool)
            n1058 = Unbundle(w1409) -> ("x"=w1408:dbl, "y"=w1407:dbl, "z"=w1406:dbl)
            n1059 = case shown="0" w1401 {
              tunnel: w1412 -> [_ w1429 _]
              tunnel: w1413 -> [w1423 _ _]
              tunnel: w1408 -> [_ w1428 _]
              tunnel: w1407 -> [w1425 _ _]
              tunnel: w1406 -> [_ _ w1430]
              tunnel: [w1425 w1428 w1430] -> w1398
              tunnel: [w1422 w1429 "deg." ("new element/subarray")] -> w1400
              tunnel: w1404 -> [w1424 _ _]
              frame 1, Default {
                n1060 = case shown="0, Default" w1424 {
                  tunnel: w1423 -> [_ w1427]
                  tunnel: ["dB" ("Y unit") w1427] -> w1422
                  frame 0, Default {
                  }
                  frame 1 {
                  }
                }
              }
              frame 0 {
              }
              frame 2 {
              }
            }
            n1061 = flat-sequence {
              tunnel: w1405 -> [w1419]
              tunnel: w1400 -> [w1416]
              tunnel: w1399 -> [w1415]
              tunnel: w1398 -> [w1414]
              frame #0 {
                n1062 = property on="UpSingleVal" class="DigNum (strict)"("Value"=w1414, "Precision"=w1415) -> ()  [unwired: 2 in, 2 out]
                n1063 = local write "up_unit"(w1416) -> ()
                n1064 = Select(t=w1416, s=w1419, f="dB") -> (s? t:f=w1417:string)
                n1065 = local write "Multi unit"(w1417) -> ()
              }
              frame #1 {
                n1066 = local write "Plot Multilimit"(TRUE ("Plot Multilimit")) -> ()
                n1067 = local write "Load state"(FALSE ("Load state")) -> ()
              }
            }
          }
          frame 1, Default {
            n1068 = case shown="\"Curves\", Default" w1439 {
              tunnel: w1440 -> [w1458 w1487]
              tunnel: w1441 -> [w1451 w1483]
              tunnel: [w1450 w1482] -> w1432
              tunnel: [w1449 w1481] -> w1434
              tunnel: [w1447 w1479] -> w1433
              frame "Single Values" {
                n1069 = Unbundle By Name(w1451) -> ("Y data"=w1448:u16, "X unit"=w1454:string, "Y unit"=w1453:string, "Curve"=w1461:cluster{"x":dbl, "y":dbl, "z":dbl}[])
                n1070 = Index Array(array=w1461, index=0) -> (element=w1459:cluster{"x":dbl, "y":dbl, "z":dbl})
                n1071 = Unbundle(w1459) -> ("x"=w1457:dbl, "y"=w1456:dbl, "z"=w1455:dbl)
                n1072 = case shown="1" w1458 {
                  tunnel: w1457 -> [w1464 w1471 w1478]
                  tunnel: w1456 -> [_ w1470 _]
                  tunnel: w1455 -> [_ _ w1474]
                  tunnel: w1454 -> [w1463 w1468 w1476]
                  tunnel: w1453 -> [_ w1466 _]
                  tunnel: [w1463 w1468 w1476] -> w1447
                  tunnel: [w1463 w1465 "deg." ("new element/subarray")] -> w1450
                  tunnel: [w1462 w1469 w1477] -> w1452
                  tunnel: w1448 -> [_ w1467 _]
                  frame 0, Default {
                    n1073 = Bundle("x"=w1464, "x"=w1464) -> (w1462:cluster{"x":dbl, "x":dbl})  [unwired: 1 out]
                  }
                  frame 1 {
                    n1074 = Bundle("x"=w1471, "y"=w1470) -> (w1469:cluster{"x":dbl, "y":dbl})  [unwired: 1 out]
                    n1075 = case shown="0, Default" w1467 {
                      tunnel: w1466 -> [_ w1473]
                      tunnel: ["dB" ("Y unit") w1473] -> w1465
                      frame 0, Default {
                      }
                      frame 1 {
                      }
                    }
                  }
                  frame 2 {
                    n1076 = Bundle("x"=w1478, "z"=w1474) -> (w1477:cluster{"x":dbl, "z":dbl})  [unwired: 1 out]
                  }
                }
                n1077 = Build Array(w1452) -> (w1449:cluster{"x":dbl, "z":dbl}[])
              }
              frame "Curves", Default {
                n1078 = Unbundle By Name(w1483) -> ("Y data"=w1480:u16, "X unit"=w1486:string, "Y unit"=w1485:string, "Curve"=w1484:cluster{"x":dbl, "y":dbl, "z":dbl}[])
                n1079 = case shown="1, Default" w1487 {
                  tunnel: w1486 -> [w1492 w1500 w1508]
                  tunnel: w1485 -> [w1489 _ _]
                  tunnel: w1484 -> [w1493 w1502 w1509]
                  tunnel: [w1492 w1500 w1508] -> w1479
                  tunnel: [w1488 w1500 "deg." ("new element/subarray")] -> w1482
                  tunnel: [w1491 w1501 w1506] -> w1481
                  tunnel: w1480 -> [w1490 _ _]
                  frame 1, Default {
                    n1080 = for {
                      tunnel: w1493 -> [w1496] mode=indexing
                      tunnel: [w1498] -> w1491 mode=indexing
                      n1081 = Unbundle(w1496) -> ("x"=w1499:dbl, "y"=w1497:dbl)  [unwired: 1 out]
                      n1082 = Bundle("x"=w1499, "y"=w1497) -> (w1498:cluster{"x":dbl, "y":dbl})  [unwired: 1 out]
                    }
                    n1083 = case shown="1" w1490 {
                      tunnel: w1489 -> [_ w1495]
                      tunnel: ["dB" ("Y unit") w1495] -> w1488
                      frame 0, Default {
                      }
                      frame 1 {
                      }
                    }
                  }
                  frame 0 {
                    n1084 = for {
                      tunnel: w1502 -> [w1503] mode=indexing
                      tunnel: [w1504] -> w1501 mode=indexing
                      n1085 = Unbundle(w1503) -> ("x"=w1505:dbl)  [unwired: 2 out]
                      n1086 = Bundle("x"=w1505, "x"=w1505) -> (w1504:cluster{"x":dbl, "x":dbl})  [unwired: 1 out]
                    }
                  }
                  frame 2 {
                    n1087 = for {
                      tunnel: w1509 -> [w1511] mode=indexing
                      tunnel: [w1512] -> w1506 mode=indexing
                      n1088 = Unbundle(w1511) -> ("x"=w1513:dbl, "z"=w1510:dbl)  [unwired: 1 out]
                      n1089 = Bundle("x"=w1513, "z"=w1510) -> (w1512:cluster{"x":dbl, "z":dbl})  [unwired: 1 out]
                    }
                  }
                }
              }
            }
            "Up Limit Data" <- w1434
            n1090 = call "CRYCurve to Table.vi"("y precision"=w1435, "x precision"=w1436, "Limit curve In"=w1434) -> ("Limit Table"=w1437:string[][])  [unwired: 1 in, 7 out]
            n1091 = Build Array(w1433, w1432) -> (w1438:string[])
            n1092 = flat-sequence {
              tunnel: w1438 -> [w1444]
              tunnel: w1437 -> [w1443]
              tunnel: w1432 -> [w1442]
              frame #0 {
                n1093 = local write "up_unit"(w1442) -> ()
                n1094 = property on="UpTable_2" class="Tbl (strict)"("Value"=w1443, "Row Headers[]"=w1444) -> ()  [unwired: 2 in, 2 out]
              }
              frame #1 {
                n1095 = local write "Plot graphs"(TRUE ("Plot graphs")) -> ()
                n1096 = local write "Load state"(FALSE ("Load state")) -> ()
              }
            }
          }
          frame 2 {
            n1097 = case shown="\"Single Values\", Default" w1517 {
              tunnel: w1516 -> [w1527 _]
              tunnel: w1515 -> [w1529 _]
              tunnel: w1518 -> [w1528 _]
              tunnel: w1519 -> [w1526 _]
              tunnel: w1514 -> [_ _]
              frame "Single Values", Default {
                n1098 = Unbundle By Name(w1526) -> ("Y data"=w1524:u16, "X unit"=w1532:string, "Y unit"=w1531:string, "Curve"=w1538:cluster{"x":dbl, "y":dbl, "z":dbl}[])
                n1099 = Index Array(array=w1538, index=0) -> (element=w1536:cluster{"x":dbl, "y":dbl, "z":dbl})
                n1100 = Unbundle(w1536) -> ("x"=w1535:dbl, "y"=w1534:dbl, "z"=w1533:dbl)
                n1101 = case shown="1" w1528 {
                  tunnel: w1535 -> [w1545 w1552 w1559]
                  tunnel: w1534 -> [_ w1551 _]
                  tunnel: w1533 -> [_ _ w1555]
                  tunnel: w1532 -> [w1544 w1549 w1557]
                  tunnel: w1531 -> [_ w1547 _]
                  tunnel: [w1544 w1549 w1557] -> w1525
                  tunnel: [w1544 w1546 "deg." ("new element/subarray")] -> w1523
                  tunnel: [w1543 w1550 w1558] -> w1530
                  tunnel: w1524 -> [_ w1548 _]
                  frame 0, Default {
                    n1102 = Bundle("x"=w1545, "x"=w1545) -> (w1543:cluster{"x":dbl, "x":dbl})  [unwired: 1 out]
                  }
                  frame 1 {
                    n1103 = Bundle("x"=w1552, "y"=w1551) -> (w1550:cluster{"x":dbl, "y":dbl})  [unwired: 1 out]
                    n1104 = case shown="0, Default" w1548 {
                      tunnel: w1547 -> [_ w1554]
                      tunnel: ["dB" ("Y unit") w1554] -> w1546
                      frame 0, Default {
                      }
                      frame 1 {
                      }
                    }
                  }
                  frame 2 {
                    n1105 = Bundle("x"=w1559, "z"=w1555) -> (w1558:cluster{"x":dbl, "z":dbl})  [unwired: 1 out]
                  }
                }
                n1106 = Build Array(w1530) -> (w1520:cluster{"x":dbl, "z":dbl}[])
                n1107 = Build Array(w1525, w1523) -> (w1521:string[])
                n1108 = local write "up_unit"(w1523) -> ()
                n1109 = call "CRYCurve to Table.vi"("y precision"=w1529, "x precision"=w1527, "Limit curve In"=w1520) -> ("Limit Table"=w1522:string[][])  [unwired: 1 in, 7 out]
                n1110 = local write "Up Limit Data"(w1520) -> ()
                n1111 = flat-sequence {
                  tunnel: w1522 -> [w1540]
                  tunnel: w1521 -> [w1539]
                  frame #0 {
                    n1112 = property on="UpTable_2" class="Tbl (strict)"("Value"=w1540, "Row Headers[]"=w1539) -> ()  [unwired: 2 in, 2 out]
                  }
                  frame #1 {
                    n1113 = local write "Plot graphs"(TRUE ("Plot graphs")) -> ()
                    n1114 = local write "Load state"(FALSE ("Load state")) -> ()
                  }
                }
              }
              frame "Waveforms" {
              }
            }
          }
        }
        n1115 = local read "Limit Cluster"() -> (w1391:T1)
        n1116 = Bundle By Name(cluster=w1391, "Lim Curve axis up"=w1387) -> (w1389:T1)
        n1117 = local write "Limit Cluster"(w1389) -> ()
      }
      event "LoSource": Value Change {
        n1118 = event-data() -> ("OldVal"=w1560:u16, "NewVal"=w1561:u16)  [unwired: 5 out]
        n1119 = local read "Limit Cluster"() -> (w1565:T1)
        n1120 = local read "X Resolution"() -> (w1564:u8)
        n1121 = local read "Y Resolution"() -> (w1563:u8)
        n1122 = local read "Limits_Ring"() -> (w1566:u16)
        n1123 = local read "Type"() -> (w1567:u16)
        n1124 = Bundle By Name(cluster=w1565, "Lower Limit Type"=w1561) -> (w1562:T1)
        n1125 = local write "Limit Cluster"(w1562) -> ()
        n1126 = case shown="3" w1567 {
          tunnel: w1561 -> [w1572 w1630 w1692 w1752]
          tunnel: w1566 -> [w1571 _ _ w1751]
          tunnel: w1565 -> [w1570 w1629 w1691 w1750]
          tunnel: w1564 -> [_ w1628 w1690 _]
          tunnel: w1563 -> [w1569 w1627 w1689 w1749]
          tunnel: w1560 -> [w1568 w1626 w1688 w1748]
          frame 0, Default {
            n1127 = case shown="0, Default" w1572 {
              selector: w1572 -> [_ w1598]
              tunnel: w1571 -> [w1590 w1609]
              tunnel: w1570 -> [w1591 _]
              tunnel: w1569 -> [w1576 _]
              tunnel: w1568 -> [_ w1597]
              frame 0, Default {
                w1581 = u8 2 ("Disabled")
                w1582 = FALSE ("Visible")
                w1583 = TRUE ("Visible")
                n1128 = property on="Insert Lower" class="Bool"("Disabled"=w1581) -> ()  [unwired: 2 in, 2 out]
                n1129 = property on="Delete Lower" class="Bool"("Disabled"=w1581) -> ()  [unwired: 2 in, 2 out]
                n1130 = property on="copy Lower" class="Bool"("Disabled"=u8 0) -> ()  [unwired: 2 in, 2 out]
                n1131 = property on="Sub5 Tab" class="TabCtl (strict)"("Visible"=w1583) -> ()  [unwired: 2 in, 2 out]
                n1132 = property on="Lo Limit Val" class="DigNum (strict)"("Visible"=w1583) -> ()  [unwired: 2 in, 2 out]
                n1133 = property on="Sub3 Tab" class="TabCtl (strict)"("Visible"=w1583) -> ()  [unwired: 2 in, 2 out]
                n1134 = property on="lo single unit" class="Str"("Visible"=w1583) -> ()  [unwired: 2 in, 2 out]
                n1135 = local read "UpSource"() -> (w1579:u16)
                n1136 = property on="Sub7 Tab" class="TabCtl (strict)"("Visible"=w1582) -> ()  [unwired: 2 in, 2 out]
                n1137 = property on="X Lo Val" class="DigNum (strict)"("Visible"=w1582) -> ()  [unwired: 2 in, 2 out]
                n1138 = property on="Low x Unit" class="Ring (strict)"("Visible"=w1582) -> ()  [unwired: 2 in, 2 out]
                n1139 = property on="LoTable_1" class="Tbl (strict)"("Visible"=w1582) -> ()  [unwired: 2 in, 2 out]
                n1140 = Unbundle By Name(w1591) -> ("Lower Limit"=w1587:cluster{dbl, dbl}[])
                n1141 = Equal To 0?(x=w1579) -> (x = 0?=w1578:bool)
                n1142 = local read "data unit"() -> (w1584:string)
                n1143 = case shown="2" w1590 {
                  tunnel: w1578 -> [_ w1595]
                  frame 1, Default {
                    n1144 = property on="Single Limit" class="Slide (strict)"("Disabled"=u8 0) -> ()  [unwired: 2 in, 2 out]
                  }
                  frame 2 {
                    n1145 = Select(t=u8 0, s=w1595, f=u8 1 ("Disabled")) -> (s? t:f=w1593:u8)
                    n1146 = property on="Multi Limit" class="Slide (strict)"("Disabled"=w1593) -> ()  [unwired: 2 in, 2 out]
                  }
                }
                n1147 = Index Array(array=w1587, index=0) -> (element=w1588:cluster{dbl, dbl})
                n1148 = local write "lo single unit"(w1584) -> ()
                n1149 = Build Array(w1584, "%") -> (w1585:string[])
                n1150 = Unbundle(w1588) -> (w1573:dbl)  [unwired: 1 out]
                n1151 = property on="Low y Unit" class="Ring (strict)"("Strings []"=w1585) -> ()  [unwired: 2 in, 2 out]
                n1152 = local write "RawLo Limit"(w1573) -> ()
                n1153 = call "CRYRepresent numeric by precission.vi"("Pprecision"=w1576, "Numeric In"=w1573) -> ("Out Format"=w1574:string, "Numeric Out"=w1575:dbl)  [unwired: 7 in, 1 out]
                n1154 = property on="Lo Limit Val" class="DigNum (strict)"("Value"=w1575, "FormatString"=w1574) -> ()  [unwired: 2 in, 2 out]
                n1155 = local write "Plot Multilimit"(TRUE ("Plot Multilimit")) -> ()
              }
              frame 1 {
                w1607 = TRUE ("Visible")
                w1608 = FALSE ("Visible")
                n1156 = case shown="1, Default" w1609 {
                  frame 1, Default {
                    n1157 = property on="Single Limit" class="Slide (strict)"("Disabled"=u8 1) -> ()  [unwired: 2 in, 2 out]
                  }
                  frame 2 {
                    n1158 = property on="Multi Limit" class="Slide (strict)"("Disabled"=u8 1) -> ()  [unwired: 2 in, 2 out]
                  }
                }
                n1159 = property on="LoTable_2" class="Tbl (strict)"("Visible"=w1608) -> ()  [unwired: 2 in, 2 out]
                n1160 = property on="Sub5 Tab" class="TabCtl (strict)"("Visible"=w1608) -> ()  [unwired: 2 in, 2 out]
                n1161 = property on="Sub3 Tab" class="TabCtl (strict)"("Visible"=w1608) -> ()  [unwired: 2 in, 2 out]
                n1162 = property on="Lo_type" class="RadioBtnsControl (strict)"("Visible"=TRUE) -> ("Controls[]"=w1605:refnum<vi>[])  [unwired: 2 in, 2 out]
                n1163 = property on="Sub7 Tab" class="TabCtl (strict)"("Visible"=w1607) -> ()  [unwired: 2 in, 2 out]
                n1164 = property on="LoSingleVal" class="DigNum (strict)"("Visible"=w1607) -> ()  [unwired: 2 in, 2 out]
                n1165 = for {
                  tunnel: w1605 -> [w1614] mode=indexing
                  i -> [w1615]
                  n1166 = case shown="0, Default" w1615 {
                    tunnel: w1614 -> [w1616 w1620]
                    frame 0, Default {
                      n1167 = To More Specific Class(target class=refnum<vi> refnum ("Single Values"), reference=w1616) -> (specific class reference=w1619:refnum<vi>)  [unwired: 1 in, 1 out]
                      n1168 = property class="Bool (strict)"(reference=w1619, "Disabled"=u8 0) -> ()  [unwired: 1 in, 2 out]
                    }
                    frame 1, 2 {
                      n1169 = To More Specific Class(target class=refnum<vi> refnum ("Single Values"), reference=w1620) -> (specific class reference=w1623:refnum<vi>)  [unwired: 1 in, 1 out]
                      n1170 = property class="Bool (strict)"(reference=w1623, "Disabled"=u8 2) -> ()  [unwired: 1 in, 2 out]
                    }
                  }
                }
                n1171 = property on="Lo_xyz" class="Slide (strict)"("Visible"=TRUE, "TextLbls[]"=string[] ["x", "y", "z"] ("Text Labels[]"), "Disabled"=u8 0) -> ()  [unwired: 2 in, 2 out]
                n1172 = local read "Load state"() -> (w1600:bool)
                n1173 = Not Equal?(x=w1597, y=w1598) -> (x != y?=w1601:bool)
                n1174 = Or(x=w1601, y=w1600) -> (x .or. y?=w1599:bool)
                n1175 = case shown="True" w1599 {
                  frame False {
                    n1176 = local write "Plot Multilimit"(TRUE ("Plot Multilimit")) -> ()
                  }
                  frame True {
                    n1177 = property on="Lo_type" class="RadioBtnsControl (strict)"("Val(Sgnl)"=enum32{"Single Values", "Curves", "Waveforms"}."Single Values" ("Up_type")) -> ()  [unwired: 2 in, 2 out]
                  }
                }
              }
            }
          }
          frame 1 {
            w1624 = FALSE ("Visible")
            w1625 = FALSE ("Visible")
            n1178 = case shown="0, Default" w1630 {
              selector: w1630 -> [w1631 w1663]
              tunnel: w1629 -> [w1636 _]
              tunnel: w1628 -> [w1638 _]
              tunnel: w1627 -> [w1637 _]
              tunnel: w1626 -> [w1632 w1662]
              frame 0, Default {
                w1642 = FALSE ("Visible")
                w1639 = u8 0 ("Disabled")
                w1640 = TRUE ("Visible")
                n1179 = property on="Delete Lower" class="Bool"("Disabled"=w1639) -> ()  [unwired: 2 in, 2 out]
                n1180 = property on="Lo Limit Val" class="DigNum (strict)"("Visible"=w1642) -> ()  [unwired: 2 in, 2 out]
                n1181 = property on="Sub5 Tab" class="TabCtl (strict)"("Visible"=w1640) -> ()  [unwired: 2 in, 2 out]
                n1182 = property on="X Lo Val" class="DigNum (strict)"("Visible"=w1640) -> ()  [unwired: 2 in, 2 out]
                n1183 = property on="Insert Lower" class="Bool"("Disabled"=w1639) -> ()  [unwired: 2 in, 2 out]
                n1184 = property on="lo single unit" class="Str"("Visible"=w1642) -> (error out=w1641:errorcluster)  [unwired: 2 in, 1 out]
                n1185 = property on="Low x Unit" class="Ring (strict)"("Visible"=w1640) -> ()  [unwired: 2 in, 2 out]
                n1186 = property on="copy Lower" class="Bool"("Disabled"=w1639) -> ()  [unwired: 2 in, 2 out]
                n1187 = local read "Load state"() -> (w1634:bool)
                n1188 = property on="Sub3 Tab" class="TabCtl (strict)"("Visible"=w1640) -> ()  [unwired: 2 in, 2 out]
                n1189 = Not Equal?(x=w1632, y=w1631) -> (x != y?=w1635:bool)
                n1190 = property on="Sub7 Tab" class="TabCtl (strict)"(error in=w1641, "Visible"=w1642) -> ()  [unwired: 1 in, 2 out]
                n1191 = property on="LoTable_1" class="Tbl (strict)"("Visible"=w1640) -> ()  [unwired: 2 in, 2 out]
                n1192 = Or(x=w1635, y=w1634) -> (x .or. y?=w1633:bool)
                n1193 = case shown="True" w1633 {
                  tunnel: w1638 -> [_ w1645]
                  tunnel: w1637 -> [_ w1644]
                  tunnel: w1636 -> [_ w1643]
                  frame False {
                  }
                  frame True {
                    w1647 = "%"
                    n1194 = property on="Data Table" class="Tbl (strict)"() -> ("Row Headers[]"=w1651:string[])  [unwired: 2 in, 2 out]
                    n1195 = flat-sequence {
                      tunnel: w1645 -> [w1657]
                      tunnel: w1644 -> [w1656]
                      tunnel: w1643 -> [w1655]
                      frame #0 {
                        n1196 = property on="LoTable_1" class="Tbl (strict)"("Value"=string[][] [] ("LoTable_1")) -> ()  [unwired: 2 in, 2 out]
                      }
                      frame #1 {
                        n1197 = Unbundle By Name(w1655) -> ("Lower Limit"=w1658:cluster{dbl, dbl}[])
                        n1198 = call "CRYCurve to Table.vi"("y precision"=w1656, "x precision"=w1657, "Limit curve In"=w1658) -> ("Limit Table"=w1659:string[][])  [unwired: 1 in, 7 out]
                        n1199 = local write "LoTable_1"(w1659) -> ()
                      }
                      frame #2 {
                        n1200 = local write "Load state"(FALSE ("Load state")) -> ()
                        n1201 = local write "Plot graphs"(TRUE ("Plot graphs")) -> ()
                      }
                    }
                    n1202 = Index Array(array=w1651, index=0) -> (element=w1650:string)
                    n1203 = Index Array(array=w1651, index=1) -> (element=w1648:string)
                    n1204 = property on="LoTable_1" class="Tbl (strict)"("Row Headers[]"=w1651) -> ()  [unwired: 2 in, 2 out]
                    n1205 = Build Array(w1650, w1647) -> (w1649:string[])
                    n1206 = Build Array(w1648, w1647) -> (w1646:string[])
                    n1207 = property on="Low y Unit" class="Ring (strict)"("Strings []"=w1646) -> ()  [unwired: 2 in, 2 out]
                    n1208 = property on="Low x Unit" class="Ring (strict)"("Strings []"=w1649) -> ()  [unwired: 2 in, 2 out]
                  }
                }
              }
              frame 1 {
                w1673 = TRUE ("Visible")
                w1672 = FALSE ("Visible")
                n1209 = property on="Sub3 Tab" class="TabCtl (strict)"("Visible"=w1672) -> ()  [unwired: 2 in, 2 out]
                n1210 = property on="LoSingleVal" class="DigNum (strict)"("Visible"=w1672) -> ()  [unwired: 2 in, 2 out]
                n1211 = property on="Lo_type" class="RadioBtnsControl (strict)"("Visible"=TRUE) -> ("Controls[]"=w1670:refnum<vi>[])  [unwired: 2 in, 2 out]
                n1212 = property on="Sub5 Tab" class="TabCtl (strict)"("Visible"=w1672) -> ()  [unwired: 2 in, 2 out]
                n1213 = for {
                  tunnel: w1670 -> [w1676] mode=indexing
                  i -> [w1677]
                  n1214 = case shown="2" w1677 {
                    tunnel: w1676 -> [w1678 w1682]
                    frame 0, 1, Default {
                      n1215 = To More Specific Class(target class=refnum<vi> refnum ("Single Values"), reference=w1678) -> (specific class reference=w1681:refnum<vi>)  [unwired: 1 in, 1 out]
                      n1216 = property class="Bool (strict)"(reference=w1681, "Disabled"=u8 0) -> ()  [unwired: 1 in, 2 out]
                    }
                    frame 2 {
                      n1217 = To More Specific Class(target class=refnum<vi> refnum ("Single Values"), reference=w1682) -> (specific class reference=w1685:refnum<vi>)  [unwired: 1 in, 1 out]
                      n1218 = property class="Bool (strict)"(reference=w1685, "Disabled"=u8 2) -> ()  [unwired: 1 in, 2 out]
                    }
                  }
                }
                n1219 = property on="LoTable_2" class="Tbl (strict)"("Visible"=w1673) -> ()  [unwired: 2 in, 2 out]
                n1220 = property on="Sub7 Tab" class="TabCtl (strict)"("Visible"=w1673) -> ()  [unwired: 2 in, 2 out]
                n1221 = local read "Load state"() -> (w1665:bool)
                n1222 = Not Equal?(x=w1662, y=w1663) -> (x != y?=w1666:bool)
                n1223 = property on="Lo_xyz" class="Slide (strict)"("Visible"=TRUE, "TextLbls[]"=string[] ["x", "y", "z"] ("Text Labels[]"), "Disabled"=u8 0) -> ()  [unwired: 2 in, 2 out]
                n1224 = Or(x=w1666, y=w1665) -> (x .or. y?=w1664:bool)
                n1225 = case shown="False" w1664 {
                  frame False {
                    n1226 = local write "Plot graphs"(TRUE ("Plot graphs")) -> ()
                  }
                  frame True {
                    n1227 = local read "Lo_type"() -> (w1675:enum32{"Single Values", "Curves", "Waveforms"})
                    n1228 = property on="Lo_type" class="RadioBtnsControl (strict)"("Val(Sgnl)"=w1675) -> ()  [unwired: 2 in, 2 out]
                  }
                }
              }
            }
            n1229 = property on="UpAlignRst_2" class="Str"("Visible"=w1624) -> ()  [unwired: 2 in, 2 out]
            n1230 = property on="LowAlignRst_2" class="Str"("Visible"=w1624) -> ()  [unwired: 2 in, 2 out]
            n1231 = property on="UpAlignRst_1" class="Str"("Visible"=w1625) -> ()  [unwired: 2 in, 2 out]
            n1232 = property on="DataAlignRst" class="Str"("Visible"=w1625) -> ()  [unwired: 2 in, 2 out]
            n1233 = property on="LowAlignRst_1" class="Str"("Visible"=w1625) -> ()  [unwired: 2 in, 2 out]
          }
          frame 2 {
            w1686 = FALSE ("Visible")
            w1687 = FALSE ("Visible")
            n1234 = case shown="0, Default" w1692 {
              selector: w1692 -> [w1697 w1727]
              tunnel: w1691 -> [w1695 _]
              tunnel: w1690 -> [w1694 _]
              tunnel: w1689 -> [w1693 _]
              tunnel: w1688 -> [w1698 w1726]
              frame 0, Default {
                w1706 = FALSE ("Visible")
                w1702 = u8 0 ("Disabled")
                w1704 = TRUE ("Visible")
                n1235 = property on="Lo Limit Val" class="DigNum (strict)"("Visible"=w1706) -> ()  [unwired: 2 in, 2 out]
                n1236 = property on="Delete Lower" class="Bool"("Disabled"=w1702) -> ()  [unwired: 2 in, 2 out]
                n1237 = property on="Insert Lower" class="Bool"("Disabled"=w1702) -> ()  [unwired: 2 in, 2 out]
                n1238 = property on="copy Lower" class="Bool"("Disabled"=u8 2) -> ()  [unwired: 2 in, 2 out]
                n1239 = property on="Sub5 Tab" class="TabCtl (strict)"("Visible"=w1704) -> ()  [unwired: 2 in, 2 out]
                n1240 = property on="Low x Unit" class="Ring (strict)"("Visible"=w1704) -> (error out=w1703:errorcluster)  [unwired: 2 in, 1 out]
                n1241 = local read "Load state"() -> (w1699:bool)
                n1242 = property on="lo single unit" class="Str"("Visible"=w1706) -> (error out=w1705:errorcluster)  [unwired: 2 in, 1 out]
                n1243 = property on="X Lo Val" class="DigNum (strict)"("Visible"=w1704) -> ()  [unwired: 2 in, 2 out]
                n1244 = property on="Sub3 Tab" class="TabCtl (strict)"(error in=w1703, "Visible"=w1704) -> ()  [unwired: 1 in, 2 out]
                n1245 = Not Equal?(x=w1698, y=w1697) -> (x != y?=w1700:bool)
                n1246 = property on="Sub7 Tab" class="TabCtl (strict)"(error in=w1705, "Visible"=w1706) -> ()  [unwired: 1 in, 2 out]
                n1247 = property on="LoTable_1" class="Tbl (strict)"("Visible"=w1704) -> ()  [unwired: 2 in, 2 out]
                n1248 = Or(x=w1700, y=w1699) -> (x .or. y?=w1696:bool)
                n1249 = case shown="True" w1696 {
                  tunnel: w1694 -> [_ w1709]
                  tunnel: w1693 -> [_ w1708]
                  tunnel: w1695 -> [_ w1707]
                  frame False {
                  }
                  frame True {
                    w1711 = "%"
                    n1250 = property on="Data Table" class="Tbl (strict)"() -> ("Row Headers[]"=w1715:string[])  [unwired: 2 in, 2 out]
                    n1251 = flat-sequence {
                      tunnel: w1709 -> [w1721]
                      tunnel: w1708 -> [w1720]
                      tunnel: w1707 -> [w1719]
                      frame #0 {
                        n1252 = property on="LoTable_1" class="Tbl (strict)"("Value"=string[][] [] ("LoTable_1")) -> ()  [unwired: 2 in, 2 out]
                      }
                      frame #1 {
                        n1253 = Unbundle By Name(w1719) -> ("Lower Limit"=w1722:cluster{dbl, dbl}[])
                        n1254 = call "CRYCurve to Table.vi"("y precision"=w1720, "x precision"=w1721, "Limit curve In"=w1722) -> ("Limit Table"=w1723:string[][])  [unwired: 1 in, 7 out]
                        n1255 = local write "LoTable_1"(w1723) -> ()
                      }
                      frame #2 {
                        n1256 = local write "Plot graphs"(TRUE ("Plot graphs")) -> ()
                        n1257 = local write "Load state"(FALSE ("Load state")) -> ()
                      }
                    }
                    n1258 = Index Array(array=w1715, index=0) -> (element=w1714:string)
                    n1259 = Index Array(array=w1715, index=1) -> (element=w1712:string)
                    n1260 = property on="LoTable_1" class="Tbl (strict)"("Row Headers[]"=w1715) -> ()  [unwired: 2 in, 2 out]
                    n1261 = Build Array(w1714, w1711) -> (w1713:string[])
                    n1262 = Build Array(w1712, w1711) -> (w1710:string[])
                    n1263 = property on="Low y Unit" class="Ring (strict)"("Strings []"=w1710) -> ()  [unwired: 2 in, 2 out]
                    n1264 = property on="Low x Unit" class="Ring (strict)"("Strings []"=w1713) -> ()  [unwired: 2 in, 2 out]
                  }
                }
              }
              frame 1 {
                w1735 = TRUE ("Visible")
                w1733 = FALSE ("Visible")
                n1265 = property on="Lo_type" class="RadioBtnsControl (strict)"("Visible"=TRUE) -> ("Controls[]"=w1731:refnum<vi>[])  [unwired: 2 in, 2 out]
                n1266 = property on="Sub5 Tab" class="TabCtl (strict)"("Visible"=w1733) -> ()  [unwired: 2 in, 2 out]
                n1267 = property on="Sub7 Tab" class="TabCtl (strict)"("Visible"=w1735) -> (error out=w1734:errorcluster)  [unwired: 2 in, 1 out]
                n1268 = for {
                  tunnel: w1731 -> [w1738] mode=indexing
                  i -> [w1739]
                  n1269 = case shown="1" w1739 {
                    tunnel: w1738 -> [w1740 w1744]
                    frame 0, 2, Default {
                      n1270 = To More Specific Class(target class=refnum<vi> refnum ("Single Values"), reference=w1740) -> (specific class reference=w1743:refnum<vi>)  [unwired: 1 in, 1 out]
                      n1271 = property class="Bool (strict)"(reference=w1743, "Disabled"=u8 0) -> ()  [unwired: 1 in, 2 out]
                    }
                    frame 1 {
                      n1272 = To More Specific Class(target class=refnum<vi> refnum ("Single Values"), reference=w1744) -> (specific class reference=w1747:refnum<vi>)  [unwired: 1 in, 1 out]
                      n1273 = property class="Bool (strict)"(reference=w1747, "Disabled"=u8 2) -> ()  [unwired: 1 in, 2 out]
                    }
                  }
                }
                n1274 = property on="Sub3 Tab" class="TabCtl (strict)"("Visible"=w1733) -> ()  [unwired: 2 in, 2 out]
                n1275 = property on="LoTable_2" class="Tbl (strict)"(error in=w1734, "Visible"=w1735) -> ()  [unwired: 1 in, 2 out]
                n1276 = property on="LoSingleVal" class="DigNum (strict)"("Visible"=w1733) -> ()  [unwired: 2 in, 2 out]
                n1277 = local read "Load state"() -> (w1729:bool)
                n1278 = Not Equal?(x=w1726, y=w1727) -> (x != y?=w1728:bool)
                n1279 = Or(x=w1728, y=w1729) -> (x .or. y?=w1730:bool)
                n1280 = case shown="False" w1730 {
                  frame False {
                    n1281 = local write "Plot graphs"(TRUE ("Plot graphs")) -> ()
                  }
                  frame True {
                    n1282 = local read "Lo_type"() -> (w1737:enum32{"Single Values", "Curves", "Waveforms"})
                    n1283 = property on="Lo_type" class="RadioBtnsControl (strict)"("Val(Sgnl)"=w1737) -> ()  [unwired: 2 in, 2 out]
                  }
                }
              }
            }
            n1284 = property on="UpAlignRst_1" class="Str"("Visible"=w1687) -> ()  [unwired: 2 in, 2 out]
            n1285 = property on="DataAlignRst" class="Str"("Visible"=w1687) -> ()  [unwired: 2 in, 2 out]
            n1286 = property on="LowAlignRst_1" class="Str"("Visible"=w1687) -> ()  [unwired: 2 in, 2 out]
            n1287 = property on="UpAlignRst_2" class="Str"("Visible"=w1686) -> ()  [unwired: 2 in, 2 out]
            n1288 = property on="LowAlignRst_2" class="Str"("Visible"=w1686) -> ()  [unwired: 2 in, 2 out]
          }
          frame 3 {
            n1289 = case shown="0, Default" w1752 {
              selector: w1752 -> [_ w1778]
              tunnel: w1751 -> [w1758 w1789]
              tunnel: w1750 -> [w1761 _]
              tunnel: w1749 -> [w1756 _]
              tunnel: w1748 -> [_ w1777]
              frame 0, Default {
                w1763 = u8 2 ("Disabled")
                w1765 = FALSE ("Visible")
                w1764 = TRUE ("Visible")
                w1768 = "dB" ("lo single unit")
                n1290 = property on="Delete Lower" class="Bool"("Disabled"=w1763) -> ()  [unwired: 2 in, 2 out]
                n1291 = property on="Insert Lower" class="Bool"("Disabled"=w1763) -> ()  [unwired: 2 in, 2 out]
                n1292 = property on="Lo Limit Val" class="DigNum (strict)"("Visible"=w1764) -> ()  [unwired: 2 in, 2 out]
                n1293 = property on="lo single unit" class="Str"("Visible"=w1764) -> ()  [unwired: 2 in, 2 out]
                n1294 = property on="Sub3 Tab" class="TabCtl (strict)"("Visible"=w1764) -> ()  [unwired: 2 in, 2 out]
                n1295 = property on="Sub5 Tab" class="TabCtl (strict)"("Visible"=w1764) -> ()  [unwired: 2 in, 2 out]
                n1296 = property on="copy Lower" class="Bool"("Disabled"=u8 0) -> ()  [unwired: 2 in, 2 out]
                n1297 = property on="X Lo Val" class="DigNum (strict)"("Visible"=w1765) -> ()  [unwired: 2 in, 2 out]
                n1298 = property on="Low x Unit" class="Ring (strict)"("Visible"=w1765) -> ()  [unwired: 2 in, 2 out]
                n1299 = property on="Sub7 Tab" class="TabCtl (strict)"("Visible"=w1765) -> ()  [unwired: 2 in, 2 out]
                n1300 = property on="LoTable_1" class="Tbl (strict)"("Visible"=w1765) -> ()  [unwired: 2 in, 2 out]
                n1301 = local read "UpSource"() -> (w1760:u16)
                n1302 = Unbundle By Name(w1761) -> ("Lower Limit"=w1769:cluster{dbl, dbl}[])
                n1303 = Equal To 0?(x=w1760) -> (x = 0?=w1759:bool)
                n1304 = local write "lo single unit"(w1768) -> ()
                n1305 = Build Array(w1768, "%") -> (w1766:string[])
                n1306 = case shown="1, Default" w1758 {
                  tunnel: w1759 -> [_ w1775]
                  frame 1, Default {
                    n1307 = property on="Single Limit" class="Slide (strict)"("Disabled"=u8 0) -> ()  [unwired: 2 in, 2 out]
                  }
                  frame 2 {
                    n1308 = Select(t=u8 0, s=w1775, f=u8 1 ("Disabled")) -> (s? t:f=w1773:u8)
                    n1309 = property on="Multi Limit" class="Slide (strict)"("Disabled"=w1773) -> ()  [unwired: 2 in, 2 out]
                  }
                }
                n1310 = property on="Low y Unit" class="Ring (strict)"("Strings []"=w1766) -> ()  [unwired: 2 in, 2 out]
                n1311 = local write "Multi unit"(w1768) -> ()
                n1312 = Index Array(array=w1769, index=0) -> (element=w1770:cluster{dbl, dbl})
                n1313 = Unbundle(w1770) -> (w1753:dbl)  [unwired: 1 out]
                n1314 = local write "RawLo Limit"(w1753) -> ()
                n1315 = call "CRYRepresent numeric by precission.vi"("Pprecision"=w1756, "Numeric In"=w1753) -> ("Out Format"=w1754:string, "Numeric Out"=w1755:dbl)  [unwired: 7 in, 1 out]
                n1316 = property on="Lo Limit Val" class="DigNum (strict)"("Value"=w1755, "FormatString"=w1754) -> ()  [unwired: 2 in, 2 out]
                n1317 = local write "Plot Multilimit"(TRUE ("Plot Multilimit")) -> ()
              }
              frame 1 {
                w1788 = TRUE ("Visible")
                w1787 = FALSE ("Visible")
                n1318 = case shown="2" w1789 {
                  frame 1, Default {
                    n1319 = property on="Single Limit" class="Slide (strict)"("Disabled"=u8 1) -> ()  [unwired: 2 in, 2 out]
                  }
                  frame 2 {
                    n1320 = property on="Multi Limit" class="Slide (strict)"("Disabled"=u8 1) -> ()  [unwired: 2 in, 2 out]
                  }
                }
                n1321 = property on="Sub3 Tab" class="TabCtl (strict)"("Visible"=w1787) -> ()  [unwired: 2 in, 2 out]
                n1322 = property on="Sub5 Tab" class="TabCtl (strict)"("Visible"=w1787) -> ()  [unwired: 2 in, 2 out]
                n1323 = property on="LoTable_2" class="Tbl (strict)"("Visible"=w1787) -> ()  [unwired: 2 in, 2 out]
                n1324 = property on="Lo_type" class="RadioBtnsControl (strict)"("Visible"=TRUE) -> ("Controls[]"=w1785:refnum<vi>[])  [unwired: 2 in, 2 out]
                n1325 = for {
                  tunnel: w1785 -> [w1794] mode=indexing
                  i -> [w1795]
                  n1326 = case shown="1, 2" w1795 {
                    tunnel: w1794 -> [w1796 w1800]
                    frame 0, Default {
                      n1327 = To More Specific Class(target class=refnum<vi> refnum ("Single Values"), reference=w1796) -> (specific class reference=w1799:refnum<vi>)  [unwired: 1 in, 1 out]
                      n1328 = property class="Bool (strict)"(reference=w1799, "Disabled"=u8 0) -> ()  [unwired: 1 in, 2 out]
                    }
                    frame 1, 2 {
                      n1329 = To More Specific Class(target class=refnum<vi> refnum ("Single Values"), reference=w1800) -> (specific class reference=w1803:refnum<vi>)  [unwired: 1 in, 1 out]
                      n1330 = property class="Bool (strict)"(reference=w1803, "Disabled"=u8 2) -> ()  [unwired: 1 in, 2 out]
                    }
                  }
                }
                n1331 = property on="Sub7 Tab" class="TabCtl (strict)"("Visible"=w1788) -> ()  [unwired: 2 in, 2 out]
                n1332 = property on="LoSingleVal" class="DigNum (strict)"("Visible"=w1788) -> ()  [unwired: 2 in, 2 out]
                n1333 = property on="Lo_xyz" class="Slide (strict)"("Visible"=TRUE, "Disabled"=u8 0, "TextLbls[]"=string[] ["x", "y", "z"] ("Text Labels[]")) -> ()  [unwired: 2 in, 2 out]
                n1334 = local read "Load state"() -> (w1780:bool)
                n1335 = Not Equal?(x=w1777, y=w1778) -> (x != y?=w1781:bool)
                n1336 = Or(x=w1781, y=w1780) -> (x .or. y?=w1779:bool)
                n1337 = case shown="True" w1779 {
                  frame False {
                    n1338 = local write "Plot Multilimit"(TRUE ("Plot Multilimit")) -> ()
                  }
                  frame True {
                    n1339 = property on="Lo_type" class="RadioBtnsControl (strict)"("Val(Sgnl)"=enum32{"Single Values", "Curves", "Waveforms"}."Single Values" ("Up_type")) -> ()  [unwired: 2 in, 2 out]
                  }
                }
              }
            }
          }
        }
      }
      event "Lo_type": Value Change {
        n1340 = event-data() -> ("NewVal"=w1805:enum32{"Single Values", "Curves", "Waveforms"})  [unwired: 6 out]
        n1341 = case shown="\"Curves\"" w1805 {
          tunnel: w1804 -> [w1817 w1828 w1840]
          tunnel: [w1818 w1830 w1841] -> w1808
          frame "Single Values", Default {
            n1342 = call "CRYGet Upper Step Data.vi"("Type In"=enum16{"Curves", "Values", "Results", "WFM"}."Values", "No.VI"=w1817) -> ("Value array"=w1815:T13)  [unwired: 9 out]
            n1343 = property on="Lo_xyz" class="Slide (strict)"("Visible"=TRUE, "TextLbls[]"=string[] ["x", "y", "z"] ("Text Labels[]"), "Disabled"=u8 0, "Scale.Text Color"=u32 0) -> ()  [unwired: 2 in, 2 out]
            n1344 = for {
              tunnel: w1815 -> [w1825] mode=indexing
              tunnel: [w1824] -> w1818 mode=indexing
              n1345 = Unbundle By Name(w1825) -> ("Name"=w1824:string)
            }
            n1346 = property on="LoTable_2" class="Tbl (strict)"("Disabled"=u8 0) -> ()  [unwired: 2 in, 2 out]
          }
          frame "Curves" {
            n1347 = call "CRYGet Upper Step Data.vi"("Type In"=enum16{"Curves", "Values", "Results", "WFM"}."Curves", "No.VI"=w1828) -> ("Curve array"=w1826:T13)  [unwired: 9 out]
            n1348 = property on="Lo_xyz" class="Slide (strict)"("Visible"=TRUE, "TextLbls[]"=string[] ["x", "y", "z"] ("Text Labels[]"), "Disabled"=u8 0, "Scale.Text Color"=u32 0) -> ()  [unwired: 2 in, 2 out]
            n1349 = for {
              tunnel: w1826 -> [w1837] mode=indexing
              tunnel: [w1836] -> w1830 mode=indexing
              n1350 = Unbundle By Name(w1837) -> ("Name"=w1836:string)
            }
            n1351 = property on="LoTable_2" class="Tbl (strict)"("Disabled"=u8 0) -> ()  [unwired: 2 in, 2 out]
            n1352 = property on="LoTable_2" class="Tbl (strict)"("Value"=string[][] [] ("Lower limit Table")) -> ()  [unwired: 2 in, 2 out]
          }
          frame "Waveforms" {
            w1846 = u8 2 ("Disabled")
            n1353 = call "CRYGet Upper Step Data.vi"("Type In"=enum16{"Curves", "Values", "Results", "WFM"}."WFM", "No.VI"=w1840) -> ("Waveform Array"=w1838:T14)  [unwired: 9 out]
            n1354 = property on="Lo_xyz" class="Slide (strict)"("Visible"=TRUE, "TextLbls[]"=string[] ["x0", "dx", "y"] ("Text Labels[]"), "Disabled"=w1846, "Value"=w1846, "Scale.Text Color"=u32 1193471) -> ()  [unwired: 2 in, 2 out]
            n1355 = for {
              tunnel: w1838 -> [w1849] mode=indexing
              tunnel: [w1848] -> w1841 mode=indexing
              n1356 = Unbundle By Name(w1849) -> ("Name"=w1848:string)
            }
            n1357 = property on="LoTable_2" class="Tbl (strict)"("Value"=string[][] [] ("Lower limit Table"), "Disabled"=u8 2) -> ()  [unwired: 2 in, 2 out]
          }
        }
        n1358 = local read "Limit Cluster"() -> (w1814:T1)
        n1359 = property on="Lo Cur Name" class="Ring (strict)"("Strings []"=w1808) -> ()  [unwired: 2 in, 2 out]
        n1360 = Unbundle By Name(w1814) -> ("Curve Names"=w1813:string[])
        n1361 = Index Array(array=w1813, index=1) -> (element=w1807:string)
        n1362 = Search 1D Array(1D array=w1808, element=w1807) -> (index of element=w1809:i32)  [unwired: 1 in]
        n1363 = Less Than 0?(x=w1809) -> (x < 0?=w1811:bool)
        n1364 = Select(t=0, s=w1811, f=w1809) -> (s? t:f=w1806:i32)
        n1365 = property on="Lo Cur Name" class="Ring (strict)"("Val(Sgnl)"=w1806) -> ()  [unwired: 2 in, 2 out]
      }
      event "Lo Cur Name": Value Change {
        w1851 = FALSE ("Visible")
        w1852 = FALSE ("Visible")
        n1366 = event-data() -> ("NewVal"=w1853:u16)  [unwired: 6 out]
        n1367 = local read "Lo_type"() -> (w1855:enum32{"Single Values", "Curves", "Waveforms"})
        n1368 = Equal?(x=w1855, y=u16 2) -> (x = y?=w1863:bool)
        n1369 = property on="UpAlignRst_2" class="Str"("Visible"=w1851) -> ()  [unwired: 2 in, 2 out]
        n1370 = property on="LowAlignRst_2" class="Str"("Visible"=w1851) -> ()  [unwired: 2 in, 2 out]
        n1371 = property on="UpAlignRst_1" class="Str"("Visible"=w1852) -> ()  [unwired: 2 in, 2 out]
        n1372 = property on="DataAlignRst" class="Str"("Visible"=w1852) -> ()  [unwired: 2 in, 2 out]
        n1373 = property on="LowAlignRst_1" class="Str"("Visible"=w1852) -> ()  [unwired: 2 in, 2 out]
        n1374 = case shown="True" w1863 {
          tunnel: w1853 -> [w1876 w1892]
          tunnel: w1855 -> [w1874 _]
          tunnel: w1850 -> [w1875 w1889]
          tunnel: [w1877 w1894] -> w1856
          frame False {
            n1375 = case shown="\"Curves\"" w1874 {
              tunnel: w1875 -> [w1882 w1885]
              tunnel: [w1881 w1884] -> w1873
              frame "Single Values", Default {
                n1376 = call "CRYGet Upper Step Data.vi"("Type In"=enum16{"Curves", "Values", "Results", "WFM"}."Values" ("Type"), "No.VI"=w1882) -> ("Value array"=w1881:T13)  [unwired: 9 out]
              }
              frame "Curves" {
                n1377 = call "CRYGet Upper Step Data.vi"("Type In"=enum16{"Curves", "Values", "Results", "WFM"}."Curves" ("Type"), "No.VI"=w1885) -> ("Curve array"=w1884:T13)  [unwired: 9 out]
              }
            }
            n1378 = Index Array(array=w1873, index=w1876) -> (element=→"Lo Curve and Values":T3)
            n1379 = local read "Lo_xyz"() -> (w1880:u16)
            n1380 = property on="Lo Cur Name" class="Ring (strict)"() -> ("Strings []"=w1879:string[])  [unwired: 2 in, 2 out]
            n1381 = property on="Lo_xyz" class="Slide (strict)"("Val(Sgnl)"=w1880) -> ()  [unwired: 2 in, 2 out]
            n1382 = Index Array(array=w1879, index=w1876) -> (element=w1877:string)
          }
          frame True {
            n1383 = call "CRYGet Upper Step Data.vi"("Type In"=enum16{"Curves", "Values", "Results", "WFM"}."WFM", "No.VI"=w1889) -> ("Waveform Array"=w1887:T14)  [unwired: 9 out]
            n1384 = Index Array(array=w1887, index=w1892) -> (element=w1895:T2)
            "Lo Wave" <- w1895
            n1385 = Unbundle By Name(w1895) -> ("X unit"=w1898:string, "Y unit"=w1897:string)
            n1386 = property on="Lo Cur Name" class="Ring (strict)"() -> ("Strings []"=w1893:string[])  [unwired: 2 in, 2 out]
            n1387 = Build Array(w1898, w1897) -> (w1896:string[])
            n1388 = local write "low_unit"(w1897) -> ()
            n1389 = Index Array(array=w1893, index=w1892) -> (element=w1894:string)
            n1390 = property on="LoTable_2" class="Tbl (strict)"("Row Headers[]"=w1896) -> ()  [unwired: 2 in, 2 out]
            n1391 = local write "Load state"(FALSE ("Load state")) -> ()
            n1392 = local write "Plot graphs"(TRUE ("Plot graphs")) -> ()
          }
        }
        n1393 = local read "Limit Cluster"() -> (w1857:T1)
        n1394 = Unbundle By Name(w1857) -> ("Curve Names"=w1859:string[])
        n1395 = Index Array(array=w1859, index=1) -> (element=w1861:string)
        n1396 = Empty String/Path?(string/path=w1861) -> (empty?=w1860:bool)
        n1397 = case shown="True" w1860 {
          tunnel: w1856 -> [w1866 w1870]
          tunnel: w1859 -> [w1868 w1871]
          tunnel: [w1865 w1869] -> w1858
          frame False {
            n1398 = Replace Array Subset(array=w1868, new element=w1866, index=1) -> (w1865:string[])
          }
          frame True {
            n1399 = Insert Into Array(array=w1871, index=1, new element=w1870) -> (w1869:string[])
          }
        }
        n1400 = Bundle By Name(cluster=w1857, "Data Selection Lower"=w1855, "Curve Names"=w1858) -> (w1854:T1)
        n1401 = local write "Limit Cluster"(w1854) -> ()
      }
      event "Lo_xyz": Value Change {
        n1402 = event-data() -> ("OldVal"=w1900:u16, "NewVal"=w1899:u16)  [unwired: 5 out]
        n1403 = Not Equal?(x=w1900, y=w1899) -> (x != y?=w1901:bool)
        n1404 = local read "Lo Curve and Values"() -> (w1903:T3)
        n1405 = case shown="True" w1901 {
          frame False {
          }
          frame True {
            w1910 = FALSE ("Visible")
            n1406 = property on="LowAlignRst_1" class="Str"("Visible"=w1910) -> ()  [unwired: 2 in, 2 out]
            n1407 = property on="LowAlignRst_2" class="Str"("Visible"=w1910) -> ()  [unwired: 2 in, 2 out]
          }
        }
        n1408 = local read "X Resolution"() -> (w1906:u8)
        n1409 = local read "Y Resolution"() -> (w1905:u8)
        n1410 = local read "Limits_Ring"() -> (w1907:u16)
        n1411 = local read "Lo_type"() -> (w1909:enum32{"Single Values", "Curves", "Waveforms"})
        n1412 = local read "Type"() -> (w1908:u16)
        n1413 = local read "Limit Cluster"() -> (w1904:T1)
        n1414 = Bundle By Name(cluster=w1904, "Lim Curve axis lo"=w1899) -> (w1902:T1)
        n1415 = case shown="1, Default" w1908 {
          selector: w1908 -> [w1918 _ _]
          tunnel: w1903 -> [w1919 w1950 w2026]
          tunnel: w1899 -> [w1917 w1949 w2025]
          tunnel: w1909 -> [_ w1948 w2024]
          tunnel: w1906 -> [_ w1944 w2023]
          tunnel: w1905 -> [w1914 w1943 w2022]
          tunnel: w1907 -> [_ _ _]
          frame 0, 3 {
            n1416 = Unbundle By Name(w1919) -> ("Y data"=w1920:u16, "X unit"=w1929:string, "Y unit"=w1930:string, "Curve"=w1928:cluster{"x":dbl, "y":dbl, "z":dbl}[])
            n1417 = Index Array(array=w1928, index=0) -> (element=w1926:cluster{"x":dbl, "y":dbl, "z":dbl})
            n1418 = Unbundle(w1926) -> ("x"=w1925:dbl, "y"=w1924:dbl, "z"=w1923:dbl)
            n1419 = case shown="1, Default" w1917 {
              tunnel: w1929 -> [_ w1938 _]
              tunnel: w1930 -> [w1932 _ _]
              tunnel: w1925 -> [_ w1937 _]
              tunnel: w1924 -> [w1934 _ _]
              tunnel: w1923 -> [_ _ w1939]
              tunnel: [w1934 w1937 w1939] -> w1913
              tunnel: [w1931 w1938 "deg." ("new element/subarray")] -> w1915
              tunnel: w1920 -> [w1933 _ _]
              frame 1, Default {
                n1420 = case shown="0, Default" w1933 {
                  tunnel: w1932 -> [_ w1936]
                  tunnel: ["dB" ("Y unit") w1936] -> w1931
                  frame 0, Default {
                  }
                  frame 1 {
                  }
                }
              }
              frame 0 {
              }
              frame 2 {
              }
            }
            n1421 = Equal To 0?(x=w1918) -> (x = 0?=w1922:bool)
            n1422 = property on="LoSingleVal" class="DigNum (strict)"("Value"=w1913, "Precision"=w1914) -> ()  [unwired: 2 in, 2 out]
            n1423 = local write "low_unit"(w1915) -> ()
            n1424 = Select(t=w1915, s=w1922, f="dB") -> (s? t:f=w1916:string)
            n1425 = local write "Multi unit"(w1916) -> ()
            n1426 = local write "Plot Multilimit"(TRUE ("Plot Multilimit")) -> ()
            n1427 = local write "Load state"(FALSE ("Load state")) -> ()
          }
          frame 1, Default {
            n1428 = case shown="\"Curves\", Default" w1948 {
              tunnel: w1949 -> [w1966 w1995]
              tunnel: w1950 -> [w1959 w1991]
              tunnel: [w1958 w1990] -> w1942
              tunnel: [w1957 w1989] -> w1941
              tunnel: [w1955 w1987] -> w1947
              frame "Single Values" {
                n1429 = Unbundle By Name(w1959) -> ("Y data"=w1956:u16, "X unit"=w1962:string, "Y unit"=w1961:string, "Curve"=w1969:cluster{"x":dbl, "y":dbl, "z":dbl}[])
                n1430 = Index Array(array=w1969, index=0) -> (element=w1967:cluster{"x":dbl, "y":dbl, "z":dbl})
                n1431 = Unbundle(w1967) -> ("x"=w1965:dbl, "y"=w1964:dbl, "z"=w1963:dbl)
                n1432 = case shown="0, Default" w1966 {
                  tunnel: w1965 -> [w1972 w1979 w1986]
                  tunnel: w1964 -> [_ w1978 _]
                  tunnel: w1963 -> [_ _ w1982]
                  tunnel: w1962 -> [w1971 w1976 w1984]
                  tunnel: w1961 -> [_ w1974 _]
                  tunnel: [w1971 w1976 w1984] -> w1955
                  tunnel: [w1971 w1973 "deg." ("new element/subarray")] -> w1958
                  tunnel: [w1970 w1977 w1985] -> w1960
                  tunnel: w1956 -> [_ w1975 _]
                  frame 0, Default {
                    n1433 = Bundle("x"=w1972, "x"=w1972) -> (w1970:cluster{"x":dbl, "x":dbl})  [unwired: 1 out]
                  }
                  frame 1 {
                    n1434 = Bundle("x"=w1979, "y"=w1978) -> (w1977:cluster{"x":dbl, "y":dbl})  [unwired: 1 out]
                    n1435 = case shown="0, Default" w1975 {
                      tunnel: w1974 -> [_ w1981]
                      tunnel: ["dB" ("Y unit") w1981] -> w1973
                      frame 0, Default {
                      }
                      frame 1 {
                      }
                    }
                  }
                  frame 2 {
                    n1436 = Bundle("x"=w1986, "z"=w1982) -> (w1985:cluster{"x":dbl, "z":dbl})  [unwired: 1 out]
                  }
                }
                n1437 = Build Array(w1960) -> (w1957:cluster{"x":dbl, "z":dbl}[])
              }
              frame "Curves", Default {
                n1438 = Unbundle By Name(w1991) -> ("Y data"=w1988:u16, "X unit"=w1994:string, "Y unit"=w1993:string, "Curve"=w1992:cluster{"x":dbl, "y":dbl, "z":dbl}[])
                n1439 = case shown="1, Default" w1995 {
                  tunnel: w1994 -> [w2000 w2008 w2016]
                  tunnel: w1993 -> [w1997 _ _]
                  tunnel: w1992 -> [w2001 w2010 w2017]
                  tunnel: [w2000 w2008 w2016] -> w1987
                  tunnel: [w1996 w2008 "deg." ("new element/subarray")] -> w1990
                  tunnel: [w1999 w2009 w2014] -> w1989
                  tunnel: w1988 -> [w1998 _ _]
                  frame 1, Default {
                    n1440 = for {
                      tunnel: w2001 -> [w2004] mode=indexing
                      tunnel: [w2006] -> w1999 mode=indexing
                      n1441 = Unbundle(w2004) -> ("x"=w2007:dbl, "y"=w2005:dbl)  [unwired: 1 out]
                      n1442 = Bundle("x"=w2007, "y"=w2005) -> (w2006:cluster{"x":dbl, "y":dbl})  [unwired: 1 out]
                    }
                    n1443 = case shown="0, Default" w1998 {
                      tunnel: w1997 -> [_ w2003]
                      tunnel: ["dB" ("Y unit") w2003] -> w1996
                      frame 0, Default {
                      }
                      frame 1 {
                      }
                    }
                  }
                  frame 0 {
                    n1444 = for {
                      tunnel: w2010 -> [w2011] mode=indexing
                      tunnel: [w2012] -> w2009 mode=indexing
                      n1445 = Unbundle(w2011) -> ("x"=w2013:dbl)  [unwired: 2 out]
                      n1446 = Bundle("x"=w2013, "x"=w2013) -> (w2012:cluster{"x":dbl, "x":dbl})  [unwired: 1 out]
                    }
                  }
                  frame 2 {
                    n1447 = for {
                      tunnel: w2017 -> [w2019] mode=indexing
                      tunnel: [w2020] -> w2014 mode=indexing
                      n1448 = Unbundle(w2019) -> ("x"=w2021:dbl, "z"=w2018:dbl)  [unwired: 1 out]
                      n1449 = Bundle("x"=w2021, "z"=w2018) -> (w2020:cluster{"x":dbl, "z":dbl})  [unwired: 1 out]
                    }
                  }
                }
              }
            }
            "Lo Limit Data" <- w1941
            n1450 = call "CRYCurve to Table.vi"("y precision"=w1943, "x precision"=w1944, "Limit curve In"=w1941) -> ("Limit Table"=w1945:string[][])  [unwired: 1 in, 7 out]
            n1451 = Build Array(w1947, w1942) -> (w1946:string[])
            n1452 = local write "low_unit"(w1942) -> ()
            n1453 = flat-sequence {
              tunnel: w1946 -> [w1952]
              tunnel: w1945 -> [w1951]
              frame #0 {
                n1454 = property on="LoTable_2" class="Tbl (strict)"("Value"=w1951, "Row Headers[]"=w1952) -> ()  [unwired: 2 in, 2 out]
              }
              frame #1 {
                n1455 = local write "Plot graphs"(TRUE ("Plot graphs")) -> ()
                n1456 = local write "Load state"(FALSE ("Load state")) -> ()
              }
            }
          }
          frame 2 {
            n1457 = case shown="\"Single Values\", Default" w2024 {
              tunnel: w2023 -> [w2034 _]
              tunnel: w2022 -> [w2036 _]
              tunnel: w2025 -> [w2035 _]
              tunnel: w2026 -> [w2033 _]
              frame "Single Values", Default {
                n1458 = Unbundle By Name(w2033) -> ("Y data"=w2031:u16, "X unit"=w2039:string, "Y unit"=w2038:string, "Curve"=w2045:cluster{"x":dbl, "y":dbl, "z":dbl}[])
                n1459 = Index Array(array=w2045, index=0) -> (element=w2043:cluster{"x":dbl, "y":dbl, "z":dbl})
                n1460 = Unbundle(w2043) -> ("x"=w2042:dbl, "y"=w2041:dbl, "z"=w2040:dbl)
                n1461 = case shown="1" w2035 {
                  tunnel: w2042 -> [w2052 w2059 w2066]
                  tunnel: w2041 -> [_ w2058 _]
                  tunnel: w2040 -> [_ _ w2062]
                  tunnel: w2039 -> [w2051 w2056 w2064]
                  tunnel: w2038 -> [_ w2054 _]
                  tunnel: [w2051 w2056 w2064] -> w2032
                  tunnel: [w2051 w2053 "deg." ("new element/subarray")] -> w2030
                  tunnel: [w2050 w2057 w2065] -> w2037
                  tunnel: w2031 -> [_ w2055 _]
                  frame 0, Default {
                    n1462 = Bundle("x"=w2052, "x"=w2052) -> (w2050:cluster{"x":dbl, "x":dbl})  [unwired: 1 out]
                  }
                  frame 1 {
                    n1463 = Bundle("x"=w2059, "y"=w2058) -> (w2057:cluster{"x":dbl, "y":dbl})  [unwired: 1 out]
                    n1464 = case shown="0, Default" w2055 {
                      tunnel: w2054 -> [_ w2061]
                      tunnel: ["dB" ("Y unit") w2061] -> w2053
                      frame 0, Default {
                      }
                      frame 1 {
                      }
                    }
                  }
                  frame 2 {
                    n1465 = Bundle("x"=w2066, "z"=w2062) -> (w2065:cluster{"x":dbl, "z":dbl})  [unwired: 1 out]
                  }
                }
                n1466 = Build Array(w2037) -> (w2027:cluster{"x":dbl, "z":dbl}[])
                n1467 = Build Array(w2032, w2030) -> (w2028:string[])
                n1468 = local write "low_unit"(w2030) -> ()
                n1469 = call "CRYCurve to Table.vi"("y precision"=w2036, "x precision"=w2034, "Limit curve In"=w2027) -> ("Limit Table"=w2029:string[][])  [unwired: 1 in, 7 out]
                n1470 = local write "Lo Limit Data"(w2027) -> ()
                n1471 = flat-sequence {
                  tunnel: w2029 -> [w2047]
                  tunnel: w2028 -> [w2046]
                  frame #0 {
                    n1472 = property on="LoTable_2" class="Tbl (strict)"("Value"=w2047, "Row Headers[]"=w2046) -> ()  [unwired: 2 in, 2 out]
                  }
                  frame #1 {
                    n1473 = local write "Plot graphs"(TRUE ("Plot graphs")) -> ()
                    n1474 = local write "Load state"(FALSE ("Load state")) -> ()
                  }
                }
              }
              frame "Waveforms" {
              }
            }
          }
        }
        n1475 = local write "Limit Cluster"(w1902) -> ()
      }
      event "Alignment": Value Change {
        n1476 = event-data() -> ("OldVal"=w2070:u16, "NewVal"=w2069:u16)  [unwired: 5 out]
        n1477 = local read "Type"() -> (w2072:u16)
        n1478 = Not Equal?(x=w2070, y=w2069) -> (x != y?=w2068:bool)
        n1479 = local read "Limit Cluster"() -> (w2076:T1)
        n1480 = case shown="False" w2068 {
          tunnel: [_ w2112] -> w2067
          frame False {
          }
          frame True {
            w2112 = TRUE ("Load state")
            w2113 = FALSE ("Visible")
            w2114 = FALSE ("Visible")
            n1481 = property on="UpAlignRst_1" class="Str"("Visible"=w2114) -> ()  [unwired: 2 in, 2 out]
            n1482 = property on="UpAlignRst_2" class="Str"("Visible"=w2113) -> ()  [unwired: 2 in, 2 out]
            n1483 = local write "Load state"(w2112) -> ()
            n1484 = property on="DataAlignRst" class="Str"("Visible"=w2114) -> ()  [unwired: 2 in, 2 out]
            n1485 = property on="LowAlignRst_2" class="Str"("Visible"=w2113) -> ()  [unwired: 2 in, 2 out]
            n1486 = property on="LowAlignRst_1" class="Str"("Visible"=w2114) -> ()  [unwired: 2 in, 2 out]
          }
        }
        n1487 = Bundle By Name(cluster=w2076, "Tolerance"=w2069) -> (w2075:T1)
        n1488 = Equal?(x=w2069, y=u16 4) -> (x = y?=w2080:bool)
        n1489 = Equal?(x=w2069, y=u16 5) -> (x = y?=w2079:bool)
        n1490 = local write "Limit Cluster"(w2075) -> ()
        n1491 = Or(x=w2080, y=w2079) -> (x .or. y?=w2073:bool)
        n1492 = property on="Limits Graph" class="XYGraph (strict)"("Active Plot"=u32 4, "Plot.Visible?"=w2073) -> ()  [unwired: 2 in, 2 out]
        n1493 = flat-sequence {
          tunnel: w2072 -> [w2092]
          tunnel: w2069 -> [w2091]
          tunnel: w2067 -> [_]
          frame #0 {
            n1494 = case shown="1, 2" w2092 {
              tunnel: w2091 -> [_ w2093]
              frame Default {
              }
              frame 1, 2 {
                n1495 = In Range and Coerce(upper limit=u16 4 ("hi"), x=w2093, lower limit=u16 2 ("lo")) -> (In Range?=w2100:bool)  [unwired: 1 out]
                n1496 = In Range and Coerce(upper limit=u16 6 ("hi"), x=w2093, lower limit=u16 4 ("y")) -> (In Range?=w2095:bool)  [unwired: 1 out]
                n1497 = case shown="True" w2100 {
                  frame False {
                    n1498 = local read "Limits_Ring"() -> (w2103:u16)
                    n1499 = property on="Limits_Ring" class="Ring (strict)"("Disabled"=u16 0 ("x"), "Val(Sgnl)"=w2103) -> ()  [unwired: 2 in, 2 out]
                  }
                  frame True {
                    w2108 = u16 2 items=["Upper Only", "Lower Only", "Upper & Lower"] ("Limits")
                    n1500 = property on="Limits_Ring" class="Ring (strict)"("Disabled"=u16 2 ("x")) -> ()  [unwired: 2 in, 2 out]
                    n1501 = local read "Limits_Ring"() -> (w2107:u16)
                    n1502 = Not Equal?(x=w2108, y=w2107) -> (x != y?=w2106:bool)
                    n1503 = case shown="True" w2106 {
                      frame False {
                      }
                      frame True {
                        w2110 = u16 2 items=["Upper Only", "Lower Only", "Upper & Lower"] ("Limits")
                        n1504 = disable-structure shown="Disabled" {
                          frame Disabled {
                            n1505 = local read "Load state"() -> ()  [unwired: 1 out]
                          }
                          frame Enabled {
                          }
                        }
                        n1506 = local write "Limits_Ring"(w2110) -> ()
                        n1507 = case shown="False" FALSE {
                          tunnel: w2110 -> [w2111 _]
                          frame False {
                            n1508 = property on="Limits_Ring" class="Ring (strict)"("Val(Sgnl)"=w2111) -> ()  [unwired: 2 in, 2 out]
                          }
                          frame True {
                          }
                        }
                      }
                    }
                  }
                }
                n1509 = Select(t=u8 0, s=w2095, f=u8 2) -> (s? t:f=w2094:u8)
                n1510 = property on="X AlignRef" class="DigNum (strict)"("Disabled"=w2094) -> ()  [unwired: 2 in, 2 out]
                n1511 = property on="Y AlignRef" class="DigNum (strict)"("Disabled"=w2094) -> ()  [unwired: 2 in, 2 out]
              }
            }
          }
        }
        n1512 = case shown="0" w2069 {
          tunnel: [u8 0 ("Write Attribute") u8 2 ("Write Attribute")] -> w2083
          tunnel: [u8 6 ("Write Attribute") u8 6 ("Write Attribute")] -> w2082
          tunnel: [u8 1 ("Write Attribute") u8 2 ("Write Attribute")] -> w2081
          tunnel: [i16 -4 ("Write Attribute") w2123] -> w2086
          tunnel: [u8 2 ("Write Attribute") u8 0 ("Write Attribute")] -> w2085
          tunnel: [i16 -3 ("Write Attribute") w2123] -> w2084
          frame 0 {
          }
          frame Default {
            w2123 = i16 -1 ("Write Attribute")
          }
        }
        n1513 = local read "Load state"() -> (w2071:bool)
        n1514 = case shown="True" w2071 {
          frame False {
          }
          frame True {
            n1515 = local read "Limits_Ring"() -> (w2115:u16)
            n1516 = local read "x float"() -> (w2116:bool)
            n1517 = property on="Limits_Ring" class="Ring (strict)"("Val(Sgnl)"=w2115) -> ()  [unwired: 2 in, 2 out]
            n1518 = property on="x float" class="Bool (strict)"("Val(Sgnl)"=w2116) -> ()  [unwired: 2 in, 2 out]
          }
        }
        n1519 = property on="Limits Graph" class="XYGraph (strict)"("Active Plot"=u32 1, "Plot.Plot Interpolation"=w2083, "Plot.Point Style"=w2082, "Plot.Line Width"=w2081, "Plot.Fill To"=w2086, "Active Plot"=u32 0, "Plot.Plot Interpolation"=u8 2, "Plot.Point Style"=w2085, "Plot.Line Width"=w2081, "Active Plot"=u32 2, "Plot.Plot Interpolation"=w2083, "Plot.Point Style"=w2082, "Plot.Line Width"=w2081, "Plot.Fill To"=w2084) -> ()  [unwired: 2 in, 2 out]
      }
      event "Limits_Ring": Value Change {
        n1520 = event-data() -> ("OldVal"=w2130:u16, "NewVal"=w2129:u16)  [unwired: 5 out]
        n1521 = local read "Type"() -> (w2132:u16)
        n1522 = Not Equal?(x=w2130, y=w2129) -> (x != y?=w2128:bool)
        n1523 = local read "Limit Cluster"() -> (w2133:T1)
        n1524 = case shown="True" w2128 {
          frame False {
          }
          frame True {
            n1525 = local write "Load state"(TRUE ("Load state")) -> ()
          }
        }
        n1526 = Equal To 0?(x=w2132) -> (x = 0?=w2134:bool)
        n1527 = Equal?(x=w2132, y=u16 3) -> (x = y?=w2136:bool)
        n1528 = Or(x=w2134, y=w2136) -> (x .or. y?=w2135:bool)
        n1529 = Bundle By Name(cluster=w2133, "Type"=w2132, "Limits"=w2129) -> (w2131:T1)
        n1530 = local write "Limit Cluster"(w2131) -> ()
        n1531 = case shown="True" w2135 {
          tunnel: w2129 -> [w2144 w2160]
          tunnel: w2128 -> [w2143 _]
          frame False {
            n1532 = local read "Alignment"() -> (w2140:u16)
            n1533 = case shown="2" w2144 {
              frame 0, Default {
                w2150 = TRUE ("Visible")
                w2151 = FALSE ("Visible")
                n1534 = property on="Lower Limit" class="Bool (strict)"("Visible"=w2151) -> ()  [unwired: 2 in, 2 out]
                n1535 = property on="Upper Limit" class="Bool (strict)"("Visible"=w2150) -> ()  [unwired: 2 in, 2 out]
                n1536 = local read "UpSource"() -> (w2149:u16)
                n1537 = property on="Sub3 Tab" class="TabCtl (strict)"("Visible"=w2151) -> ()  [unwired: 2 in, 2 out]
                n1538 = property on="UpSource" class="Slide (strict)"("Visible"=w2150) -> ()  [unwired: 2 in, 2 out]
                n1539 = property on="Sub5 Tab" class="TabCtl (strict)"("Visible"=w2151) -> ()  [unwired: 2 in, 2 out]
                n1540 = property on="UpSource" class="Slide (strict)"("Val(Sgnl)"=w2149) -> ()  [unwired: 2 in, 2 out]
                n1541 = property on="Sub7 Tab" class="TabCtl (strict)"("Visible"=w2151) -> ()  [unwired: 2 in, 2 out]
                n1542 = local write "Plot index"(1 ("Plot index")) -> ()
                n1543 = property on="LoSource" class="Slide (strict)"("Visible"=w2151) -> ()  [unwired: 2 in, 2 out]
              }
              frame 1 {
                w2153 = FALSE ("Visible")
                w2155 = TRUE ("Visible")
                n1544 = property on="Lower Limit" class="Bool (strict)"("Visible"=w2155) -> ()  [unwired: 2 in, 2 out]
                n1545 = property on="Sub2 Tab" class="TabCtl (strict)"("Visible"=w2153) -> ()  [unwired: 2 in, 2 out]
                n1546 = local read "LoSource"() -> (w2154:u16)
                n1547 = property on="Sub4 Tab" class="TabCtl (strict)"("Visible"=w2153) -> ()  [unwired: 2 in, 2 out]
                n1548 = property on="LoSource" class="Slide (strict)"("Visible"=w2155) -> ()  [unwired: 2 in, 2 out]
                n1549 = property on="LoSource" class="Slide (strict)"("Val(Sgnl)"=w2154) -> ()  [unwired: 2 in, 2 out]
                n1550 = property on="Sub6 Tab" class="TabCtl (strict)"("Visible"=w2153) -> ()  [unwired: 2 in, 2 out]
                n1551 = property on="UpSource" class="Slide (strict)"("Visible"=w2153) -> ()  [unwired: 2 in, 2 out]
                n1552 = local write "Plot index"(2 ("Plot index")) -> ()
                n1553 = property on="Upper Limit" class="Bool (strict)"("Visible"=w2153) -> ()  [unwired: 2 in, 2 out]
              }
              frame 2 {
                w2159 = TRUE ("Visible")
                n1554 = property on="Upper Limit" class="Bool (strict)"("Visible"=w2159) -> ()  [unwired: 2 in, 2 out]
                n1555 = local read "UpSource"() -> (w2158:u16)
                n1556 = local read "LoSource"() -> (w2157:u16)
                n1557 = property on="UpSource" class="Slide (strict)"("Visible"=w2159) -> ()  [unwired: 2 in, 2 out]
                n1558 = property on="LoSource" class="Slide (strict)"("Val(Sgnl)"=w2157) -> ()  [unwired: 2 in, 2 out]
                n1559 = property on="UpSource" class="Slide (strict)"("Val(Sgnl)"=w2158) -> ()  [unwired: 2 in, 2 out]
                n1560 = property on="Lower Limit" class="Bool (strict)"("Visible"=w2159) -> ()  [unwired: 2 in, 2 out]
                n1561 = property on="LoSource" class="Slide (strict)"("Visible"=w2159) -> ()  [unwired: 2 in, 2 out]
                n1562 = local write "Plot index"(1 ("Plot index")) -> ()
              }
            }
            n1563 = Greater Or Equal?(x=w2140, y=u16 4) -> (x >= y?=w2141:bool)
            n1564 = And(x=w2143, y=w2141) -> (x .and. y?=w2142:bool)
            n1565 = case shown="True" w2142 {
              frame False {
              }
              frame True {
                n1566 = flat-sequence {
                  tunnel: [w2146] -> w2145
                  tunnel: w2145 -> [w2147]
                  frame #0 {
                    w2146 = 0.0 ("X AlignRef")
                    n1567 = local write "X AlignRef"(w2146) -> ()
                    n1568 = local write "Y AlignRef"(w2146) -> ()
                  }
                  frame #1 {
                    n1569 = property on="X AlignRef" class="DigNum (strict)"("Val(Sgnl)"=w2147) -> ()  [unwired: 2 in, 2 out]
                  }
                }
              }
            }
          }
          frame True {
            n1570 = case shown="2" w2160 {
              frame 0, Default {
                w2162 = TRUE ("Visible")
                w2161 = FALSE ("Visible")
                n1571 = property on="Lower Limit" class="Bool (strict)"("Visible"=w2161) -> ()  [unwired: 2 in, 2 out]
                n1572 = property on="LoSource" class="Slide (strict)"("Visible"=w2161) -> ()  [unwired: 2 in, 2 out]
                n1573 = property on="Single Limit" class="Slide (strict)"("Visible"=w2162, "BG Color"=u32 16860) -> ()  [unwired: 2 in, 2 out]
                n1574 = local read "UpSource"() -> (w2163:u16)
                n1575 = property on="Sub3 Tab" class="TabCtl (strict)"("Visible"=w2161) -> ()  [unwired: 2 in, 2 out]
                n1576 = property on="Multi Limit" class="Slide (strict)"("Visible"=w2161) -> ()  [unwired: 2 in, 2 out]
                n1577 = property on="Up tip" class="Str"("Visible"=w2162) -> ()  [unwired: 2 in, 2 out]
                n1578 = property on="UpSource" class="Slide (strict)"("Val(Sgnl)"=w2163) -> ()  [unwired: 2 in, 2 out]
                n1579 = property on="Sub5 Tab" class="TabCtl (strict)"("Visible"=w2161) -> ()  [unwired: 2 in, 2 out]
                n1580 = property on="Lo tip" class="Str"("Visible"=w2161) -> ()  [unwired: 2 in, 2 out]
                n1581 = property on="Upper Limit" class="Bool (strict)"("Visible"=w2162) -> ()  [unwired: 2 in, 2 out]
                n1582 = property on="Sub7 Tab" class="TabCtl (strict)"("Visible"=w2161) -> ()  [unwired: 2 in, 2 out]
                n1583 = property on="UpSource" class="Slide (strict)"("Visible"=w2162) -> ()  [unwired: 2 in, 2 out]
              }
              frame 1 {
                w2166 = TRUE ("Visible")
                w2165 = FALSE ("Visible")
                n1584 = property on="UpSource" class="Slide (strict)"("Visible"=w2165) -> ()  [unwired: 2 in, 2 out]
                n1585 = property on="Sub2 Tab" class="TabCtl (strict)"("Visible"=w2165) -> ()  [unwired: 2 in, 2 out]
                n1586 = property on="Single Limit" class="Slide (strict)"("Visible"=w2166, "BG Color"=u32 16754242) -> ()  [unwired: 2 in, 2 out]
                n1587 = local read "LoSource"() -> (w2167:u16)
                n1588 = property on="Upper Limit" class="Bool (strict)"("Visible"=w2165) -> ()  [unwired: 2 in, 2 out]
                n1589 = property on="Sub4 Tab" class="TabCtl (strict)"("Visible"=w2165) -> ()  [unwired: 2 in, 2 out]
                n1590 = property on="Lo tip" class="Str"("Visible"=w2166) -> ()  [unwired: 2 in, 2 out]
                n1591 = property on="LoSource" class="Slide (strict)"("Val(Sgnl)"=w2167) -> ()  [unwired: 2 in, 2 out]
                n1592 = property on="Sub6 Tab" class="TabCtl (strict)"("Visible"=w2165) -> ()  [unwired: 2 in, 2 out]
                n1593 = property on="Multi Limit" class="Slide (strict)"("Visible"=w2165) -> ()  [unwired: 2 in, 2 out]
                n1594 = property on="Lower Limit" class="Bool (strict)"("Visible"=w2166) -> ()  [unwired: 2 in, 2 out]
                n1595 = property on="Up tip" class="Str"("Visible"=w2165) -> ()  [unwired: 2 in, 2 out]
                n1596 = property on="LoSource" class="Slide (strict)"("Visible"=w2166) -> ()  [unwired: 2 in, 2 out]
              }
              frame 2 {
                w2169 = TRUE ("Visible")
                n1597 = property on="Multi Limit" class="Slide (strict)"("Visible"=w2169) -> ()  [unwired: 2 in, 2 out]
                n1598 = property on="Upper Limit" class="Bool (strict)"("Visible"=w2169) -> ()  [unwired: 2 in, 2 out]
                n1599 = property on="Single Limit" class="Slide (strict)"("Visible"=FALSE) -> ()  [unwired: 2 in, 2 out]
                n1600 = property on="Lo tip" class="Str"("Visible"=w2169) -> ()  [unwired: 2 in, 2 out]
                n1601 = property on="UpSource" class="Slide (strict)"("Visible"=w2169) -> ()  [unwired: 2 in, 2 out]
                n1602 = local read "UpSource"() -> (w2170:u16)
                n1603 = local read "LoSource"() -> (w2171:u16)
                n1604 = property on="Up tip" class="Str"("Visible"=w2169) -> ()  [unwired: 2 in, 2 out]
                n1605 = property on="Lower Limit" class="Bool (strict)"("Visible"=w2169) -> ()  [unwired: 2 in, 2 out]
                n1606 = property on="UpSource" class="Slide (strict)"("Val(Sgnl)"=w2170) -> ()  [unwired: 2 in, 2 out]
                n1607 = property on="LoSource" class="Slide (strict)"("Val(Sgnl)"=w2171) -> ()  [unwired: 2 in, 2 out]
                n1608 = property on="LoSource" class="Slide (strict)"("Visible"=w2169) -> ()  [unwired: 2 in, 2 out]
              }
            }
          }
        }
      }
      event "Out Fail": Value Change {
        n1609 = event-data() -> ("NewVal"=w2182:bool)  [unwired: 6 out]
        n1610 = property on="Type" class="Slide (strict)"() -> ("Value"=w2176:u16)  [unwired: 2 in, 2 out]
        n1611 = local read "Limit Cluster"() -> (w2177:T1)
        n1612 = Bundle By Name(cluster=w2177, "Output failed point curves?"=w2182) -> (w2173:T1)
        n1613 = Equal?(x=u16 1, y=w2176) -> (x = y?=w2174:bool)
        n1614 = Equal?(x=w2176, y=u16 2) -> (x = y?=w2180:bool)
        n1615 = Or(x=w2174, y=w2180) -> (x .or. y?=w2181:bool)
        n1616 = local write "Limit Cluster"(w2173) -> ()
        n1617 = property on="Limits_Ring" class="Ring (strict)"() -> ("Value"=w2178:u16)  [unwired: 2 in, 2 out]
        n1618 = case shown="True" w2181 {
          tunnel: w2182 -> [_ w2185]
          tunnel: w2178 -> [_ w2186]
          frame False {
          }
          frame True {
            n1619 = case shown="0, Default" w2186 {
              tunnel: w2185 -> [w2191 w2198 w2203]
              tunnel: [w2190 w2197 w2203] -> w2188
              tunnel: [w2189 w2196 w2203] -> w2187
              frame 0, Default {
                n1620 = case shown="True" w2191 {
                  tunnel: [FALSE ("Plot.Visible") TRUE ("Plot.Visible")] -> w2190
                  tunnel: [FALSE ("Plot.Visible") FALSE ("Plot.Visible")] -> w2189
                  frame False {
                  }
                  frame True {
                  }
                }
              }
              frame 1 {
                n1621 = case shown="False" w2198 {
                  tunnel: [FALSE ("Plot.Visible") FALSE ("Plot.Visible")] -> w2197
                  tunnel: [FALSE ("Plot.Visible") TRUE ("Plot.Visible")] -> w2196
                  frame False {
                  }
                  frame True {
                  }
                }
              }
              frame 2 {
              }
            }
            n1622 = property on="Limits Graph" class="XYGraph (strict)"("Active Plot"=u32 5, "Plot.Visible?"=w2188, "Active Plot"=u32 6, "Plot.Visible?"=w2187) -> ()  [unwired: 2 in, 2 out]
          }
        }
      }
      event "Mapping": Value Change {
        n1623 = event-data() -> ("NewVal"=w2212:u16)  [unwired: 6 out]
        n1624 = property on="Type" class="Slide (strict)"() -> ("Value"=w2206:u16)  [unwired: 2 in, 2 out]
        n1625 = Equal?(x=u16 1, y=w2206) -> (x = y?=w2208:bool)
        n1626 = Equal?(x=w2206, y=u16 2) -> (x = y?=w2210:bool)
        n1627 = local read "Limit Cluster"() -> (w2211:T1)
        n1628 = Or(x=w2208, y=w2210) -> (x .or. y?=w2205:bool)
        n1629 = Bundle By Name(cluster=w2211, "X Axis"=w2212) -> (w2204:T1)
        n1630 = case shown="True" w2205 {
          tunnel: w2212 -> [_ w2214]
          tunnel: w2206 -> [_ w2213]
          frame False {
          }
          frame True {
            n1631 = case shown="0, Default" w2214 {
              tunnel: w2213 -> [w2215 _]
              frame 0, Default {
                n1632 = case shown="2, Default" w2215 {
                  tunnel: ["s" ("size_unit") "Hz" ("size_unit")] -> w2216
                  frame 2, Default {
                  }
                  frame 1 {
                  }
                }
                n1633 = local write "size_unit"(w2216) -> ()
              }
              frame 1 {
                n1634 = local write "size_unit"("%" ("size_unit")) -> ()
              }
            }
          }
        }
        n1635 = local write "Limit Cluster"(w2204) -> ()
      }
      event "x float": Value Change {
        n1636 = event-data() -> ("NewVal"=w2228:bool)  [unwired: 6 out]
        n1637 = property on="Type" class="Slide (strict)"() -> ("Value"=w2223:u16)  [unwired: 2 in, 2 out]
        n1638 = Equal?(x=u16 1, y=w2223) -> (x = y?=w2221:bool)
        n1639 = Equal?(x=w2223, y=u16 2) -> (x = y?=w2226:bool)
        n1640 = Or(x=w2221, y=w2226) -> (x .or. y?=w2227:bool)
        n1641 = local read "Limit Cluster"() -> (w2224:T1)
        n1642 = case shown="True" w2227 {
          tunnel: w2228 -> [_ w2229]
          frame False {
          }
          frame True {
            n1643 = Select(t=u8 0, s=w2229, f=u8 2 ("Disabled")) -> (s? t:f=w2232:u8)
            n1644 = property on="size_unit" class="Str"("Disabled"=w2232) -> ()  [unwired: 2 in, 2 out]
            n1645 = property on="Minimum" class="DigNum (strict)"("Disabled"=w2232) -> ()  [unwired: 2 in, 2 out]
            n1646 = property on="Maximum" class="DigNum (strict)"("Disabled"=w2232) -> ()  [unwired: 2 in, 2 out]
            n1647 = property on="Step Size" class="DigNum (strict)"("Disabled"=w2232) -> ()  [unwired: 2 in, 2 out]
          }
        }
        n1648 = Bundle By Name(cluster=w2224, "x float"=w2228) -> (w2220:T1)
        n1649 = local write "Limit Cluster"(w2220) -> ()
      }
      event "X Resolution", "Y Resolution": Value Change {
        n1650 = event-data() -> ()  [unwired: 7 out]
        n1651 = local read "Limit Cluster"() -> (w2253:T1)
        n1652 = local read "X Resolution"() -> (w2261:u8)
        n1653 = local read "Y Resolution"() -> (w2258:u8)
        n1654 = Unbundle By Name(w2253) -> ("Upper Limit"=w2255:cluster{dbl, dbl}[], "Lower Limit"=w2254:cluster{dbl, dbl}[])
        n1655 = Greater?(x=w2261, y=u8 30) -> (0:w2262:bool)
        n1656 = Greater?(x=w2258, y=u8 30) -> (0:w2260:bool)
        n1657 = local read "Type"() -> (w2246:u16)
        n1658 = case shown="True" w2260 {
          tunnel: w2258 -> [w2294 _]
          tunnel: [w2294 u8 30 ("NewVal")] -> w2236
          frame False {
          }
          frame True {
          }
        }
        n1659 = case shown="True" w2262 {
          tunnel: w2261 -> [w2296 _]
          tunnel: [w2296 u8 30 ("NewVal")] -> w2244
          frame False {
          }
          frame True {
          }
        }
        n1660 = case shown="1" w2246 {
          tunnel: w2244 -> [_ w2267 _]
          tunnel: w2236 -> [_ w2266 _]
          frame 0, Default {
            n1661 = local write "Plot Multilimit"(TRUE ("Plot Multilimit")) -> ()
          }
          frame 1 {
            n1662 = disable-structure shown="Disabled" {
              frame Disabled {
                n1663 = local write "Plot graphs"(TRUE ("Plot graphs")) -> ()
              }
              frame Enabled {
              }
            }
            n1664 = global read "CRYLimit edit global.vi" "Data"() -> (w2268:cluster{"x":dbl, "y":dbl}[])
            n1665 = call "CRYCurve to Table.vi"("y precision"=w2266, "Margin"=TRUE, "x precision"=w2267, "Limit curve In"=w2268) -> ("Limit Table"=w2269:string[][])  [unwired: 7 out]
            n1666 = local write "Data Table"(w2269) -> ()
          }
          frame 2 {
            n1667 = disable-structure shown="Disabled" {
              frame Disabled {
                n1668 = local write "Plot graphs"(TRUE ("Plot graphs")) -> ()
              }
              frame Enabled {
              }
            }
          }
        }
        n1669 = property on="Limits Graph" class="XYGraph (strict)"("YScale.Precision"=w2236) -> ()  [unwired: 2 in, 2 out]
        n1670 = local read "Up_type"() -> (w2251:enum32{"Single Values", "Curves", "Waveforms"})
        n1671 = local read "UpSource"() -> (w2257:u16)
        n1672 = local read "Lo_type"() -> (w2249:enum32{"Single Values", "Curves", "Waveforms"})
        n1673 = local read "LoSource"() -> (w2256:u16)
        n1674 = property on="Limits Graph" class="XYGraph (strict)"("XScale.Precision"=w2244) -> ()  [unwired: 2 in, 2 out]
        n1675 = Bundle By Name(cluster=w2253, "X-Resolution"=w2244, "Y-Resolution"=w2236) -> (w2245:T1)
        n1676 = property on="UpSingleVal" class="DigNum (strict)"("Precision"=w2236) -> ()  [unwired: 2 in, 2 out]
        n1677 = Equal?(x=w2251, y=enum32{"Single Values", "Curves", "Waveforms"}."Waveforms") -> (x = y?=w2250:bool)
        n1678 = case shown="1" w2257 {
          tunnel: w2255 -> [w2286 _]
          tunnel: w2244 -> [w2285 w2289]
          tunnel: w2236 -> [w2284 w2288]
          tunnel: w2250 -> [_ w2287]
          frame 0, Default {
            n1679 = call "CRYCurve to Table.vi"("y precision"=w2284, "x precision"=w2285, "Limit curve In"=w2286) -> ("Limit Table"=w2283:string[][])  [unwired: 1 in, 7 out]
            n1680 = local write "UpTable_1"(w2283) -> ()
          }
          frame 1 {
            n1681 = case shown="False" w2287 {
              tunnel: w2289 -> [w2293 _]
              tunnel: w2288 -> [w2292 _]
              frame False {
                n1682 = local read "Up Limit Data"() -> (w2290:cluster{"x":dbl, "y":dbl}[])
                n1683 = call "CRYCurve to Table.vi"("y precision"=w2292, "x precision"=w2293, "Limit curve In"=w2290) -> ("Limit Table"=w2291:string[][])  [unwired: 1 in, 7 out]
                n1684 = local write "UpTable_2"(w2291) -> ()
              }
              frame True {
              }
            }
          }
        }
        n1685 = property on="Multi value" class="Slide (strict)"("Scale.Precision"=w2236) -> ()  [unwired: 2 in, 2 out]
        n1686 = local write "Limit Cluster"(w2245) -> ()
        n1687 = Equal?(x=w2249, y=enum32{"Single Values", "Curves", "Waveforms"}."Waveforms") -> (x = y?=w2247:bool)
        n1688 = local read "Raw DataVal"() -> (w2243:dbl)
        n1689 = local read "RawUp Limit"() -> (w2239:dbl)
        n1690 = case shown="1" w2256 {
          tunnel: w2254 -> [w2275 _]
          tunnel: w2244 -> [w2273 w2278]
          tunnel: w2236 -> [w2272 w2277]
          tunnel: w2247 -> [_ w2276]
          frame 0, Default {
            n1691 = call "CRYCurve to Table.vi"("y precision"=w2272, "x precision"=w2273, "Limit curve In"=w2275) -> ("Limit Table"=w2274:string[][])  [unwired: 1 in, 7 out]
            n1692 = local write "LoTable_1"(w2274) -> ()
          }
          frame 1 {
            n1693 = case shown="False" w2276 {
              tunnel: w2278 -> [w2281 _]
              tunnel: w2277 -> [w2280 _]
              frame False {
                n1694 = local read "Lo Limit Data"() -> (w2279:cluster{"x":dbl, "y":dbl}[])
                n1695 = call "CRYCurve to Table.vi"("y precision"=w2280, "x precision"=w2281, "Limit curve In"=w2279) -> ("Limit Table"=w2282:string[][])  [unwired: 1 in, 7 out]
                n1696 = local write "LoTable_2"(w2282) -> ()
              }
              frame True {
              }
            }
          }
        }
        n1697 = local read "RawLo Limit"() -> (w2235:dbl)
        n1698 = property class="DigNum (strict)"("Precision"=w2236) -> ()  [unwired: 2 in, 2 out]
        n1699 = call "CRYRepresent numeric by precission.vi"("Pprecision"=w2236, "Numeric In"=w2243) -> ("Out Format"=w2240:string, "output string"=w2241:string, "Numeric Out"=w2242:dbl)  [unwired: 7 in]
        n1700 = call "CRYRepresent numeric by precission.vi"("Pprecision"=w2236, "Numeric In"=w2239) -> ("Out Format"=w2237:string, "Numeric Out"=w2238:dbl)  [unwired: 7 in, 1 out]
        n1701 = call "CRYRepresent numeric by precission.vi"("Pprecision"=w2236, "Numeric In"=w2235) -> ("Out Format"=w2233:string, "Numeric Out"=w2234:dbl)  [unwired: 7 in, 1 out]
        n1702 = property on="LoSingleVal" class="DigNum (strict)"("Precision"=w2236) -> ()  [unwired: 2 in, 2 out]
        n1703 = property on="Data Value" class="DigNum (strict)"("Value"=w2242, "FormatString"=w2240) -> ()  [unwired: 2 in, 2 out]
        n1704 = property class="DigNum (strict)"("NumText.Text"=w2241, "FormatString"=w2240) -> ()  [unwired: 2 in, 2 out]
        n1705 = property on="Up Limit Val" class="DigNum (strict)"("Value"=w2238, "FormatString"=w2237) -> ()  [unwired: 2 in, 2 out]
        n1706 = property on="Lo Limit Val" class="DigNum (strict)"("Value"=w2234, "FormatString"=w2233) -> ()  [unwired: 2 in, 2 out]
      }
      event "X Up Val": Value Change {
        n1707 = event-data() -> ("NewVal"=w2298:dbl)  [unwired: 6 out]
        n1708 = local read "Limit Cluster"() -> (w2300:T1)
        n1709 = Bundle By Name(cluster=w2300, "X Up Val"=w2298) -> (w2299:T1)
        n1710 = local write "Limit Cluster"(w2299) -> ()
      }
      event "Y Up Val": Value Change {
        n1711 = event-data() -> ("NewVal"=w2301:dbl)  [unwired: 6 out]
        n1712 = local read "Limit Cluster"() -> (w2303:T1)
        n1713 = Bundle By Name(cluster=w2303, "Y Up Val"=w2301) -> (w2302:T1)
        n1714 = local write "Limit Cluster"(w2302) -> ()
      }
      event "X Lo Val": Value Change {
        n1715 = event-data() -> ("NewVal"=w2304:dbl)  [unwired: 6 out]
        n1716 = local read "Limit Cluster"() -> (w2306:T1)
        n1717 = Bundle By Name(cluster=w2306, "X Low Val"=w2304) -> (w2305:T1)
        n1718 = local write "Limit Cluster"(w2305) -> ()
      }
      event "Y Lo Val": Value Change {
        n1719 = event-data() -> ("NewVal"=w2307:dbl)  [unwired: 6 out]
        n1720 = local read "Limit Cluster"() -> (w2309:T1)
        n1721 = Bundle By Name(cluster=w2309, "Y Low Val"=w2307) -> (w2308:T1)
        n1722 = local write "Limit Cluster"(w2308) -> ()
      }
      event "Offset Upper": Value Change {
        n1723 = event-data() -> ()  [unwired: 7 out]
        n1724 = case shown="True" "Offset Upper" {
          frame False {
          }
          frame True {
            n1725 = local read "Upp y Unit"() -> (w2312:u16)
            n1726 = local read "Upp x Unit"() -> (w2311:u16)
            n1727 = local read "Type"() -> (w2313:u16)
            n1728 = case shown="1, 2, Default" w2313 {
              tunnel: w2312 -> [w2315 w2356]
              tunnel: w2311 -> [_ w2340]
              frame 0, 3 {
                n1729 = case shown="1" w2315 {
                  tunnel: [w2316 w2319] -> w2314
                  frame 0, Default {
                    n1730 = local read "Up Limit Val"() -> (w2318:dbl)
                    n1731 = local read "Y Up Val"() -> (w2317:dbl)
                    n1732 = Add(x=w2318, y=w2317) -> (x+y=w2316:dbl)
                  }
                  frame 1 {
                    n1733 = local read "up single unit"() -> (w2322:string)
                    n1734 = Equal?(x=w2322, y="dB") -> (x = y?=w2320:bool)
                    n1735 = case shown="True" w2320 {
                      tunnel: [w2323 w2330] -> w2319
                      frame False {
                        n1736 = local read "Up Limit Val"() -> (w2324:dbl)
                        n1737 = local read "Y Up Val"() -> (w2329:dbl)
                        n1738 = Divide(x=w2329, y=100.0) -> (x/y=w2327:dbl)
                        n1739 = Add(x=1.0, y=w2327) -> (x+y=w2325:dbl)
                        n1740 = Multiply(x=w2324, y=w2325) -> (x*y=w2323:dbl)
                      }
                      frame True {
                        n1741 = local read "Up Limit Val"() -> (w2336:dbl)
                        n1742 = local read "Y Up Val"() -> (w2335:dbl)
                        n1743 = Divide(x=w2335, y=100.0) -> (x/y=w2333:dbl)
                        n1744 = call "CRYConversion dB-Lin.vi"("Log In"=w2336) -> ("Lin Out"=w2338:dbl)  [unwired: 5 in, 3 out]
                        n1745 = Add(x=1.0, y=w2333) -> (x+y=w2331:dbl)
                        n1746 = Multiply(x=w2338, y=w2331) -> (x*y=w2337:dbl)
                        n1747 = call "CRYConversion dB-Lin.vi"("Lin In"=w2337) -> ("Log Out"=w2330:dbl)  [unwired: 5 in, 3 out]
                      }
                    }
                  }
                }
                n1748 = property on="Up Limit Val" class="DigNum (strict)"("Val(Sgnl)"=w2314) -> ()  [unwired: 2 in, 2 out]
              }
              frame 1, 2, Default {
                n1749 = local read "UpTable_1"() -> (w2343:string[][])
                n1750 = call "CRYTable Empty Ignore.vi"("Table In"=w2343) -> ("Table Out"=w2344:string[][])  [unwired: 10 in]
                n1751 = local read "X Up Val"() -> (w2349:dbl)
                n1752 = local read "Y Up Val"() -> (w2348:dbl)
                n1753 = property on="UpTable_1" class="Tbl (strict)"() -> ("Selection Start"=w2355:T5, "Selection Size"=w2354:T5)  [unwired: 2 in, 2 out]
                n1754 = call "CRYTable to Curve.vi"("Table In"=w2344) -> ("Limit curve"=w2342:cluster{"Numeric":dbl, "Numeric 2":dbl}[])  [unwired: 10 in]
                n1755 = local read "Y Resolution"() -> (w2345:u8)
                n1756 = local read "X Resolution"() -> (w2346:u8)
                n1757 = local read "data unit"() -> (w2351:string)
                n1758 = Unbundle(w2355) -> ("Column"=w2353:i32)  [unwired: 1 out]
                n1759 = Unbundle(w2354) -> ("Column"=w2352:i32)  [unwired: 1 out]
                n1760 = call "CRYLimit Table Offset.vi"("Limit in"=w2342, "Data unit"=w2351, "X offset"=w2349, "Y offset"=w2348, "Starting Column"=w2353, "Number of columns"=w2352, "x Unit"=w2340, "y Unit"=w2356) -> ("Limit out"=w2347:cluster{"Numeric":dbl, "Log Out":dbl}[])  [unwired: 2 in, 5 out]
                n1761 = local read "Limit Cluster"() -> (w2350:T1)
                n1762 = Bundle By Name(cluster=w2350, "Upper Limit"=w2347) -> (w2341:T1)
                n1763 = call "CRYCurve to Table.vi"("y precision"=w2345, "x precision"=w2346, "Limit curve In"=w2347) -> ("Limit Table"=w2339:string[][])  [unwired: 1 in, 7 out]
                n1764 = flat-sequence {
                  tunnel: w2339 -> [w2357]
                  frame #0 {
                    n1765 = local write "UpTable_1"(w2357) -> ()
                  }
                  frame #1 {
                    n1766 = local write "Plot graphs"(TRUE ("Plot graphs")) -> ()
                  }
                }
                n1767 = local write "Limit Cluster"(w2341) -> ()
              }
            }
          }
        }
      }
      event "Offset Lower": Value Change {
        n1768 = event-data() -> ()  [unwired: 7 out]
        n1769 = case shown="True" "Offset Lower" {
          frame False {
          }
          frame True {
            n1770 = local read "Low y Unit"() -> (w2360:u16)
            n1771 = local read "Low x Unit"() -> (w2361:u16)
            n1772 = local read "Type"() -> (w2362:u16)
            n1773 = case shown="1, 2, Default" w2362 {
              tunnel: w2361 -> [_ w2405]
              tunnel: w2360 -> [w2364 w2404]
              frame 0, 3 {
                n1774 = case shown="1" w2364 {
                  tunnel: [w2365 w2368] -> w2363
                  frame 0, Default {
                    n1775 = local read "Lo Limit Val"() -> (w2367:dbl)
                    n1776 = local read "Y Lo Val"() -> (w2366:dbl)
                    n1777 = Add(x=w2367, y=w2366) -> (x+y=w2365:dbl)
                  }
                  frame 1 {
                    n1778 = local read "lo single unit"() -> (w2369:string)
                    n1779 = Equal?(x=w2369, y="dB") -> (x = y?=w2370:bool)
                    n1780 = case shown="True" w2370 {
                      tunnel: [w2372 w2379] -> w2368
                      frame False {
                        n1781 = local read "Y Lo Val"() -> (w2378:dbl)
                        n1782 = local read "Lo Limit Val"() -> (w2373:dbl)
                        n1783 = Divide(x=w2378, y=100.0) -> (x/y=w2376:dbl)
                        n1784 = Add(x=1.0, y=w2376) -> (x+y=w2374:dbl)
                        n1785 = Multiply(x=w2373, y=w2374) -> (x*y=w2372:dbl)
                      }
                      frame True {
                        n1786 = local read "Lo Limit Val"() -> (w2385:dbl)
                        n1787 = local read "Y Lo Val"() -> (w2384:dbl)
                        n1788 = Divide(x=w2384, y=100.0) -> (x/y=w2382:dbl)
                        n1789 = call "CRYConversion dB-Lin.vi"("Log In"=w2385) -> ("Lin Out"=w2387:dbl)  [unwired: 5 in, 3 out]
                        n1790 = Add(x=1.0, y=w2382) -> (x+y=w2380:dbl)
                        n1791 = Multiply(x=w2387, y=w2380) -> (x*y=w2386:dbl)
                        n1792 = call "CRYConversion dB-Lin.vi"("Lin In"=w2386) -> ("Log Out"=w2379:dbl)  [unwired: 5 in, 3 out]
                      }
                    }
                  }
                }
                n1793 = property on="Lo Limit Val" class="DigNum (strict)"("Val(Sgnl)"=w2363) -> ()  [unwired: 2 in, 2 out]
              }
              frame 1, 2, Default {
                n1794 = local read "Y Lo Val"() -> (w2398:dbl)
                n1795 = local read "X Lo Val"() -> (w2399:dbl)
                n1796 = local read "LoTable_1"() -> (w2390:string[][])
                n1797 = property on="LoTable_1" class="Tbl (strict)"() -> ("Selection Start"=w2403:T5, "Selection Size"=w2402:T5)  [unwired: 2 in, 2 out]
                n1798 = local read "Y Resolution"() -> (w2392:u8)
                n1799 = local read "X Resolution"() -> (w2393:u8)
                n1800 = call "CRYTable Empty Ignore.vi"("Table In"=w2390) -> ("Table Out"=w2391:string[][])  [unwired: 10 in]
                n1801 = Unbundle(w2403) -> ("Column"=w2397:i32)  [unwired: 1 out]
                n1802 = Unbundle(w2402) -> ("Column"=w2396:i32)  [unwired: 1 out]
                n1803 = local read "data unit"() -> (w2400:string)
                n1804 = call "CRYTable to Curve.vi"("Table In"=w2391) -> ("Limit curve"=w2389:cluster{"Numeric":dbl, "Numeric 2":dbl}[])  [unwired: 10 in]
                n1805 = call "CRYLimit Table Offset.vi"("Limit in"=w2389, "Data unit"=w2400, "X offset"=w2399, "Y offset"=w2398, "Starting Column"=w2397, "Number of columns"=w2396, "x Unit"=w2405, "y Unit"=w2404) -> ("Limit out"=w2394:cluster{"Numeric":dbl, "Log Out":dbl}[])  [unwired: 2 in, 5 out]
                n1806 = local read "Limit Cluster"() -> (w2401:T1)
                n1807 = Bundle By Name(cluster=w2401, "Lower Limit"=w2394) -> (w2388:T1)
                n1808 = call "CRYCurve to Table.vi"("y precision"=w2392, "x precision"=w2393, "Limit curve In"=w2394) -> ("Limit Table"=w2395:string[][])  [unwired: 1 in, 7 out]
                n1809 = flat-sequence {
                  tunnel: w2395 -> [w2406]
                  frame #0 {
                    n1810 = local write "LoTable_1"(w2406) -> ()
                  }
                  frame #1 {
                    n1811 = local write "Plot graphs"(TRUE ("Plot graphs")) -> ()
                  }
                }
                n1812 = local write "Limit Cluster"(w2388) -> ()
              }
            }
          }
        }
      }
      event "Insert Upper": Value Change {
        n1813 = event-data() -> ()  [unwired: 7 out]
        n1814 = case shown="True" "Insert Upper" {
          frame False {
          }
          frame True {
            n1815 = control-ref of="UpTable_1"() -> (w2409:refnum<vi>)
            n1816 = call "CRYLimit Table Insert.vi"("Limit Table"=w2409) -> ()  [unwired: 3 in, 8 out]
          }
        }
      }
      event "Insert Lower": Value Change {
        n1817 = event-data() -> ()  [unwired: 7 out]
        n1818 = case shown="True" "Insert Lower" {
          frame False {
          }
          frame True {
            n1819 = control-ref of="LoTable_1"() -> (w2411:refnum<vi>)
            n1820 = call "CRYLimit Table Insert.vi"("Limit Table"=w2411) -> ()  [unwired: 3 in, 8 out]
          }
        }
      }
      event "UpTable_1": Value Change {
        n1821 = event-data() -> ("NewVal"=w2420:string[][])  [unwired: 6 out]
        n1822 = Transpose 2D Array(2D array=w2420) -> (transposed array=w2416:string[][])
        n1823 = for {
          tunnel: w2416 -> [w2433] mode=indexing
          shift-right: [w2429] -> w2412
          shift-left: cluster{dbl, dbl}[] [] -> [w2430]
          tunnel: [w2422] -> w2419 mode=indexing
          tunnel: [w2421] -> w2414 mode=indexing
          w2436 = "%_1p" ("format string")
          n1824 = Index Array(array=w2433, index=0 ("Index")) -> (element=w2424:string)
          n1825 = Index Array(array=w2433, index=1 ("Index")) -> (element=w2423:string)
          n1826 = Scan Value(string=w2424, format string=w2436) -> (value=w2439:dbl)  [unwired: 1 in, 1 out]
          n1827 = Scan Value(string=w2423, format string=w2436) -> (value=w2440:dbl)  [unwired: 1 in, 1 out]
          n1828 = Equal?(x=w2424, y="") -> (x = y?=w2432:bool)
          n1829 = Equal?(x=w2423, y="") -> (x = y?=w2431:bool)
          n1830 = Not Equal?(x=w2424, y="") -> (x != y?=w2427:bool)
          n1831 = Not Equal?(x=w2423, y="") -> (x != y?=w2428:bool)
          n1832 = And(x=w2432, y=w2431) -> (x .and. y?=w2422:bool)
          n1833 = And(x=w2427, y=w2428) -> (x .and. y?=w2421:bool)
          n1834 = case shown="False" w2422 {
            tunnel: w2440 -> [w2445 _]
            tunnel: w2439 -> [w2444 _]
            tunnel: [w2442 w2446] -> w2429
            tunnel: w2430 -> [w2443 w2446]
            frame False {
              n1835 = Bundle(w2444, w2445) -> (w2441:cluster{dbl, dbl})  [unwired: 1 out]
              n1836 = Insert Into Array(array=w2443, new element=w2441) -> (w2442:cluster{dbl, dbl}[])  [unwired: 1 in]
            }
            frame True {
            }
          }
        }
        n1837 = And Array Elements(Boolean array=w2414) -> (logical AND=w2417:bool)
        n1838 = Or Array Elements(Boolean array=w2419) -> (logical OR=w2418:bool)
        n1839 = Or(x=w2418, y=w2417) -> (x .or. y?=w2413:bool)
        n1840 = case shown="True" w2413 {
          tunnel: w2412 -> [_ w2448]
          frame False {
          }
          frame True {
            n1841 = Sort 1D Array(array=w2448) -> (sorted array=w2447:cluster{dbl, dbl}[])
            n1842 = local read "Y Resolution"() -> (w2450:u8)
            n1843 = local read "X Resolution"() -> (w2449:u8)
            n1844 = call "CRYCurve to Table.vi"("y precision"=w2450, "x precision"=w2449, "Limit curve In"=w2447) -> ("Limit Table"=w2451:string[][])  [unwired: 7 in, 1 out]
            n1845 = local write "UpTable_1"(w2451) -> ()
            n1846 = local read "Limit Cluster"() -> (w2453:T1)
            n1847 = Bundle By Name(cluster=w2453, "Upper Limit"=w2447) -> (w2454:T1)
            n1848 = local write "Limit Cluster"(w2454) -> ()
            n1849 = local write "Plot graphs"(TRUE ("Plot graphs")) -> ()
          }
        }
      }
      event "LoTable_1": Value Change {
        n1850 = event-data() -> ("NewVal"=w2463:string[][])  [unwired: 6 out]
        n1851 = Transpose 2D Array(2D array=w2463) -> (transposed array=w2458:string[][])
        n1852 = for {
          shift-right: [w2473] -> w2455
          shift-left: cluster{dbl, dbl}[] [] -> [w2474]
          tunnel: [w2466] -> w2462 mode=indexing
          tunnel: [w2465] -> w2457 mode=indexing
          tunnel: w2458 -> [w2464] mode=indexing
          w2479 = "%_1p" ("format string")
          n1853 = Index Array(array=w2464, index=0 ("Index")) -> (element=w2468:string)
          n1854 = Index Array(array=w2464, index=1 ("Index")) -> (element=w2467:string)
          n1855 = Scan Value(string=w2468, format string=w2479) -> (value=w2482:dbl)  [unwired: 1 in, 1 out]
          n1856 = Scan Value(string=w2467, format string=w2479) -> (value=w2483:dbl)  [unwired: 1 in, 1 out]
          n1857 = Equal?(x=w2468, y="") -> (x = y?=w2476:bool)
          n1858 = Equal?(x=w2467, y="") -> (x = y?=w2475:bool)
          n1859 = Not Equal?(x=w2468, y="") -> (x != y?=w2471:bool)
          n1860 = Not Equal?(x=w2467, y="") -> (x != y?=w2472:bool)
          n1861 = And(x=w2476, y=w2475) -> (x .and. y?=w2466:bool)
          n1862 = And(x=w2471, y=w2472) -> (x .and. y?=w2465:bool)
          n1863 = case shown="False" w2466 {
            tunnel: w2483 -> [w2488 _]
            tunnel: w2482 -> [w2487 _]
            tunnel: [w2485 w2489] -> w2473
            tunnel: w2474 -> [w2486 w2489]
            frame False {
              n1864 = Bundle(w2487, w2488) -> (w2484:cluster{dbl, dbl})  [unwired: 1 out]
              n1865 = Insert Into Array(array=w2486, new element=w2484) -> (w2485:cluster{dbl, dbl}[])  [unwired: 1 in]
            }
            frame True {
            }
          }
        }
        n1866 = And Array Elements(Boolean array=w2457) -> (logical AND=w2460:bool)
        n1867 = Or Array Elements(Boolean array=w2462) -> (logical OR=w2461:bool)
        n1868 = Or(x=w2461, y=w2460) -> (x .or. y?=w2456:bool)
        n1869 = case shown="True" w2456 {
          tunnel: w2455 -> [_ w2491]
          frame False {
          }
          frame True {
            n1870 = Sort 1D Array(array=w2491) -> (sorted array=w2490:cluster{dbl, dbl}[])
            n1871 = local read "Y Resolution"() -> (w2493:u8)
            n1872 = local read "X Resolution"() -> (w2492:u8)
            n1873 = call "CRYCurve to Table.vi"("y precision"=w2493, "x precision"=w2492, "Limit curve In"=w2490) -> ("Limit Table"=w2494:string[][])  [unwired: 7 in, 1 out]
            n1874 = local write "LoTable_1"(w2494) -> ()
            n1875 = local read "Limit Cluster"() -> (w2496:T1)
            n1876 = Bundle By Name(cluster=w2496, "Lower Limit"=w2490) -> (w2497:T1)
            n1877 = local write "Limit Cluster"(w2497) -> ()
            n1878 = local write "Plot graphs"(TRUE ("Plot graphs")) -> ()
          }
        }
      }
      event "Delete Upper": Value Change {
        n1879 = event-data() -> ()  [unwired: 7 out]
        n1880 = case shown="True" "Delete Upper" {
          frame False {
          }
          frame True {
            n1881 = property on="UpTable_1" class="Tbl (strict)"() -> ("Value"=w2506:string[][], "Selection Start"=w2504:T5, "Selection Size"=w2505:T5)  [unwired: 2 in, 2 out]
            n1882 = call "CRYLimit Table Delete Item.vi"("Selection Size"=w2505, "Selection Start"=w2504, "Table In"=w2506) -> ("Table Out"=w2502:string[][])  [unwired: 8 out]
            n1883 = local write "UpTable_1"(w2502) -> ()
            n1884 = call "CRYTable Empty Ignore.vi"("Table In"=w2502) -> ("Table Out"=w2503:string[][])  [unwired: 10 in]
            n1885 = call "CRYTable to Curve.vi"("Table In"=w2503) -> ("Limit curve"=w2501:cluster{"Numeric":dbl, "Numeric 2":dbl}[])  [unwired: 10 in]
            n1886 = local read "Limit Cluster"() -> (w2507:T1)
            n1887 = Bundle By Name(cluster=w2507, "Upper Limit"=w2501) -> (w2499:T1)
            n1888 = local write "Plot graphs"(TRUE ("Plot graphs")) -> ()
            n1889 = local write "Limit Cluster"(w2499) -> ()
          }
        }
      }
      event "Delete Lower": Value Change {
        n1890 = event-data() -> ()  [unwired: 7 out]
        n1891 = case shown="True" "Delete Lower" {
          frame False {
          }
          frame True {
            n1892 = property on="LoTable_1" class="Tbl (strict)"() -> ("Value"=w2517:string[][], "Selection Start"=w2515:T5, "Selection Size"=w2516:T5)  [unwired: 2 in, 2 out]
            n1893 = call "CRYLimit Table Delete Item.vi"("Selection Size"=w2516, "Selection Start"=w2515, "Table In"=w2517) -> ("Table Out"=w2511:string[][])  [unwired: 8 out]
            n1894 = call "CRYTable Empty Ignore.vi"("Table In"=w2511) -> ("Table Out"=w2513:string[][])  [unwired: 10 in]
            n1895 = local write "LoTable_1"(w2511) -> ()
            n1896 = call "CRYTable to Curve.vi"("Table In"=w2513) -> ("Limit curve"=w2512:cluster{"Numeric":dbl, "Numeric 2":dbl}[])  [unwired: 10 in]
            n1897 = Delete From Array(array=w2512) -> (array with subset deleted=w2514:cluster{"Numeric":dbl, "Numeric 2":dbl}[])  [unwired: 2 in, 1 out]
            n1898 = local read "Limit Cluster"() -> (w2518:T1)
            n1899 = Bundle By Name(cluster=w2518, "Lower Limit"=w2514) -> (w2509:T1)
            n1900 = local write "Limit Cluster"(w2509) -> ()
            n1901 = local write "Plot graphs"(TRUE ("Plot graphs")) -> ()
          }
        }
      }
      event "Clear Upper": Value Change {
        n1902 = event-data() -> ()  [unwired: 7 out]
        n1903 = case shown="True" "Clear Upper" {
          frame False {
          }
          frame True {
            n1904 = local read "Type"() -> (w2520:u16)
            n1905 = case shown="0, 3" w2520 {
              frame 0, 3 {
                n1906 = local read "Limits_Ring"() -> (w2525:u16)
                n1907 = local write "Up Limit Val"(0.0 ("Up Limit Val")) -> ()
                n1908 = Equal To 0?(x=w2525) -> (x = 0?=w2524:bool)
                n1909 = case shown="True" w2524 {
                  tunnel: 0.0 ("Single Limit") -> [_ w2526]
                  frame False {
                  }
                  frame True {
                    n1910 = local write "Single Limit"(w2526) -> ()
                  }
                }
                n1911 = local write "Plot Multilimit"(TRUE ("Plot Multilimit")) -> ()
              }
              frame 1, 2, Default {
                w2527 = T5 {"Row"=-1, "Column"=-1} ("Selection Start")
                n1912 = local read "Limit Cluster"() -> (w2533:T1)
                n1913 = Bundle By Name(cluster=w2533, "Upper Limit"=cluster{dbl, dbl}[] []) -> (w2531:T1)
                n1914 = local write "Limit Cluster"(w2531) -> ()
                n1915 = property on="UpTable_1" class="Tbl (strict)"("Value"=string[][] [] ("UpTable_1"), "Index Values"=T5 {"Row"=0, "Column"=0} ("Selection Start"), "Selection Start"=w2527, "Selection Size"=w2527) -> ()  [unwired: 2 in, 2 out]
                n1916 = local write "Plot graphs"(TRUE ("Plot graphs")) -> ()
              }
            }
          }
        }
      }
      event "copy Upper": Value Change {
        n1917 = event-data() -> ()  [unwired: 7 out]
        n1918 = case shown="True" "copy Upper" {
          frame False {
          }
          frame True {
            n1919 = local read "Type"() -> (w2535:u16)
            n1920 = case shown="0, 3" w2535 {
              selector: w2535 -> [w2540 _]
              frame 0, 3 {
                n1921 = local read "Limits_Ring"() -> (w2539:u16)
                n1922 = case shown="0, Default" w2540 {
                  tunnel: [w2542 0.0 ("Data Value")] -> w2536
                  frame 0, Default {
                    n1923 = local read "Data Value"() -> (w2542:dbl)
                  }
                  frame 3 {
                  }
                }
                n1924 = local write "Plot Multilimit"(TRUE ("Plot Multilimit")) -> ()
                n1925 = Equal To 0?(x=w2539) -> (x = 0?=w2538:bool)
                n1926 = local write "Up Limit Val"(w2536) -> ()
                n1927 = case shown="True" w2538 {
                  tunnel: w2536 -> [_ w2541]
                  frame False {
                  }
                  frame True {
                    n1928 = local write "Single Limit"(w2541) -> ()
                  }
                }
              }
              frame 1, Default {
                n1929 = local read "Data Table"() -> (w2545:string[][])
                n1930 = global read "CRYLimit edit global.vi" "Data"() -> (w2554:cluster{"x":dbl, "y":dbl}[])
                n1931 = local read "Limit Cluster"() -> (w2555:T1)
                n1932 = Bundle By Name(cluster=w2555, "Upper Limit"=w2554) -> (w2553:T1)
                n1933 = Index Array(array=w2545, index (row)=1) -> (element=w2550:string[])  [unwired: 1 in]
                n1934 = local write "UpTable_1"(w2545) -> ()
                n1935 = Array Size(array=w2550) -> (size(s)=w2549:i32)
                n1936 = Bundle("index (row)"=1, w2549) -> (w2547:cluster{"index (row)":i32, i32})  [unwired: 1 in]
                n1937 = property on="UpTable_1" class="Tbl (strict)"("Selection Size"=w2547, "Selection Start"=T5 {"Row"=1, "Column"=0}, "Index Values"=T8 {"Row"=0, "Column"=0}) -> ()  [unwired: 2 in, 2 out]
                n1938 = local write "Limit Cluster"(w2553) -> ()
                n1939 = local write "Plot graphs"(TRUE ("Plot graphs")) -> ()
              }
            }
          }
        }
      }
      event "Clear Lower": Value Change {
        n1940 = event-data() -> ()  [unwired: 7 out]
        n1941 = case shown="True" "Clear Lower" {
          frame False {
          }
          frame True {
            n1942 = local read "Type"() -> (w2557:u16)
            n1943 = case shown="0, 3" w2557 {
              frame 0, 3 {
                w2558 = 0.0 ("Lo Limit Val")
                n1944 = local read "Limits_Ring"() -> (w2562:u16)
                n1945 = Equal?(x=w2562, y=u16 1) -> (x = y?=w2560:bool)
                n1946 = local write "Lo Limit Val"(w2558) -> ()
                n1947 = case shown="True" w2560 {
                  tunnel: w2558 -> [_ w2563]
                  frame False {
                  }
                  frame True {
                    n1948 = local write "Single Limit"(w2563) -> ()
                  }
                }
                n1949 = local write "Plot Multilimit"(TRUE ("Plot Multilimit")) -> ()
              }
              frame 1, 2, Default {
                n1950 = local read "Limit Cluster"() -> (w2566:T1)
                n1951 = Bundle By Name(cluster=w2566, "Lower Limit"=cluster{dbl, dbl}[] []) -> (w2564:T1)
                n1952 = local write "Limit Cluster"(w2564) -> ()
                n1953 = flat-sequence {
                  frame #0 {
                    w2567 = T5 {"Row"=-1, "Column"=-1} ("Selection Size")
                    n1954 = property on="LoTable_1" class="Tbl (strict)"("Value"=string[][] [] ("LoTable_1"), "Index Values"=T5 {"Row"=0, "Column"=0} ("Selection Start"), "Selection Start"=w2567, "Selection Size"=w2567) -> ()  [unwired: 2 in, 2 out]
                  }
                  frame #1 {
                    n1955 = local write "Plot graphs"(TRUE ("Plot graphs")) -> ()
                  }
                }
              }
            }
          }
        }
      }
      event "copy Lower": Value Change {
        n1956 = event-data() -> ()  [unwired: 7 out]
        n1957 = case shown="True" "copy Lower" {
          frame False {
          }
          frame True {
            n1958 = local read "Type"() -> (w2572:u16)
            n1959 = case shown="0, 3" w2572 {
              selector: w2572 -> [w2578 _]
              frame 0, 3 {
                n1960 = local read "Limits_Ring"() -> (w2576:u16)
                n1961 = case shown="0, Default" w2578 {
                  tunnel: [w2580 0.0 ("Data Value")] -> w2573
                  frame 0, Default {
                    n1962 = local read "Data Value"() -> (w2580:dbl)
                  }
                  frame 3 {
                  }
                }
                n1963 = local write "Plot Multilimit"(TRUE ("Plot Multilimit")) -> ()
                n1964 = Equal?(x=w2576, y=u16 1) -> (x = y?=w2575:bool)
                n1965 = case shown="True" w2575 {
                  tunnel: w2573 -> [_ w2579]
                  frame False {
                  }
                  frame True {
                    n1966 = local write "Single Limit"(w2579) -> ()
                  }
                }
                n1967 = local write "Lo Limit Val"(w2573) -> ()
              }
              frame 1, Default {
                n1968 = local read "Data Table"() -> (w2586:string[][])
                n1969 = global read "CRYLimit edit global.vi" "Data"() -> (w2592:cluster{"x":dbl, "y":dbl}[])
                n1970 = local read "Limit Cluster"() -> (w2593:T1)
                n1971 = local write "Plot graphs"(TRUE ("Plot graphs")) -> ()
                n1972 = Bundle By Name(cluster=w2593, "Lower Limit"=w2592) -> (w2591:T1)
                n1973 = Index Array(array=w2586, index (row)=1) -> (element=w2589:string[])  [unwired: 1 in]
                n1974 = local write "LoTable_1"(w2586) -> ()
                n1975 = Array Size(array=w2589) -> (size(s)=w2588:i32)
                n1976 = local write "Limit Cluster"(w2591) -> ()
                n1977 = Bundle("index (row)"=1, w2588) -> (w2584:cluster{"index (row)":i32, i32})  [unwired: 1 in]
                n1978 = property on="LoTable_1" class="Tbl (strict)"("Selection Size"=w2584, "Selection Start"=T5 {"Row"=1, "Column"=0}, "Index Values"=T8 {"Row"=0, "Column"=0}) -> ()  [unwired: 2 in, 2 out]
              }
            }
          }
        }
      }
      event "Multi Limit": Value Change {
        n1979 = event-data() -> ("CtlRef"=w2602:refnum<vi>)  [unwired: 6 out]
        n1980 = local read "Limits_Ring"() -> (w2600:u16)
        n1981 = local read "LoSource"() -> (w2598:u16)
        n1982 = local read "UpSource"() -> (w2599:u16)
        n1983 = Equal To 0?(x=w2598) -> (x = 0?=w2595:bool)
        n1984 = Equal?(x=w2600, y=u16 2) -> (x = y?=w2597:bool)
        n1985 = Equal To 0?(x=w2599) -> (x = 0?=w2596:bool)
        n1986 = Compound Arithmetic op=AND(w2597, w2596, w2595) -> (w2594:bool)
        n1987 = case shown="True" w2594 {
          tunnel: w2602 -> [_ w2627]
          tunnel: w2600 -> [_ w2626]
          frame False {
          }
          frame True {
            w2624 = 0 ("index")
            n1988 = control-ref of="Multi value"() -> (w2625:refnum<vi>)
            n1989 = call "CRYMultilimit Value Change.vi"("Limits"=w2626, "Multi Limit"=w2627, "Multi value"=w2625) -> ("Lo tip"=w2612:cluster{dbl, dbl}, "Up tip"=w2613:cluster{dbl, dbl}, "Lower Limit"=w2607:dbl, "Upper Limit"=w2609:dbl)  [unwired: 3 in, 2 out]
            n1990 = local read "Limit Cluster"() -> (w2611:T1)
            n1991 = property on="Up tip" class="Str"("Position"=w2613) -> ()  [unwired: 2 in, 2 out]
            n1992 = property on="Lo tip" class="Str"("Position"=w2612) -> ()  [unwired: 2 in, 2 out]
            n1993 = local read "Y Resolution"() -> (w2608:u8)
            n1994 = Unbundle By Name(w2611) -> ("Upper Limit"=w2619:cluster{dbl, dbl}[], "Lower Limit"=w2614:cluster{dbl, dbl}[])
            n1995 = local write "RawLo Limit"(w2607) -> ()
            n1996 = local write "RawUp Limit"(w2609) -> ()
            n1997 = call "CRYRepresent numeric by precission.vi"("Pprecision"=w2608, "Numeric In"=w2607) -> ("Out Format"=w2603:string, "Numeric Out"=w2604:dbl)  [unwired: 7 in, 1 out]
            n1998 = call "CRYRepresent numeric by precission.vi"("Pprecision"=w2608, "Numeric In"=w2609) -> ("Out Format"=w2605:string, "Numeric Out"=w2606:dbl)  [unwired: 7 in, 1 out]
            n1999 = Index Array(array=w2619, index=w2624) -> (element=w2623:cluster{dbl, dbl})
            n2000 = Index Array(array=w2614, index=w2624) -> (element=w2622:cluster{dbl, dbl})
            n2001 = property on="Up Limit Val" class="DigNum (strict)"("Value"=w2606, "FormatString"=w2605) -> ()  [unwired: 2 in, 2 out]
            n2002 = property on="Lo Limit Val" class="DigNum (strict)"("Value"=w2604, "FormatString"=w2603) -> ()  [unwired: 2 in, 2 out]
            n2003 = Unbundle(w2622) -> (w2617:dbl)  [unwired: 1 out]
            n2004 = Unbundle(w2623) -> (w2621:dbl)  [unwired: 1 out]
            n2005 = Bundle(w2621, "Upper Limit"=w2609) -> (w2620:cluster{dbl, "Upper Limit":dbl})  [unwired: 1 out]
            n2006 = Bundle(w2617, "Lower Limit"=w2607) -> (w2616:cluster{dbl, "Lower Limit ":dbl})  [unwired: 1 out]
            n2007 = Replace Array Subset(array=w2619, new element=w2620, index=0) -> (w2629:cluster{dbl, dbl}[])
            n2008 = Replace Array Subset(array=w2614, new element=w2616, index=0) -> (w2628:cluster{dbl, dbl}[])
            n2009 = Bundle By Name(cluster=w2611, "Upper Limit"=w2629, "Lower Limit"=w2628) -> (w2610:T1)
            n2010 = local write "Limit Cluster"(w2610) -> ()
          }
        }
      }
      event "Up Limit Val": Value Change {
        n2011 = event-data() -> ("NewVal"=w2632:dbl)  [unwired: 6 out]
        n2012 = local read "Limit Cluster"() -> (w2644:T1)
        n2013 = Unbundle By Name(w2644) -> ("Upper Limit"=w2635:cluster{dbl, dbl}[])
        n2014 = Array Size(array=w2635) -> (size(s)=w2638:i32)
        n2015 = Equal To 0?(x=w2638) -> (x = 0?=w2637:bool)
        n2016 = local read "Y Resolution"() -> (w2630:u8)
        n2017 = local write "RawUp Limit"(w2632) -> ()
        n2018 = Select(t=cluster{dbl, dbl}[] [{0.0, 0.0}] ("Upper Limit"), s=w2637, f=w2635) -> (s? t:f=w2634:cluster{dbl, dbl}[])
        n2019 = call "CRYRepresent numeric by precission.vi"("Pprecision"=w2630, "Numeric In"=w2632) -> ("Out Format"=w2633:string, "Numeric Out"=w2631:dbl)  [unwired: 7 in, 1 out]
        n2020 = property on="Up Limit Val" class="DigNum (strict)"("Value"=w2631, "FormatString"=w2633) -> ()  [unwired: 2 in, 2 out]
        n2021 = local read "Limits_Ring"() -> (w2642:u16)
        n2022 = Index Array(array=w2634, index=0) -> (element=w2648:cluster{dbl, dbl})
        n2023 = Equal To 0?(x=w2642) -> (x = 0?=w2641:bool)
        n2024 = Unbundle(w2648) -> (w2647:dbl)  [unwired: 1 out]
        n2025 = Bundle(w2647, "Numeric Out"=w2631) -> (w2646:cluster{dbl, "Numeric Out":dbl})  [unwired: 1 out]
        n2026 = case shown="True" w2641 {
          tunnel: w2631 -> [_ w2650]
          frame False {
          }
          frame True {
            n2027 = local write "Single Limit"(w2650) -> ()
          }
        }
        n2028 = Replace Array Subset(array=w2634, new element=w2646, index=0) -> (w2643:cluster{dbl, dbl}[])
        n2029 = Bundle By Name(cluster=w2644, "Upper Limit"=w2643, "Up Limit Val"=w2631) -> (w2639:T1)
        n2030 = local write "Limit Cluster"(w2639) -> ()
        n2031 = local write "Plot Multilimit"(TRUE ("Plot Multilimit")) -> ()
      }
      event "Lo Limit Val": Value Change {
        n2032 = event-data() -> ("NewVal"=w2653:dbl)  [unwired: 6 out]
        n2033 = local read "Limit Cluster"() -> (w2666:T1)
        n2034 = Unbundle By Name(w2666) -> ("Lower Limit"=w2656:cluster{dbl, dbl}[])
        n2035 = Array Size(array=w2656) -> (size(s)=w2659:i32)
        n2036 = Equal To 0?(x=w2659) -> (x = 0?=w2658:bool)
        n2037 = Select(t=cluster{dbl, dbl}[] [{0.0, 0.0}] ("Upper Limit"), s=w2658, f=w2656) -> (s? t:f=w2655:cluster{dbl, dbl}[])
        n2038 = local read "Limits_Ring"() -> (w2664:u16)
        n2039 = local read "Y Resolution"() -> (w2651:u8)
        n2040 = local write "RawLo Limit"(w2653) -> ()
        n2041 = Index Array(array=w2655, index=0) -> (element=w2668:cluster{dbl, dbl})
        n2042 = Equal?(x=w2664, y=u16 1) -> (x = y?=w2662:bool)
        n2043 = Unbundle(w2668) -> (w2669:dbl)  [unwired: 1 out]
        n2044 = call "CRYRepresent numeric by precission.vi"("Pprecision"=w2651, "Numeric In"=w2653) -> ("Out Format"=w2654:string, "Numeric Out"=w2652:dbl)  [unwired: 7 in, 1 out]
        n2045 = property on="Lo Limit Val" class="DigNum (strict)"("Value"=w2652, "FormatString"=w2654) -> ()  [unwired: 2 in, 2 out]
        n2046 = Bundle(w2669, "Numeric Out"=w2652) -> (w2670:cluster{dbl, "Numeric Out":dbl})  [unwired: 1 out]
        n2047 = case shown="True" w2662 {
          tunnel: w2652 -> [_ w2672]
          frame False {
          }
          frame True {
            n2048 = local write "Single Limit"(w2672) -> ()
          }
        }
        n2049 = Replace Array Subset(array=w2655, new element=w2670, index=0) -> (w2665:cluster{dbl, dbl}[])
        n2050 = Bundle By Name(cluster=w2666, "Lower Limit"=w2665, "Low Limit Val"=w2652) -> (w2660:T1)
        n2051 = local write "Plot Multilimit"(TRUE ("Plot Multilimit")) -> ()
        n2052 = local write "Limit Cluster"(w2660) -> ()
      }
      event "Single Limit": Value Change {
        n2053 = event-data() -> ("NewVal"=w2674:dbl)  [unwired: 6 out]
        n2054 = local read "Limits_Ring"() -> (w2675:u16)
        n2055 = local read "Limit Cluster"() -> (w2673:T1)
        n2056 = Not Equal?(x=w2675, y=u16 2) -> (x != y?=w2677:bool)
        n2057 = case shown="True" w2677 {
          tunnel: w2675 -> [_ w2680]
          tunnel: w2674 -> [_ w2679]
          tunnel: w2673 -> [_ w2678]
          frame False {
          }
          frame True {
            n2058 = case shown="0, Default" w2680 {
              tunnel: w2679 -> [w2684 w2702]
              tunnel: w2678 -> [w2681 w2699]
              frame 0, Default {
                n2059 = local read "UpSource"() -> (w2682:u16)
                n2060 = Equal To 0?(x=w2682) -> (x = 0?=w2683:bool)
                n2061 = case shown="True" w2683 {
                  tunnel: w2684 -> [_ w2686]
                  tunnel: w2681 -> [_ w2691]
                  frame False {
                  }
                  frame True {
                    n2062 = Unbundle By Name(w2691) -> ("Upper Limit"=w2693:cluster{dbl, dbl}[])
                    n2063 = Index Array(array=w2693, index=0) -> (element=w2697:cluster{dbl, dbl})
                    n2064 = Unbundle(w2697) -> (w2696:dbl)  [unwired: 1 out]
                    n2065 = local write "Plot Multilimit"(TRUE ("Plot Multilimit")) -> ()
                    n2066 = Bundle(w2696, "NewVal"=w2686) -> (w2695:cluster{dbl, "NewVal":dbl})  [unwired: 1 out]
                    n2067 = Replace Array Subset(array=w2693, new element=w2695, index=0) -> (w2692:cluster{dbl, dbl}[])
                    n2068 = local read "Y Resolution"() -> (w2687:u8)
                    n2069 = Bundle By Name(cluster=w2691, "Upper Limit"=w2692) -> (w2689:T1)
                    n2070 = local write "RawUp Limit"(w2686) -> ()
                    n2071 = call "CRYRepresent numeric by precission.vi"("Pprecision"=w2687, "Numeric In"=w2686) -> ("Out Format"=w2688:string, "Numeric Out"=w2685:dbl)  [unwired: 7 in, 1 out]
                    n2072 = property on="Up Limit Val" class="DigNum (strict)"("Value"=w2685, "FormatString"=w2688) -> ()  [unwired: 2 in, 2 out]
                    n2073 = local write "Limit Cluster"(w2689) -> ()
                  }
                }
              }
              frame 1 {
                n2074 = local read "LoSource"() -> (w2700:u16)
                n2075 = Equal To 0?(x=w2700) -> (x = 0?=w2701:bool)
                n2076 = case shown="True" w2701 {
                  tunnel: w2702 -> [_ w2703]
                  tunnel: w2699 -> [_ w2709]
                  frame False {
                  }
                  frame True {
                    n2077 = Unbundle By Name(w2709) -> ("Lower Limit"=w2711:cluster{dbl, dbl}[])
                    n2078 = Index Array(array=w2711, index=0) -> (element=w2713:cluster{dbl, dbl})
                    n2079 = Unbundle(w2713) -> (w2714:dbl)  [unwired: 1 out]
                    n2080 = local write "Plot Multilimit"(TRUE ("Plot Multilimit")) -> ()
                    n2081 = Bundle(w2714, "NewVal"=w2703) -> (w2715:cluster{dbl, "NewVal":dbl})  [unwired: 1 out]
                    n2082 = Replace Array Subset(array=w2711, new element=w2715, index=0) -> (w2710:cluster{dbl, dbl}[])
                    n2083 = Bundle By Name(cluster=w2709, "Lower Limit"=w2710) -> (w2707:T1)
                    n2084 = local write "RawLo Limit"(w2703) -> ()
                    n2085 = local read "Y Resolution"() -> (w2706:u8)
                    n2086 = disable-structure shown="Disabled" {
                      frame Disabled {
                      }
                      frame Enabled {
                      }
                    }
                    n2087 = call "CRYRepresent numeric by precission.vi"("Pprecision"=w2706, "Numeric In"=w2703) -> ("Out Format"=w2704:string, "Numeric Out"=w2705:dbl)  [unwired: 7 in, 1 out]
                    n2088 = property on="Lo Limit Val" class="DigNum (strict)"("Value"=w2705, "FormatString"=w2704) -> ()  [unwired: 2 in, 2 out]
                    n2089 = local write "Limit Cluster"(w2707) -> ()
                  }
                }
              }
            }
          }
        }
      }
      event "Step Size", "Maximum", "Minimum": Value Change {
        n2090 = event-data() -> ()  [unwired: 7 out]
        n2091 = local read "Limit Cluster"() -> (w2726:T1)
        n2092 = local read "Minimum"() -> (w2723:dbl)
        n2093 = local read "Mapping"() -> (w2724:u16)
        n2094 = local read "Maximum"() -> (w2722:dbl)
        n2095 = local read "Step Size"() -> (w2721:dbl)
        n2096 = case shown="1, Default" w2724 {
          tunnel: w2723 -> [w2730 w2741]
          tunnel: [w2730 w2739] -> w2720
          tunnel: w2721 -> [w2728 w2736]
          tunnel: [w2729 w2733] -> w2719
          tunnel: [w2728 w2732] -> w2718
          tunnel: w2722 -> [w2729 w2731]
          frame 0 {
          }
          frame 1, Default {
            w2735 = 100.0
            w2734 = 1.0
            n2097 = Divide(x=w2741, y=w2735) -> (x/y=w2740:dbl)
            n2098 = Divide(x=w2731, y=w2735) -> (x/y=w2738:dbl)
            n2099 = Divide(x=w2736, y=w2735) -> (x/y=w2737:dbl)
            n2100 = Add(x=w2734, y=w2740) -> (x+y=w2739:dbl)
            n2101 = Add(x=w2734, y=w2738) -> (x+y=w2733:dbl)
            n2102 = Add(x=w2734, y=w2737) -> (x+y=w2732:dbl)
          }
        }
        n2103 = Unbundle By Name(w2726) -> ("X min-max-step"=w2727:T15)
        n2104 = Bundle By Name(cluster=w2727, "Limit X Offset Min"=w2720, "Limit X Offset Max"=w2719, "Limit X Offset Step Size"=w2718) -> (w2725:T15)
        n2105 = Bundle By Name(cluster=w2726, "X min-max-step"=w2725) -> (w2717:T1)
        n2106 = local write "Limit Cluster"(w2717) -> ()
      }
      event "X AlignRef", "Y AlignRef": Value Change {
        n2107 = event-data() -> ()  [unwired: 7 out]
        n2108 = local read "Y AlignRef"() -> (w2745:dbl)
        n2109 = local read "X AlignRef"() -> (w2746:dbl)
        n2110 = Bundle("X AlignRef"=w2746, "Y AlignRef"=w2745) -> (w2743:cluster{"X AlignRef":dbl, "Y AlignRef":dbl})  [unwired: 1 out]
        n2111 = local read "Limit Cluster"() -> (w2744:T1)
        n2112 = Bundle By Name(cluster=w2744, "Align Ref"=w2743) -> (w2742:T1)
        n2113 = local write "Limit Cluster"(w2742) -> ()
      }
      event "Help": Value Change {
        n2114 = event-data() -> ("NewVal"=w2748:string)  [unwired: 6 out]
        n2115 = local read "Limit Cluster"() -> (w2749:T1)
        n2116 = Bundle By Name(cluster=w2749, "Help"=w2748) -> (w2747:T1)
        n2117 = local write "Limit Cluster"(w2747) -> ()
      }
      event "Custom Name": Value Change {
        n2118 = event-data() -> ("NewVal"=w2750:string)  [unwired: 6 out]
        n2119 = local read "Limit Cluster"() -> (w2752:T1)
        n2120 = Bundle By Name(cluster=w2752, "Custom Name"=w2750) -> (w2751:T1)
        n2121 = local write "Limit Cluster"(w2751) -> ()
      }
      event "bAdd DataName": Value Change {
        n2122 = event-data() -> ("NewVal"=w2753:bool)  [unwired: 6 out]
        n2123 = local read "Limit Cluster"() -> (w2755:T1)
        n2124 = Bundle By Name(cluster=w2755, "bAdd DataName"=w2753) -> (w2754:T1)
        n2125 = local write "Limit Cluster"(w2754) -> ()
      }
    }
    n2126 = Bundle("Appy limits"="Appy limits", "Load Test"="Load Test", "Plot graphs"="Plot graphs", "Plot Multilimit"="Plot Multilimit", "Add Lib"="Add Lib", "OK"="OK", "Cancel"="Cancel") -> (w85:T16)  [unwired: 1 out]
    n2127 = Cluster To Array(cluster=w85) -> (array=w84:bool[])
    n2128 = Search 1D Array(1D array=w84, element=TRUE) -> (index of element=w82:i32)  [unwired: 1 out]
    n2129 = case shown="5" w82 {
      frame Default {
      }
      frame 0 {
        n2130 = global read "CRYMainGlobal.vi" "Access Level"() -> (w2756:enum16{"Engineer", "Technician", "Operator"})
        n2131 = case shown="\"Operator\", Default" w2756 {
          frame "Engineer" {
            n2132 = flat-sequence {
              tunnel: [w2762] -> w2761
              tunnel: [w2773] -> w2760
              tunnel: w2761 -> [w2773]
              tunnel: [w2772] -> w2759
              tunnel: [w2768] -> w2758
              tunnel: [w2767] -> w2757
              tunnel: w2760 -> [w2780]
              tunnel: w2759 -> [w2779]
              tunnel: w2758 -> [w2778]
              tunnel: w2757 -> [w2777]
              frame #0 {
                n2133 = call "CRYGet Current TS Steps.vi"() -> ("SelectStepNumber in Tree"=w2764:i32, "Steps"=w2763:T7[])  [unwired: 1 in, 9 out]
                n2134 = Index Array(array=w2763, index=w2764) -> (element=w2762:T7)
              }
              frame #1 {
                w2765 = FALSE ("Visible")
                n2135 = local read "Limit Cluster"() -> (w2774:T1)
                n2136 = local read "Proper VI No"() -> (w2771:i32)
                n2137 = property on="Margin" class="DigNum (strict)"("Visible"=w2765) -> ()  [unwired: 2 in, 2 out]
                n2138 = property on="Verdict" class="Bool (strict)"("Visible"=w2765) -> ()  [unwired: 2 in, 2 out]
                n2139 = property on="tolerance" class="Str"("Visible"=w2765) -> ()  [unwired: 2 in, 2 out]
                n2140 = global write "CRYLimit edit global.vi" "ContinueF"(TRUE ("ContinueF")) -> ()
                n2141 = call "CRYFlatten Limits.vi"("Limits"=w2774) -> ("Flatten Limits String"=w2772:string)  [unwired: 10 out]
                n2142 = Build Array(w2771) -> (w2769:i32[])
                n2143 = call "CRYGet Curve Library Data Name.vi"("nData"=w2769, "sAction"="GetNamebyStep" ("sOption")) -> ("sNames"=w2768:string[], "Type Out"=w2767:string[])  [unwired: 6 in, 2 out]
              }
              frame #2 {
                w2787 = enum32{"Single Values", "Curves", "Waveforms"}."Waveforms" ("y")
                n2144 = local read "Lo_type"() -> (w2788:enum32{"Single Values", "Curves", "Waveforms"})
                n2145 = local read "Up_type"() -> (w2789:enum32{"Single Values", "Curves", "Waveforms"})
                n2146 = local read "Type"() -> (w2783:u16)
                n2147 = Not Equal?(x=w2789, y=w2787) -> (x != y?=w2786:bool)
                n2148 = Not Equal?(x=w2787, y=w2788) -> (x != y?=w2785:bool)
                n2149 = And(x=w2786, y=w2785) -> (x .and. y?=w2784:bool)
                n2150 = Bundle By Name(cluster=w2780, "Seq setup flattened"=w2779) -> (w2776:T7)
                n2151 = Unbundle By Name(w2776) -> ("StepName"=w2775:string)
                n2152 = local read "Limits_Ring"() -> (w2781:u16)
                n2153 = case shown="True" w2784 {
                  selector: w2784 -> [w2790 _]
                  tunnel: [w2790 w2801] -> w2782
                  tunnel: w2783 -> [_ w2796]
                  tunnel: w2781 -> [_ w2793]
                  frame False {
                  }
                  frame True {
                    n2154 = local read "UpSource"() -> (w2792:u16)
                    n2155 = local read "LoSource"() -> (w2791:u16)
                    n2156 = Not Equal To 0?(x=w2796) -> (x != 0?=w2797:bool)
                    n2157 = case shown="False" w2797 {
                      tunnel: [w2806 w2819] -> w2795
                      tunnel: [w2804 w2818] -> w2794
                      tunnel: w2792 -> [w2803 w2822]
                      tunnel: w2791 -> [w2802 w2821]
                      frame False {
                        w2808 = 0.0 ("UpSingleVal")
                        n2158 = case shown="0, Default" w2803 {
                          tunnel: [w2813 w2814] -> w2810
                          frame 0, Default {
                            n2159 = local read "Up Limit Val"() -> (w2813:dbl)
                          }
                          frame 1 {
                            n2160 = local read "UpSingleVal"() -> (w2814:dbl)
                          }
                        }
                        n2161 = case shown="0, Default" w2802 {
                          tunnel: [w2811 w2812] -> w2809
                          frame 0, Default {
                            n2162 = local read "Lo Limit Val"() -> (w2811:dbl)
                          }
                          frame 1 {
                            n2163 = local read "LoSingleVal"() -> (w2812:dbl)
                          }
                        }
                        n2164 = Bundle("UpSingleVal"=w2808, "UpSingleVal"=w2810) -> (w2807:cluster{"UpSingleVal":dbl, "UpSingleVal":dbl})  [unwired: 1 out]
                        n2165 = Bundle("UpSingleVal"=w2808, "LoSingleVal"=w2809) -> (w2805:cluster{"UpSingleVal":dbl, "LoSingleVal":dbl})  [unwired: 1 out]
                        n2166 = Build Array(w2807) -> (w2806:cluster{"UpSingleVal":dbl, "UpSingleVal":dbl}[])
                        n2167 = Build Array(w2805) -> (w2804:cluster{"UpSingleVal":dbl, "LoSingleVal":dbl}[])
                      }
                      frame True {
                        n2168 = case shown="0, Default" w2822 {
                          tunnel: [w2825 w2826] -> w2820
                          frame 0, Default {
                            n2169 = local read "UpTable_1"() -> (w2825:string[][])
                          }
                          frame 1 {
                            n2170 = local read "UpTable_2"() -> (w2826:string[][])
                          }
                        }
                        n2171 = case shown="0, Default" w2821 {
                          tunnel: [w2823 w2824] -> w2816
                          frame 0, Default {
                            n2172 = local read "LoTable_1"() -> (w2823:string[][])
                          }
                          frame 1 {
                            n2173 = local read "LoTable_2"() -> (w2824:string[][])
                          }
                        }
                        n2174 = call "CRYTable Empty Ignore.vi"("Table In"=w2820) -> ("Table Out"=w2817:string[][])  [unwired: 10 in]
                        n2175 = call "CRYTable Empty Ignore.vi"("Table In"=w2816) -> ("Table Out"=w2815:string[][])  [unwired: 10 in]
                        n2176 = call "CRYTable to Curve.vi"("Table In"=w2817) -> ("Limit curve"=w2819:cluster{"Numeric":dbl, "Numeric 2":dbl}[])  [unwired: 10 in]
                        n2177 = call "CRYTable to Curve.vi"("Table In"=w2815) -> ("Limit curve"=w2818:cluster{"Numeric":dbl, "Numeric 2":dbl}[])  [unwired: 10 in]
                      }
                    }
                    n2178 = local read "data unit"() -> (w2800:string)
                    n2179 = local read "up_unit"() -> (w2799:string)
                    n2180 = local read "low_unit"() -> (w2798:string)
                    n2181 = call "CRYSUpper_Lowerness Check.vi"("Limits"=w2793, "Lo unit"=w2798, "Data unit"=w2800, "Up unit"=w2799, "Type"=w2796, "Lo source"=w2791, "Up source"=w2792, "Lower limit"=w2794, "Upper limit"=w2795) -> ("Do save"=w2801:bool)  [unwired: 2 out]
                  }
                }
                n2182 = case shown="True" w2782 {
                  tunnel: w2776 -> [_ w2840]
                  tunnel: w2783 -> [_ w2839]
                  tunnel: w2775 -> [_ w2838]
                  tunnel: w2781 -> [_ w2837]
                  tunnel: w2778 -> [_ w2834]
                  tunnel: w2777 -> [_ w2833]
                  frame False {
                    n2183 = call "CRYGet Error Message.vi"("Error No"=1, "Kind"="Limits") -> ("Message"=w2829:string, "Window Title"=w2828:string)  [unwired: 4 in, 4 out]
                    n2184 = call "CRYMessage Dialog.vi"("Window Title"=w2828, "YesNoCancel"=T9."OK", "Message Content"=w2829) -> ()  [unwired: 7 in, 2 out]
                  }
                  frame True {
                    n2185 = flat-sequence {
                      tunnel: w2840 -> [w2849]
                      tunnel: w2839 -> [w2863]
                      tunnel: w2838 -> [w2859]
                      tunnel: w2837 -> [w2858]
                      tunnel: [w2843] -> w2836
                      tunnel: [w2848] -> w2835
                      tunnel: w2834 -> [w2848]
                      tunnel: w2833 -> [w2844]
                      tunnel: [w2844] -> w2832
                      tunnel: w2836 -> [w3072]
                      tunnel: w2835 -> [w3071]
                      tunnel: w2832 -> [w3069]
                      frame #0 {
                        n2186 = call "CRYLimits.vi"("Setup in"=w2849, "Step Name"=w2859) -> ("Inserted Names Out"=w2843:string[], "Data Out"=w2842:T13, "Results Out"=w2847:T17[], "Waveforms Out"=w2864:T2[])  [unwired: 6 in, 4 out]
                        n2187 = local read "Alignment"() -> (w2852:u16)
                        n2188 = local read "X Resolution"() -> (w2865:u8)
                        n2189 = local read "Y Resolution"() -> (w2857:u8)
                        n2190 = local read "UpSource"() -> (w2862:u16)
                        n2191 = local read "LoSource"() -> (w2861:u16)
                        n2192 = Index Array(array=w2847, index=0) -> (element=w2860:T17)
                        n2193 = case shown="0, Default" w2863 {
                          tunnel: [u16 8 ("Type") u16 7 ("Type")] -> w2855
                          frame 0, Default {
                          }
                          frame 1, 2 {
                          }
                        }
                        n2194 = case shown="1" w2863 {
                          tunnel: w2858 -> [_ w2883 w2986]
                          tunnel: w2865 -> [_ w2882 w2991]
                          tunnel: w2857 -> [_ w2881 w2990]
                          tunnel: w2864 -> [_ _ w2987]
                          tunnel: w2842 -> [_ w2878 w2984]
                          tunnel: w2862 -> [_ w2880 w2989]
                          tunnel: w2861 -> [_ w2879 w2988]
                          tunnel: w2852 -> [_ w2877 w2985]
                          frame 0, Default {
                            n2195 = local write "Plot Multilimit"(TRUE ("Plot Multilimit")) -> ()
                          }
                          frame 1 {
                            n2196 = flat-sequence {
                              tunnel: w2883 -> [w2905]
                              tunnel: w2882 -> [w2891]
                              tunnel: w2881 -> [w2892]
                              tunnel: w2880 -> [w2904]
                              tunnel: w2879 -> [w2903]
                              tunnel: w2878 -> [w2885]
                              tunnel: w2877 -> [w2899]
                              frame #0 {
                                n2197 = local read "Curve and Value"() -> (w2887:T3)
                                n2198 = local read "Data_xyz"() -> (w2888:u16)
                                n2199 = Equal?(x=w2899, y=u16 3) -> (x = y?=w2896:bool)
                                n2200 = Equal?(x=w2899, y=u16 5) -> (x = y?=w2897:bool)
                                n2201 = Or(x=w2896, y=w2897) -> (x .or. y?=w2889:bool)
                                n2202 = Select(t=u16 2 ("y"), s=w2889, f=u16 1 ("y")) -> (s? t:f=w2893:u16)
                                n2203 = case shown="True" w2889 {
                                tunnel: w2885 -> [_ w2927]
                                tunnel: [w2906 w2924] -> w2886
                                tunnel: w2888 -> [w2907 _]
                                tunnel: w2887 -> [w2909 _]
                                frame False {
                                n2204 = Unbundle By Name(w2909) -> ("Curve"=w2908:cluster{"x":dbl, "y":dbl, "z":dbl}[])
                                n2205 = for {
                                tunnel: w2908 -> [w2911] mode=indexing
                                tunnel: w2907 -> [w2912]
                                tunnel: [w2910] -> w2906 mode=indexing
                                n2206 = case shown="2" w2912 {
                                tunnel: w2911 -> [w2915 w2919 w2923]
                                tunnel: [w2913 w2916 w2920] -> w2910
                                frame 0, Default {
                                n2207 = Unbundle(w2915) -> ("x"=w2914:dbl)  [unwired: 2 out]
                                n2208 = Bundle("x"=w2914, "x"=w2914) -> (w2913:cluster{"x":dbl, "x":dbl})  [unwired: 1 in]
                                }
                                frame 1 {
                                n2209 = Unbundle(w2919) -> ("x"=w2918:dbl, "y"=w2917:dbl)  [unwired: 1 out]
                                n2210 = Bundle("x"=w2918, "y"=w2917) -> (w2916:cluster{"x":dbl, "y":dbl})  [unwired: 1 in]
                                }
                                frame 2 {
                                n2211 = Unbundle(w2923) -> ("x"=w2922:dbl, "z"=w2921:dbl)  [unwired: 1 out]
                                n2212 = Bundle("x"=w2922, "z"=w2921) -> (w2920:cluster{"x":dbl, "z":dbl})  [unwired: 1 in]
                                }
                                }
                                }
                                }
                                frame True {
                                n2213 = Index Array(array=w2927, index=1) -> (element=w2925:T3)
                                n2214 = call "CRYDAT to Limit Curve.vi"("Data In"=w2925) -> ("Curve Out"=w2924:cluster{"x":dbl, "y":dbl}[])  [unwired: 10 out]
                                }
                                }
                                n2215 = Array Size(array=w2885) -> (size(s)=w2902:i32)
                                n2216 = Equal To 0?(x=w2902) -> (x = 0?=w2901:bool)
                                n2217 = case shown="False" w2901 {
                                tunnel: w2905 -> [w2934 _]
                                tunnel: w2885 -> [w2931 _]
                                tunnel: w2891 -> [w2933 _]
                                tunnel: w2892 -> [w2932 _]
                                tunnel: w2904 -> [w2930 _]
                                tunnel: w2903 -> [w2929 _]
                                tunnel: w2893 -> [w2928 _]
                                frame False {
                                n2218 = case shown="2, Default" w2934 {
                                tunnel: w2931 -> [w2947 w2961 w2977]
                                tunnel: w2933 -> [w2946 w2965 w2976]
                                tunnel: w2932 -> [w2945 w2964 w2975]
                                tunnel: w2930 -> [w2941 w2962 _]
                                tunnel: w2929 -> [w2940 _ w2973]
                                tunnel: w2928 -> [w2938 _ _]
                                frame 2, Default {
                                n2219 = Index Array(array=w2947, index=w2938) -> (element=w2935:T3)
                                n2220 = Index Array(array=w2947, index=0) -> (element=w2939:T3)
                                n2221 = call "CRYDAT to Limit Curve.vi"("Data In"=w2935) -> ("Curve Out"=w2936:cluster{"x":dbl, "y":dbl}[])  [unwired: 10 out]
                                n2222 = call "CRYDAT to Limit Curve.vi"("Data In"=w2939) -> ("Curve Out"=w2937:cluster{"x":dbl, "y":dbl}[])  [unwired: 10 out]
                                n2223 = call "CRYCurve to Table.vi"("y precision"=w2945, "x precision"=w2946, "Limit curve In"=w2937) -> ("Limit Table"=w2943:string[][])  [unwired: 1 in, 7 out]
                                n2224 = call "CRYCurve to Table.vi"("y precision"=w2945, "x precision"=w2946, "Limit curve In"=w2936) -> ("Limit Table"=w2942:string[][])  [unwired: 1 in, 7 out]
                                n2225 = case shown="0, Default" w2941 {
                                tunnel: w2943 -> [w2956 w2957]
                                tunnel: w2937 -> [w2953 _]
                                frame 0, Default {
                                n2226 = local write "UpTable_1"(w2956) -> ()
                                n2227 = local read "Limit Cluster"() -> (w2954:T1)
                                n2228 = Bundle By Name(cluster=w2954, "Upper Limit"=w2953) -> (w2955:T1)
                                n2229 = local write "Limit Cluster"(w2955) -> ()
                                }
                                frame 1 {
                                n2230 = local write "UpTable_2"(w2957) -> ()
                                }
                                }
                                n2231 = case shown="0, Default" w2940 {
                                tunnel: w2942 -> [w2951 w2952]
                                tunnel: w2936 -> [w2948 _]
                                frame 0, Default {
                                n2232 = local write "LoTable_1"(w2951) -> ()
                                n2233 = local read "Limit Cluster"() -> (w2950:T1)
                                n2234 = Bundle By Name(cluster=w2950, "Lower Limit"=w2948) -> (w2949:T1)
                                n2235 = local write "Limit Cluster"(w2949) -> ()
                                }
                                frame 1 {
                                n2236 = local write "LoTable_2"(w2952) -> ()
                                }
                                }
                                }
                                frame 0 {
                                n2237 = Index Array(array=w2961, index=0) -> (element=w2960:T3)
                                n2238 = call "CRYDAT to Limit Curve.vi"("Data In"=w2960) -> ("Curve Out"=w2958:cluster{"x":dbl, "y":dbl}[])  [unwired: 10 out]
                                n2239 = call "CRYCurve to Table.vi"("y precision"=w2964, "x precision"=w2965, "Limit curve In"=w2958) -> ("Limit Table"=w2959:string[][])  [unwired: 1 in, 7 out]
                                n2240 = case shown="0, Default" w2962 {
                                tunnel: w2959 -> [w2969 w2970]
                                tunnel: w2958 -> [w2966 _]
                                frame 0, Default {
                                n2241 = local write "UpTable_1"(w2969) -> ()
                                n2242 = local read "Limit Cluster"() -> (w2967:T1)
                                n2243 = Bundle By Name(cluster=w2967, "Upper Limit"=w2966) -> (w2968:T1)
                                n2244 = local write "Limit Cluster"(w2968) -> ()
                                }
                                frame 1 {
                                n2245 = local write "UpTable_2"(w2970) -> ()
                                }
                                }
                                }
                                frame 1 {
                                n2246 = Index Array(array=w2977) -> (element=w2972:T3)  [unwired: 1 in]
                                n2247 = call "CRYDAT to Limit Curve.vi"("Data In"=w2972) -> ("Curve Out"=w2971:cluster{"x":dbl, "y":dbl}[])  [unwired: 10 out]
                                n2248 = call "CRYCurve to Table.vi"("y precision"=w2975, "x precision"=w2976, "Limit curve In"=w2971) -> ("Limit Table"=w2974:string[][])  [unwired: 1 in, 7 out]
                                n2249 = case shown="0, Default" w2973 {
                                tunnel: w2974 -> [w2981 w2982]
                                tunnel: w2971 -> [w2978 _]
                                frame 0, Default {
                                n2250 = local write "LoTable_1"(w2981) -> ()
                                n2251 = local read "Limit Cluster"() -> (w2979:T1)
                                n2252 = Bundle By Name(cluster=w2979, "Lower Limit"=w2978) -> (w2980:T1)
                                n2253 = local write "Limit Cluster"(w2980) -> ()
                                }
                                frame 1 {
                                n2254 = local write "LoTable_2"(w2982) -> ()
                                }
                                }
                                }
                                }
                                }
                                frame True {
                                }
                                }
                                n2255 = global write "CRYLimit edit global.vi" "Data"(w2886) -> ()
                                n2256 = call "CRYCurve to Table.vi"("y precision"=w2892, "Margin"=TRUE, "x precision"=w2891, "Limit curve In"=w2886) -> ("Limit Table"=w2890:string[][])  [unwired: 7 out]
                                n2257 = local write "Data Table"(w2890) -> ()
                              }
                              frame #1 {
                                n2258 = local write "Plot graphs"(TRUE ("Plot graphs")) -> ()
                              }
                            }
                          }
                          frame 2 {
                            n2259 = flat-sequence {
                              tunnel: w2991 -> [w3010]
                              tunnel: w2990 -> [w3009]
                              tunnel: w2989 -> [w3008]
                              tunnel: w2988 -> [w3007]
                              tunnel: w2987 -> [w2992]
                              tunnel: w2986 -> [w3006]
                              tunnel: w2985 -> [w2997]
                              tunnel: w2984 -> [w2993]
                              frame #0 {
                                n2260 = Equal?(x=w2997, y=u16 3) -> (x = y?=w3000:bool)
                                n2261 = Equal?(x=w2997, y=u16 5) -> (x = y?=w3001:bool)
                                n2262 = Or(x=w3000, y=w3001) -> (x .or. y?=w2995:bool)
                                n2263 = Select(t=u16 1 ("y"), s=w2995, f=u16 1 ("y")) -> (s? t:f=w2996:u16)
                                n2264 = case shown="False" w2995 {
                                tunnel: w2992 -> [_ w3017]
                                tunnel: [w3011 w3013] -> w2994
                                frame False {
                                n2265 = local read "Wave"() -> (w3012:T2)
                                n2266 = call "CRYWave Resolve Convert.vi"("Data Wave"=w3012) -> ("Curve Out"=w3011:cluster{dbl, dbl}[])  [unwired: 10 in]
                                }
                                frame True {
                                n2267 = Index Array(array=w3017, index=0) -> (element=w3014:T2)
                                n2268 = call "CRYWaveform to DAT.vi"("Waveform In"=w3014) -> ("Curve Out"=w3015:T3)  [unwired: 10 out]
                                n2269 = call "CRYDAT to Limit Curve.vi"("Data In"=w3015) -> ("Curve Out"=w3013:cluster{"x":dbl, "y":dbl}[])  [unwired: 10 out]
                                }
                                }
                                n2270 = Array Size(array=w2993) -> (size(s)=w3005:i32)
                                n2271 = Equal To 0?(x=w3005) -> (x = 0?=w3004:bool)
                                n2272 = case shown="False" w3004 {
                                tunnel: w3006 -> [w3024 _]
                                tunnel: w2993 -> [w3021 _]
                                tunnel: w3010 -> [w3023 _]
                                tunnel: w3009 -> [w3022 _]
                                tunnel: w3008 -> [w3020 _]
                                tunnel: w3007 -> [w3019 _]
                                tunnel: w2996 -> [w3018 _]
                                frame False {
                                n2273 = case shown="2, Default" w3024 {
                                tunnel: w3021 -> [w3037 w3049 w3059]
                                tunnel: w3023 -> [w3036 w3048 w3058]
                                tunnel: w3022 -> [w3035 w3047 w3057]
                                tunnel: w3020 -> [w3031 w3044 _]
                                tunnel: w3019 -> [w3030 _ w3054]
                                tunnel: w3018 -> [w3027 _ _]
                                frame 2, Default {
                                n2274 = Index Array(array=w3037, index=w3027) -> (element=w3028:T3)
                                n2275 = Index Array(array=w3037, index=0) -> (element=w3029:T3)
                                n2276 = call "CRYDAT to Limit Curve.vi"("Data In"=w3028) -> ("Curve Out"=w3026:cluster{"x":dbl, "y":dbl}[])  [unwired: 10 out]
                                n2277 = call "CRYDAT to Limit Curve.vi"("Data In"=w3029) -> ("Curve Out"=w3025:cluster{"x":dbl, "y":dbl}[])  [unwired: 10 out]
                                n2278 = call "CRYCurve to Table.vi"("y precision"=w3035, "x precision"=w3036, "Limit curve In"=w3026) -> ("Limit Table"=w3033:string[][])  [unwired: 1 in, 7 out]
                                n2279 = call "CRYCurve to Table.vi"("y precision"=w3035, "x precision"=w3036, "Limit curve In"=w3025) -> ("Limit Table"=w3032:string[][])  [unwired: 1 in, 7 out]
                                n2280 = case shown="1" w3030 {
                                tunnel: w3033 -> [w3038 w3039]
                                frame 0, Default {
                                n2281 = local write "LoTable_1"(w3038) -> ()
                                }
                                frame 1 {
                                n2282 = local write "LoTable_2"(w3039) -> ()
                                }
                                }
                                n2283 = case shown="0, Default" w3031 {
                                tunnel: w3032 -> [w3040 w3041]
                                frame 0, Default {
                                n2284 = local write "UpTable_1"(w3040) -> ()
                                }
                                frame 1 {
                                n2285 = local write "UpTable_2"(w3041) -> ()
                                }
                                }
                                }
                                frame 0 {
                                n2286 = Index Array(array=w3049, index=0) -> (element=w3043:T3)
                                n2287 = call "CRYDAT to Limit Curve.vi"("Data In"=w3043) -> ("Curve Out"=w3042:cluster{"x":dbl, "y":dbl}[])  [unwired: 10 out]
                                n2288 = call "CRYCurve to Table.vi"("y precision"=w3047, "x precision"=w3048, "Limit curve In"=w3042) -> ("Limit Table"=w3045:string[][])  [unwired: 1 in, 7 out]
                                n2289 = case shown="0, Default" w3044 {
                                tunnel: w3045 -> [w3050 w3051]
                                frame 0, Default {
                                n2290 = local write "UpTable_1"(w3050) -> ()
                                }
                                frame 1 {
                                n2291 = local write "UpTable_2"(w3051) -> ()
                                }
                                }
                                }
                                frame 1 {
                                n2292 = Index Array(array=w3059, index=0) -> (element=w3053:T3)
                                n2293 = call "CRYDAT to Limit Curve.vi"("Data In"=w3053) -> ("Curve Out"=w3052:cluster{"x":dbl, "y":dbl}[])  [unwired: 10 out]
                                n2294 = call "CRYCurve to Table.vi"("y precision"=w3057, "x precision"=w3058, "Limit curve In"=w3052) -> ("Limit Table"=w3055:string[][])  [unwired: 1 in, 7 out]
                                n2295 = case shown="0, Default" w3054 {
                                tunnel: w3055 -> [w3060 w3061]
                                frame 0, Default {
                                n2296 = local write "LoTable_1"(w3060) -> ()
                                }
                                frame 1 {
                                n2297 = local write "LoTable_2"(w3061) -> ()
                                }
                                }
                                }
                                }
                                }
                                frame True {
                                }
                                }
                                n2298 = global write "CRYLimit edit global.vi" "Data"(w2994) -> ()
                              }
                              frame #1 {
                                n2299 = local write "Plot graphs"(TRUE ("Plot graphs")) -> ()
                              }
                            }
                          }
                        }
                        n2300 = Unbundle By Name(w2860) -> ("Verdict"=→"Verdict":bool, "Margin"=w2841:dbl)
                        n2301 = stacked-sequence {
                          tunnel: w2841 -> [w2870 w2871]
                          frame #0 {
                            n2302 = local read "Y Resolution"() -> (w2869:u8)
                            n2303 = call "CRYRepresent numeric by precission.vi"("Pprecision"=w2869, "Numeric In"=w2870) -> ("Out Format"=w2868:string)  [unwired: 7 in, 2 out]
                            n2304 = property on="Margin" class="DigNum (strict)"("FormatString"=w2868) -> ()  [unwired: 2 in, 2 out]
                          }
                          frame #1 {
                            "Margin" <- w2871
                          }
                        }
                        n2305 = call "CRYGet Error Message.vi"("Kind"="Limits Sub") -> ("Unicode Message Sub"=w2846:string[])  [unwired: 5 in, 5 out]
                        n2306 = for {
                          tunnel: w2846 -> [w2875] mode=indexing
                          tunnel: [w2874] -> w2845 mode=indexing
                          n2307 = call "CRYConvert Unicode to ASCII.vi"("Unicode"=w2875) -> ("ASCII"=w2874:string)  [unwired: 4 in]
                        }
                        n2308 = Index Array(array=w2845, index=w2855) -> (element=w2854:string)
                        n2309 = Add(x=w2852, y=u16 9) -> (x+y=w2853:u16)
                        n2310 = property on="Margin" class="DigNum (strict)"("Caption.Text"=w2854) -> ()  [unwired: 2 in, 2 out]
                        n2311 = Index Array(array=w2845, index=w2853) -> (element=w2850:string)
                        n2312 = local write "tolerance"(w2850) -> ()
                        n2313 = flat-sequence {
                          tunnel: w2843 -> [_]
                          frame #0 {
                            n2314 = global read "CRYLimit edit global.vi" "ContinueF"() -> (w2872:bool)
                            n2315 = property on="Verdict" class="Bool (strict)"("Visible"=w2872) -> (error out=w2873:errorcluster)  [unwired: 2 in, 1 out]
                            n2316 = property on="Margin" class="DigNum (strict)"(error in=w2873, "Visible"=w2872) -> ()  [unwired: 1 in, 2 out]
                            n2317 = property on="tolerance" class="Str"("Visible"=w2872) -> ()  [unwired: 2 in, 2 out]
                          }
                        }
                      }
                      frame #1 {
                        w3070 = FALSE ("Visible")
                        n2318 = local read "Alignment"() -> (w3066:u16)
                        n2319 = property on="UpAlignRst_2" class="Str"("Visible"=w3070) -> ()  [unwired: 2 in, 2 out]
                        n2320 = property on="LowAlignRst_2" class="Str"("Visible"=w3070) -> ()  [unwired: 2 in, 2 out]
                        n2321 = property on="DataAlignRst" class="Str"("Visible"=w3070) -> ()  [unwired: 2 in, 2 out]
                        n2322 = property on="UpAlignRst_1" class="Str"("Visible"=w3070) -> ()  [unwired: 2 in, 2 out]
                        n2323 = property on="LowAlignRst_1" class="Str"("Visible"=w3070) -> ()  [unwired: 2 in, 2 out]
                        n2324 = disable-structure shown="Enabled" {
                          disable-tunnel: w3072 -> [w3097 w3100]
                          disable-tunnel: w3071 -> [w3096 w3099]
                          disable-tunnel: w3069 -> [_ w3098]
                          frame Disabled {
                            n2325 = call "CRYReplace Curve Name of Steps.vi"("New Name"=w3097, "Old Name"=w3096) -> ()  [unwired: 9 in, 1 out]
                          }
                          frame Enabled {
                            n2326 = call "CRYChange Name by Step Editor.vi"("Old Names Type"=w3098, "Old Names"=w3099, "New Names"=w3100) -> ()  [unwired: 9 in]
                          }
                        }
                        n2327 = global read "CRYLimit edit global.vi" "ContinueF"() -> (w3065:bool)
                        n2328 = Greater Or Equal?(x=w3066, y=u16 4) -> (x >= y?=w3067:bool)
                        n2329 = case shown="True" w3065 {
                          frame False {
                          }
                          frame True {
                            n2330 = local read "Type"() -> (w3073:u16)
                            n2331 = case shown="1, 2" w3073 {
                              frame 0, Default {
                              }
                              frame 1, 2 {
                                n2332 = local read "Alignment"() -> (w3074:u16)
                                n2333 = case shown="2, 4" w3074 {
                                frame 3, 5 {
                                n2334 = property on="DataAlignRst" class="Str"("Visible"=TRUE) -> ()  [unwired: 2 in, 2 out]
                                }
                                frame 2, 4 {
                                n2335 = local read "UpSource"() -> (w3077:u16)
                                n2336 = local read "LoSource"() -> (w3076:u16)
                                n2337 = case shown="0, Default" w3077 {
                                frame 0, Default {
                                n2338 = property on="UpAlignRst_1" class="Str"("Visible"=TRUE) -> ()  [unwired: 2 in, 2 out]
                                }
                                frame 1 {
                                n2339 = property on="UpAlignRst_2" class="Str"("Visible"=TRUE) -> ()  [unwired: 2 in, 2 out]
                                }
                                }
                                n2340 = case shown="1" w3076 {
                                frame 0, Default {
                                n2341 = property on="LowAlignRst_1" class="Str"("Visible"=TRUE) -> ()  [unwired: 2 in, 2 out]
                                }
                                frame 1 {
                                n2342 = property on="LowAlignRst_2" class="Str"("Visible"=TRUE) -> ()  [unwired: 2 in, 2 out]
                                }
                                }
                                }
                                frame Default {
                                }
                                }
                              }
                            }
                          }
                        }
                        n2343 = case shown="True" w3067 {
                          frame False {
                          }
                          frame True {
                            n2344 = global read "CRYLimit edit global.vi" "ContinueF"() -> (w3082:bool)
                            n2345 = case shown="False" w3082 {
                              frame False {
                                n2346 = global read "CRYLimit edit global.vi" "RoundOff"() -> (w3083:bool)
                                n2347 = case shown="True" w3083 {
                                frame False {
                                }
                                frame True {
                                w3084 = cluster{dbl, dbl} {0.0, 0.0} ("Align Ref")
                                n2348 = local read "Limit Cluster"() -> (w3088:T1)
                                n2349 = Bundle By Name(cluster=w3088, "Align Ref"=w3084) -> (w3087:T1)
                                n2350 = Unbundle(w3084) -> (w3086:dbl, w3085:dbl)
                                n2351 = local write "Limit Cluster"(w3087) -> ()
                                n2352 = local write "X AlignRef"(w3086) -> ()
                                n2353 = local write "Y AlignRef"(w3085) -> ()
                                }
                                }
                              }
                              frame True {
                                n2354 = global read "CRYLimit edit global.vi" "align ref point"() -> (w3090:cluster{dbl, dbl}[])
                                n2355 = Index Array(array=w3090, index=0) -> (element=w3089:cluster{dbl, dbl})
                                n2356 = local read "Limit Cluster"() -> (w3092:T1)
                                n2357 = Bundle By Name(cluster=w3092, "Align Ref"=w3089) -> (w3093:T1)
                                n2358 = Unbundle(w3089) -> (w3095:dbl, w3094:dbl)
                                n2359 = local write "Limit Cluster"(w3093) -> ()
                                n2360 = local write "X AlignRef"(w3095) -> ()
                                n2361 = local write "Y AlignRef"(w3094) -> ()
                              }
                            }
                          }
                        }
                      }
                    }
                  }
                }
              }
            }
          }
          frame "Operator", Default {
            n2362 = call "CRYGet Error Message.vi"("Kind"="Step Setup") -> ("Window Title"=w3102:string)  [unwired: 5 in, 5 out]
            n2363 = call "CRYGet Access Level Message.vi"() -> ("Multibyte string"=w3104:string)  [unwired: 11 in]
            n2364 = call "CRYMessage Dialog.vi"("Window Title"=w3102, "YesNoCancel"=T9."OK", "Message Content"=w3104) -> ()  [unwired: 7 in, 2 out]
          }
        }
      }
      frame 1 {
        # "Loading"
        n2365 = flat-sequence {
          tunnel: [w3117] -> w3105
          tunnel: w3105 -> [w3165]
          frame #0 {
            n2366 = local read "Limit Cluster"() -> (w3138:T1)
            n2367 = Unbundle By Name(w3138) -> ("X min-max-step"=w3145:T15, "X Axis"=w3135:u16, "Align Ref"=w3148:cluster{dbl, dbl}, "X-Resolution"=w3137:u8, "Y-Resolution"=w3136:u8, "Type"=w3117:u16, "Tolerance"=w3116:u16, "Limits"=w3114:u16, "x float"=w3134:bool, "magn/phase"=w3133:u16, "Upper Limit Type"=w3132:u16, "Lower Limit Type"=w3131:u16, "Lim Curve axis up"=w3130:u16, "Lim Curve axis lo"=w3129:u16, "Data Selection Upper"=w3126:u16, "Data Selection Lower"=w3125:u16, "Output failed point curves?"=w3128:bool, "Tab Value"=w3124:enum32{"Data", "Parameters"}, "Help"=w3127:string, "X Up Val"=w3113:dbl, "Y Up Val"=w3112:dbl, "X Low Val"=w3111:dbl, "Y Low Val"=w3110:dbl, "Up Limit Val"=w3108:dbl, "Low Limit Val"=w3109:dbl, "Custom Name"=w3107:string, "bAdd DataName"=w3106:bool)
            n2368 = local write "Mapping"(w3135) -> ()
            n2369 = Unbundle By Name(w3145) -> ("Limit X Offset Min"=w3144:dbl, "Limit X Offset Max"=w3143:dbl, "Limit X Offset Step Size"=w3142:dbl)
            n2370 = Unbundle(w3148) -> (w3147:dbl, w3146:dbl)
            n2371 = local write "Custom Name"(w3107) -> ()
            n2372 = local write "bAdd DataName"(w3106) -> ()
            n2373 = local write "X AlignRef"(w3147) -> ()
            n2374 = local write "Y AlignRef"(w3146) -> ()
            n2375 = local write "X Resolution"(w3137) -> ()
            n2376 = local write "Y Resolution"(w3136) -> ()
            n2377 = local write "Alignment"(w3116) -> ()
            n2378 = local write "Limits_Ring"(w3114) -> ()
            n2379 = local write "x float"(w3134) -> ()
            n2380 = local write "Data_xyz"(w3133) -> ()
            n2381 = local write "UpSource"(w3132) -> ()
            n2382 = local write "LoSource"(w3131) -> ()
            n2383 = local write "Up_xyz"(w3130) -> ()
            n2384 = local write "Lo_xyz"(w3129) -> ()
            n2385 = local write "Up_type"(w3126) -> ()
            n2386 = local write "Lo_type"(w3125) -> ()
            n2387 = local write "Out Fail"(w3128) -> ()
            n2388 = local write "Help"(w3127) -> ()
            n2389 = local write "X Up Val"(w3113) -> ()
            n2390 = local write "Y Up Val"(w3112) -> ()
            n2391 = local write "X Lo Val"(w3111) -> ()
            n2392 = local write "Y Lo Val"(w3110) -> ()
            n2393 = case shown="1, Default" w3135 {
              tunnel: w3144 -> [w3153 w3164]
              tunnel: [w3153 w3162] -> w3141
              tunnel: w3143 -> [w3152 w3159]
              tunnel: w3142 -> [w3151 w3158]
              tunnel: [w3151 w3155] -> w3139
              tunnel: [w3152 w3154] -> w3140
              frame 0 {
              }
              frame 1, Default {
                w3156 = 100.0
                w3157 = 1.0
                n2394 = Subtract(x=w3164, y=w3157) -> (x-y=w3163:dbl)
                n2395 = Subtract(x=w3159, y=w3157) -> (x-y=w3161:dbl)
                n2396 = Subtract(x=w3158, y=w3157) -> (x-y=w3160:dbl)
                n2397 = Multiply(x=w3156, y=w3163) -> (x*y=w3162:dbl)
                n2398 = Multiply(x=w3156, y=w3161) -> (x*y=w3154:dbl)
                n2399 = Multiply(x=w3156, y=w3160) -> (x*y=w3155:dbl)
              }
            }
            n2400 = property on="Main Tab" class="TabCtl (strict)"("Value"=w3124) -> ()  [unwired: 2 in, 2 out]
            n2401 = local write "RawLo Limit"(w3109) -> ()
            n2402 = local write "RawUp Limit"(w3108) -> ()
            n2403 = Equal?(x=w3117, y=u16 2) -> (x = y?=w3122:bool)
            n2404 = local write "Minimum"(w3141) -> ()
            n2405 = local write "Maximum"(w3140) -> ()
            n2406 = local write "Step Size"(w3139) -> ()
            n2407 = case shown="0, Default" w3114 {
              frame 0, Default {
                n2408 = local write "Plot index"(1 ("Plot index")) -> ()
              }
              frame 1 {
                n2409 = local write "Plot index"(2 ("Plot index")) -> ()
              }
            }
            n2410 = local write "Point index"(0 ("Point index")) -> ()
            n2411 = local write "Load state"(TRUE ("Load state")) -> ()
            n2412 = Select(t=u8 0 ("X Scale.Mapping Mode"), s=w3122, f=u8 1 ("X Scale.Mapping Mode")) -> (s? t:f=w3119:u8)
            n2413 = property on="Limits Graph" class="XYGraph (strict)"("XScale.Mapping Mode"=w3119) -> ()  [unwired: 2 in, 2 out]
          }
          frame #1 {
            n2414 = property on="Type" class="Slide (strict)"("Val(Sgnl)"=w3165) -> ()  [unwired: 2 in, 2 out]
          }
          frame #2 {
            n2415 = control-ref of="Board Tab"() -> (w3168:refnum<vi>)
            n2416 = control-ref of="This VI"() -> (w3166:refnum<vi>)
            n2417 = call "CRYAlign Steps VI Center.vi"("Tab2"=w3168, "Input/Output"=TRUE ("Preview"), "VIRef"=w3166) -> ()  [unwired: 1 in, 8 out]
          }
          frame #3 {
            n2418 = property on="Board Tab" class="TabCtl (strict)"("Visible"=TRUE) -> ()  [unwired: 2 in, 2 out]
            n2419 = local write "Load Test"(FALSE ("Load Test")) -> ()
          }
          frame #4 {
            n2420 = local read "AddStep"() -> (w3171:bool)
            n2421 = local write "Add Lib"(w3171) -> ()
          }
          frame #5 {
            n2422 = local write "AddStep"(FALSE ("AddStep")) -> ()
          }
        }
      }
      frame 2 {
        w3177 = u8 2 ("y")
        w3178 = u8 2 ("y")
        n2423 = property on="Limits Graph" class="XYGraph (strict)"() -> ("YScale.ScaleFit"=w3175:u8)  [unwired: 2 in, 2 out]
        n2424 = property on="Limits Graph" class="XYGraph (strict)"() -> ("XScale.ScaleFit"=w3179:u8)  [unwired: 2 in, 2 out]
        n2425 = local read "X Resolution"() -> (w3207:u8)
        n2426 = local read "Y Resolution"() -> (w3208:u8)
        n2427 = Equal?(x=w3179, y=w3178) -> (x = y?=w3181:bool)
        n2428 = Equal?(x=w3175, y=w3177) -> (x = y?=w3176:bool)
        n2429 = Select(t=w3179, s=w3181, f=w3178) -> (s? t:f=w3180:u8)
        n2430 = Select(t=w3175, s=w3176, f=w3177) -> (s? t:f=w3174:u8)
        n2431 = local read "LoSource"() -> (w3215:u16)
        n2432 = local read "Lo_type"() -> (w3214:enum32{"Single Values", "Curves", "Waveforms"})
        n2433 = property on="Limits Graph" class="XYGraph (strict)"("XScale.ScaleFit"=w3180) -> ()  [unwired: 2 in, 2 out]
        n2434 = local read "UpSource"() -> (w3221:u16)
        n2435 = local read "Up_type"() -> (w3223:enum32{"Single Values", "Curves", "Waveforms"})
        n2436 = property on="Limits Graph" class="XYGraph (strict)"("YScale.ScaleFit"=w3174) -> ()  [unwired: 2 in, 2 out]
        n2437 = Equal?(x=w3223, y=u16 2) -> (x = y?=w3220:bool)
        n2438 = Equal?(x=w3214, y=u16 2) -> (x = y?=w3213:bool)
        n2439 = Equal?(x=w3221, y=u16 1) -> (x = y?=w3218:bool)
        n2440 = Equal?(x=w3215, y=u16 1) -> (x = y?=w3211:bool)
        n2441 = And(x=w3218, y=w3220) -> (x .and. y?=w3219:bool)
        n2442 = And(x=w3211, y=w3213) -> (x .and. y?=w3212:bool)
        n2443 = local write "Plot graphs"(FALSE ("Plot graphs")) -> ()
        n2444 = case shown="False" w3212 {
          tunnel: w3211 -> [w3259 _]
          tunnel: w3207 -> [_ w3263]
          tunnel: w3208 -> [_ w3262]
          tunnel: [w3255 w3261] -> w3209
          frame False {
            n2445 = local read "LoTable_1"() -> (w3258:string[][])
            n2446 = local read "LoTable_2"() -> (w3260:string[][])
            n2447 = call "CRYTable Empty Ignore.vi"("Table In"=w3258) -> ("Table Out"=w3257:string[][])  [unwired: 10 in]
            n2448 = Select(t=w3260, s=w3259, f=w3257) -> (s? t:f=w3256:string[][])
            n2449 = call "CRYTable to Curve.vi"("Table In"=w3256) -> ("Limit curve"=w3255:cluster{"Numeric":dbl, "Numeric 2":dbl}[])  [unwired: 10 in]
          }
          frame True {
            n2450 = local read "Lo Wave"() -> (w3264:T2)
            n2451 = call "CRYWave Resolve Convert.vi"("Y Resolution"=w3262, "X Resolution"=w3263, "Data Wave"=w3264) -> ("Curve Out"=w3261:cluster{dbl, dbl}[])  [unwired: 8 in]
          }
        }
        n2452 = case shown="True" w3219 {
          tunnel: w3218 -> [w3269 _]
          tunnel: w3207 -> [_ w3273]
          tunnel: w3208 -> [_ w3272]
          tunnel: [w3265 w3271] -> w3210
          frame False {
            n2453 = local read "UpTable_1"() -> (w3268:string[][])
            n2454 = local read "UpTable_2"() -> (w3270:string[][])
            n2455 = call "CRYTable Empty Ignore.vi"("Table In"=w3268) -> ("Table Out"=w3267:string[][])  [unwired: 10 in]
            n2456 = Select(t=w3270, s=w3269, f=w3267) -> (s? t:f=w3266:string[][])
            n2457 = call "CRYTable to Curve.vi"("Table In"=w3266) -> ("Limit curve"=w3265:cluster{"Numeric":dbl, "Numeric 2":dbl}[])  [unwired: 10 in]
          }
          frame True {
            n2458 = local read "Up Wave"() -> (w3274:T2)
            n2459 = call "CRYWave Resolve Convert.vi"("Y Resolution"=w3272, "X Resolution"=w3273, "Data Wave"=w3274) -> ("Curve Out"=w3271:cluster{dbl, dbl}[])  [unwired: 8 in]
          }
        }
        n2460 = global read "CRYLimit edit global.vi" "critical point"() -> (w3206:cluster{dbl, dbl}[])
        n2461 = global read "CRYLimit edit global.vi" "align ref point"() -> (w3205:cluster{dbl, dbl}[])
        n2462 = global read "CRYLimit edit global.vi" "Upper Failed"() -> (w3204:cluster{dbl, dbl}[])
        n2463 = global read "CRYLimit edit global.vi" "Lower Failed"() -> (w3203:cluster{dbl, dbl}[])
        n2464 = local read "Limits_Ring"() -> (w3200:u16)
        n2465 = local read "Out Fail"() -> (w3195:bool)
        n2466 = local read "Alignment"() -> (w3192:u16)
        n2467 = case shown="0, Default" w3200 {
          tunnel: [TRUE ("Plot.Visible") FALSE ("Plot.Visible") w3254] -> w3199
          tunnel: [FALSE ("Plot.Visible") TRUE ("Plot.Visible") w3254] -> w3198
          tunnel: w3195 -> [w3237 w3246 w3253]
          tunnel: [w3236 w3245 w3253] -> w3194
          tunnel: [w3235 w3244 w3253] -> w3193
          frame 0, Default {
            n2468 = case shown="False" w3237 {
              tunnel: [FALSE ("Plot.Visible") TRUE ("Plot.Visible")] -> w3236
              tunnel: [FALSE ("Plot.Visible") FALSE ("Plot.Visible")] -> w3235
              frame False {
              }
              frame True {
              }
            }
          }
          frame 1 {
            n2469 = case shown="False" w3246 {
              tunnel: [FALSE ("Plot.Visible") FALSE ("Plot.Visible")] -> w3245
              tunnel: [FALSE ("Plot.Visible") TRUE ("Plot.Visible")] -> w3244
              frame False {
              }
              frame True {
              }
            }
          }
          frame 2 {
            w3254 = TRUE ("Plot.Visible")
          }
        }
        n2470 = global read "CRYLimit edit global.vi" "Data"() -> (w3183:cluster{"x":dbl, "y":dbl}[])
        n2471 = Equal?(x=w3192, y=u16 4) -> (x = y?=w3191:bool)
        n2472 = Equal?(x=w3192, y=u16 5) -> (x = y?=w3190:bool)
        n2473 = Or(x=w3191, y=w3190) -> (x .or. y?=w3186:bool)
        n2474 = Build Cluster Array(w3183, w3210, w3209, w3206, w3205, w3204, w3203) -> (w3173:T18)
        n2475 = disable-structure shown="Disabled" {
          frame Disabled {
            n2476 = local read "Data Table"() -> (w3234:string[][])
            n2477 = call "CRYTable to Curve.vi"("Table In"=w3234) -> ()  [unwired: 10 in, 1 out]
          }
          frame Enabled {
          }
        }
        n2478 = property on="Limits Graph" class="XYGraph (strict)"("Value"=w3173, "XScale.Precision"=w3207, "YScale.Precision"=w3208, "Active Plot"=u32 1, "Plot.Visible?"=w3199, "Active Plot"=u32 2, "Plot.Visible?"=w3198, "Active Plot"=u32 0, "Plot.Visible?"=TRUE ("Plot.Visible"), "Active Plot"=u32 5, "Plot.Visible?"=w3194, "Active Plot"=u32 6, "Plot.Visible?"=w3193, "Active Plot"=u32 4, "Plot.Visible?"=w3186) -> (error out=w3182:errorcluster)  [unwired: 2 in, 1 out]
        n2479 = disable-structure shown="Disabled" {
          disable-tunnel: w3173 -> [w3228 _]
          frame Disabled {
            n2480 = local read "Plot index"() -> (w3226:i32)
            n2481 = local read "Point index"() -> (w3227:i32)
            n2482 = Index Array(array=w3228, index=w3226) -> (element=w3230:T19)
            n2483 = Unbundle(w3230) -> ("Lower Failed"=w3231:cluster{"Numeric":dbl, "Numeric 2":dbl}[])
            n2484 = Index Array(array=w3231, index=w3227) -> (element=w3229:cluster{"Numeric":dbl, "Numeric 2":dbl})
            n2485 = property on="Limits Graph" class="XYGraph (strict)"("Cursor.Cursor Position"=w3229) -> ()  [unwired: 2 in, 2 out]
          }
          frame Enabled {
          }
        }
        n2486 = flat-sequence {
          tunnel: w3182 -> [_]
          frame #0 {
            n2487 = control-ref of="Limits Graph"() -> (w3233:refnum<vi>)
            n2488 = call "CRYPaint WaterMark.vi"("Type"="Small", "Graph Ref"=w3233) -> ()  [unwired: 10 in]
          }
        }
      }
      frame 3 {
        # "MultiLimit"
        n2489 = local read "UpSource"() -> (w3284:u16)
        n2490 = local read "LoSource"() -> (w3283:u16)
        n2491 = local read "Up Limit Val"() -> (w3280:dbl)
        n2492 = local read "Lo Limit Val"() -> (w3277:dbl)
        n2493 = local read "UpSingleVal"() -> (w3279:dbl)
        n2494 = local read "LoSingleVal"() -> (w3276:dbl)
        n2495 = Equal To 0?(x=w3284) -> (x = 0?=w3282:bool)
        n2496 = Equal To 0?(x=w3283) -> (x = 0?=w3281:bool)
        n2497 = Select(t=w3280, s=w3282, f=w3279) -> (s? t:f=w3278:dbl)
        n2498 = Select(t=w3277, s=w3281, f=w3276) -> (s? t:f=w3275:dbl)
        n2499 = local read "Limits_Ring"() -> (w3290:u16)
        n2500 = local read "Multi value"() -> (w3286:dbl)
        n2501 = control-ref of="Single Limit"() -> (w3293:refnum<vi>)
        n2502 = control-ref of="Multi Limit"() -> (w3295:refnum<vi>)
        n2503 = control-ref of="Multi value"() -> (w3294:refnum<vi>)
        n2504 = local read "Type"() -> (w3289:u16)
        n2505 = local write "Plot Multilimit"(FALSE ("Plot Multilimit")) -> ()
        n2506 = Equal To 0?(x=w3289) -> (x = 0?=w3288:bool)
        n2507 = Select(t=w3286, s=w3288, f=0.0) -> (s? t:f=w3285:dbl)
        n2508 = call "CRYMultimeter Scale Change.vi"("Limits"=w3290, "Multi Val"=w3285, "Single Limit"=w3293, "Low Limit"=w3275, "Up Limit"=w3278, "Multi value"=w3294, "Multi limit"=w3295) -> ("Lo tip"=w3291:cluster{dbl, dbl}, "Up tip"=w3292:cluster{dbl, dbl})  [unwired: 2 in, 1 out]
        n2509 = property on="Up tip" class="Str"("Position"=w3292) -> ()  [unwired: 2 in, 2 out]
        n2510 = property on="Lo tip" class="Str"("Position"=w3291) -> ()  [unwired: 2 in, 2 out]
      }
      frame 4 {
        # "Add Lib"
        n2511 = flat-sequence {
          tunnel: [w3306] -> w3303
          tunnel: [w3305] -> w3302
          tunnel: [w3304] -> w3297
          tunnel: w3303 -> [w3313]
          tunnel: [w3315] -> w3301
          tunnel: w3302 -> [w3315]
          tunnel: [w3314] -> w3300
          tunnel: [w3312] -> w3298
          tunnel: w3297 -> [w3312]
          tunnel: w3301 -> [w3321]
          tunnel: w3300 -> [w3320]
          tunnel: [w3319] -> w3299
          tunnel: w3298 -> [w3319]
          tunnel: w3299 -> [w3322]
          frame #0 {
            n2512 = local read "Proper VI No"() -> (w3304:i32)
            n2513 = local read "Limit Cluster"() -> (w3307:T1)
            n2514 = Build Array(w3304) -> (w3309:i32[])
            n2515 = call "CRYFlatten Limits.vi"("Limits"=w3307) -> ("Flatten Limits String"=w3306:string)  [unwired: 10 in]
            n2516 = call "CRYGet Curve Library Data Name.vi"("nData"=w3309, "sAction"="GetNamebyStep" ("sOption")) -> ("sNames"=w3305:string[])  [unwired: 6 in, 3 out]
          }
          frame #1 {
            n2517 = call "CRYGet Current TS Steps.vi"() -> ("SelectStepNumber in Tree"=w3317:i32, "Steps"=w3318:T7[])  [unwired: 1 in, 9 out]
            n2518 = Index Array(array=w3318, index=w3317) -> (element=w3311:T7)
            n2519 = Unbundle By Name(w3311) -> ("StepName"=w3310:string)
            n2520 = call "CRYLimit Curves Name Replace.vi"("StepName"=w3310, "Setup in"=w3311, "Step Set up In"=w3313, "Type In"="AddStep" ("t")) -> ("Inserted Names Out"=w3314:string[])  [unwired: 7 in]
          }
          frame #2 {
            n2521 = call "CRYReplace Curve Name of Steps.vi"("New Name"=w3320, "Old Name"=w3321) -> ()  [unwired: 9 in, 1 out]
          }
          frame #3 {
            n2522 = global read "CRYStepSetup Global.vi" "Load from AddStep"() -> (w3323:bool)
            n2523 = case shown="True" w3323 {
              tunnel: w3322 -> [_ w3326]
              frame False {
              }
              frame True {
                n2524 = global write "CRYStepSetup Global.vi" "Load from AddStep"(FALSE ("Load from AddStep")) -> ()
                n2525 = call "CRYStepData Manipulate.vi"("sAction"="Backup", "StepNo."=w3326) -> ()  [unwired: 10 in]
              }
            }
            n2526 = local write "Add Lib"(FALSE ("Add Lib")) -> ()
          }
        }
      }
      frame 5 {
        n2527 = flat-sequence {
          frame #0 {
            n2528 = global read "CRYMainGlobal.vi" "Access Level"() -> (w3329:enum16{"Engineer", "Technician", "Operator"})
            n2529 = case shown="\"Engineer\"" w3329 {
              frame "Engineer" {
                n2530 = flat-sequence {
                  tunnel: [w3335] -> w3333
                  tunnel: [w3340] -> w3332
                  tunnel: w3333 -> [w3347]
                  tunnel: [w3346] -> w3330
                  tunnel: w3332 -> [w3346]
                  tunnel: [w3345] -> w3331
                  tunnel: w3331 -> [w3351]
                  tunnel: w3330 -> [w3352]
                  frame #0 {
                    n2531 = local read "Limit Cluster"() -> (w3336:T1)
                    n2532 = local read "Proper VI No"() -> (w3334:i32)
                    n2533 = call "CRYFlatten Limits.vi"("Limits"=w3336) -> ("Flatten Limits String"=w3335:string)  [unwired: 10 out]
                    n2534 = Build Array(w3334) -> (w3342:i32[])
                    n2535 = call "CRYGet Curve Library Data Name.vi"("nData"=w3342, "sAction"="GetNamebyStep" ("sOption")) -> ("sNames"=w3340:string[])  [unwired: 6 in, 3 out]
                    n2536 = call "CRYPreUpdate Sequence.vi"("EventName"="SequenceUpdate", "Proper VI No"=w3334, "Project View Step Name Identifier Arg1"="", "Step flattened Arg2"=w3335, "AllChangeFlg"=TRUE ("Name/Identifier")) -> ()  [unwired: 11 in]
                  }
                  frame #1 {
                    n2537 = call "CRYGet Current TS Steps.vi"() -> ("SelectStepNumber in Tree"=w3349:i32, "Steps"=w3350:T7[])  [unwired: 1 in, 9 out]
                    n2538 = Index Array(array=w3350, index=w3349) -> (element=w3344:T7)
                    n2539 = Unbundle By Name(w3344) -> ("StepName"=w3343:string)
                    n2540 = call "CRYLimit Curves Name Replace.vi"("StepName"=w3343, "Setup in"=w3344, "Step Set up In"=w3347, "Type In"="StepOK" ("t")) -> ("Inserted Names Out"=w3345:string[])  [unwired: 7 in]
                  }
                  frame #2 {
                    n2541 = call "CRYReplace Curve Name of Steps.vi"("New Name"=w3351, "Old Name"=w3352) -> ()  [unwired: 9 in, 1 out]
                  }
                }
              }
              frame "Technician", Default {
                n2542 = call "CRYGet Error Message.vi"("Kind"="Step Setup") -> ("Window Title"=w3355:string)  [unwired: 5 in, 5 out]
                n2543 = call "CRYGet Access Level Message.vi"("sAction"="OK") -> ("Multibyte string"=w3357:string)  [unwired: 10 in]
                n2544 = call "CRYMessage Dialog.vi"("Window Title"=w3355, "YesNoCancel"=T9."OK", "Message Content"=w3357) -> ()  [unwired: 7 in, 2 out]
              }
            }
          }
          frame #1 {
            n2545 = local write "OK"(FALSE ("OK")) -> ()
          }
        }
        n2546 = local write "stop"(TRUE ("stop")) -> ()
      }
      frame 6 {
        n2547 = flat-sequence {
          frame #0 {
            n2548 = local read "Proper VI No"() -> (w3360:i32)
            n2549 = call "CRYStepData Manipulate.vi"("sAction"="Restore", "StepNo."=w3360) -> ()  [unwired: 10 in]
          }
          frame #1 {
            n2550 = local write "Cancel"(FALSE ("Cancel")) -> ()
          }
        }
        n2551 = local write "stop"(TRUE ("stop")) -> ()
      }
    }
    n2552 = global read "CRYMain Sub Window Global.vi" "gStop"() -> (w80:bool)
    n2553 = Or(x=w80, y="stop") -> (x .or. y?=w79:bool)
  }
  n2554 = flat-sequence {
    tunnel: w2 -> [_]
    frame #0 {
      n2555 = control-ref of="This VI"() -> (w3363:refnum<vi>)
      n2556 = call "CRYWork Before Step Close.vi"("StepVI Ref"=w3363) -> ()  [unwired: 11 in]
    }
    frame #1 {
      n2557 = local write "EndFlag"(TRUE ("EndFlag")) -> ()
    }
  }
